vi "ControlProgram6.6_4.vi"() -> ()   [LabVIEW 2016]
uses:
  <vilib>/Utility/miscctls.llb/LVPoint32TypeDef.ctl
  <vilib>/Platform/TimedLoop/XDataNode/timing_clust.ctl
  <vilib>/Platform/TimedLoop/XDataNode/nitl_modes.ctl
  <vilib>/Platform/TimedLoop/XDataNode/wakeup.ctl
  <vilib>/Instr/_visa.llb/Select Event Type.ctl
  <vilib>/vision/Avi1.llb/AviRefnum.ctl
  <vilib>/Utility/error.llb/DialogType.ctl
  <vilib>/DAQmx/write.llb/DAQmx Write (Analog 1D DBL NChan 1Samp).vi
  <vilib>/DAQmx/read.llb/DAQmx Read (Analog 2D DBL NChan NSamp).vi
  <vilib>/Analysis/baseanly.llb/Mean (DBL).vi
  <vilib>/DAQmx/write.llb/DAQmx Write (Digital Bool 1Line 1Point).vi
  <vilib>/DAQmx/create/channels.llb/DAQmx Create Channel (DO-Digital Output).vi
  <vilib>/DAQmx/create/channels.llb/DAQmx Create Channel (AI-Voltage-Basic).vi
  <vilib>/DAQmx/create/channels.llb/DAQmx Create Channel (AO-Voltage-Basic).vi
  <vilib>/DAQmx/configure/timing.llb/DAQmx Timing (Sample Clock).vi
  <vilib>/DAQmx/miscellaneous.llb/DAQmx Fill In Error Info.vi
  <vilib>/Instr/_visa.llb/VISA Configure Serial Port (Instr).vi
  Arnulf--joystick/git(most_up_to_date)/Logitech-joystick/Old Trap/FAST_Global_var.vi
  <vilib>/Utility/inputDevices.llb/mouseAcquire.vi
  <vilib>/Utility/inputDevices.llb/closeMouse.vi
  <vilib>/platform/TimedLoop/XDataNode/XDataNode.xnode
  <vilib>/Platform/TimedLoop/XDataNode/XDNodeRunTimeDep.lvlib
  <resource>/objmgr/daqmx.rc
  <vilib>/Analysis/NI_AALBase.lvlib
panel:
  in  "Save file index":i32
  out "Saving Move":bool
  out "Move time":string
  out "Primary Video Display":T1(plugin-control)
  out "Flush Sample Start Time":u32=2111292881
  out "Sample flush time (s)":dbl=48.0
  in  "Inject Sample":bool
  out "Cal values":T2={"AX alpha"=612.9626061060078, "BX alpha"=549.6584469744151, "AX kappa"=0.3485731373010688, "BX kappa"=0.3853424216291352, "AX offset"=-0.03900484438240665, "BX offset"=-0.11295550662085417, "AY alpha"=582.7562541114835, "BY alpha"=571.1587543790358, "AY kappa"=0.37498408087930674, "BY kappa"=0.36252029651198364, "AY offset"=-0.21125584642206058, "BY offset"=-0.12469077200400738}
  in  "Inject Pump 1":bool
  in  "Inject Pump 2":bool
  in  "Tab Control 2":T3(tab)
  in  "Force FB script":bool
  in  "Got ADig bead":bool
  in  "Move Cap. 2 (ADig Top)":bool
  in  "Dump beads":bool
  in  "Got DNA bead":bool
  in  "Flow on\ncap 2?":bool=TRUE
  in  "Flow on\ncap 1?":bool=TRUE
  in  "Flow on\ndump?":bool=TRUE
  in  "Raster set":i32=1
  in  "Fish After TA?":bool=TRUE
  in  "Delta after tether":dbl=1700.0
  in  "TA Cancel Save?":bool=TRUE
  in  "Min fish\ndelta (nm)":dbl=1425.0 min=0.0 max=5000.0 step=50.0
  in  "Max fish\ndelta (nm)":dbl=1900.0 min=0.0 max=5000.0 step=25.0
  in  "Fish Speed (ms)":i32=5000
  in  "Wait (ms)":i32=1500
  in  "# attempts":dbl=10.0
  in  "Cutoff force (pN)":dbl=4.5
  in  "Raster after\n tether?":bool=TRUE
  out "Tether":bool
  out "Attempt #":i32
  in  "Flow on\nwhile fish?":bool=TRUE
  in  "Flow on\nafter raster?":bool=TRUE
  in  "Offset raster set":i32
  in  "Offset @ Delta (nm)":dbl=1700.0
  in  "Cal @ Delta (nm)":dbl=2500.0
  in  "Cal stage position":i32=3
  out "Cal Final Sampling Rate":dbl=125000.0
  in  "Cal Averaging":i32=1
  in  "Wait before dip (s)":dbl=3.0
  in  "Start dipping after?":bool
  in  "Start trap delta (nm)":dbl=1700.0
  in  "Repeat Dip":bool
  out "Dip #":i32
  in  "Dip attempts":dbl=3.0
  in  "Cancel Rep\n Dip":bool
  out "Return elasped time":i32
  in  "Return duration":dbl=15.0
  in  "Cancel dwell":bool=TRUE
  in  "Pause dwell":bool
  in  "Start/Return position":dbl=3.0
  in  "Dip duration":dbl=15.0
  in  "Dip position":dbl=4.0
  in  "Dip":bool
  out "Dip elasped time":i32
  in  "Stop":bool=TRUE
  in  "?":T4(tab)
  out "FAST X-Y":bool
  out "FAST Z":bool
  in  "Cal time (s)":dbl=5.0
  in  "Save N sets":bool
  in  "N sets":i32=200
  out "Cal sets to save":i32=500
  in  "Reset data stream":bool
  out "Buffer Overflow":bool
  out "Stage moving":bool
  in  "Comment":string
  in  "Raster scan":bool
  out "Saving":bool
  in  "Save cal":bool
  in  "Save Data":bool
  in  "Stop saving":bool
  out "Calibrating":bool
  out "Progress":dbl(slide) scale=0.0..100.0
  in  "Read Cal":bool
  in  "Fish":bool
  in  "Averaging Number":i32=1250
  out "Final Sampling Rate":dbl=100.0
  in  "Trap position (V)":cluster{"X":dbl, "Y":dbl}={"X"=3.9042624789680316, "Y"=0.2}
  in  "Trap delta (nm)":dbl=2500.0 min=0.0 max=5000.0 step=50.0
  in  "Fixed X":dbl=1.1
  in  "Fixed Y":dbl=0.15
  in  "Shutter 1 (B)":bool
  in  "Shutter 2 (A)":bool
  in  "Pulling direction":bool
  out "Raster scanning...":bool
  out "Current file name":path=path "D:/data/160111/160111_006.dat"
  in  "AX alpha":dbl=612.9626061060078 format="%#_3p"
  in  "BX alpha":dbl=549.6584469744151 format="%#_3g"
  in  "AX kappa":dbl=0.3485731373010688 format="%#_3g"
  in  "BX kappa":dbl=0.3853424216291352 format="%#_3g"
  in  "AX offset":dbl=-0.03900484438240665 format="%#_3g"
  in  "BX offset":dbl=-0.11295550662085417 format="%#_3g"
  in  "AY alpha":dbl=582.7562541114835 format="%#_3g"
  in  "BY alpha":dbl=571.1587543790358 format="%#_3g"
  in  "AY kappa":dbl=0.37498408087930674 format="%#_3g"
  in  "BY kappa":dbl=0.36252029651198364 format="%#_3g"
  in  "AY offset":dbl=-0.21125584642206058 format="%#_3g"
  in  "BY offset":dbl=-0.12469077200400738 format="%#_3g"
  out "Buffer status":u8(slide) scale=0.0..100.0
  in  "Target":bool
  in  "Set Current\nPos to (0,0,0)":bool
  in  "dump spot":string="Dump beads spot"
  in  "up flow spot":string="Upper flow spot"
  in  "low flow spot":string="Lower flow spot"
  in  "up cap":string="Upper capillary (ADig beads)"
  in  "bottom cap":string="Lower capillary (DNA beads)"
  in  "Move to Position 5":bool
  in  "Set Position 5":bool
  in  "Saved stage positions":dbl[][](array[numeric])=[[1.0, 0.0, 0.0, 0.0], [2.0, -0.13716, -3.21132, 0.01436], [3.0, 0.45, -0.73974, 0.005], [4.0, 0.45, -2.1978, 0.005], [5.0, 0.45, -2.63158, -0.02256]]
  in  "Set Position 2":bool
  in  "Move to Position 2":bool
  in  "Set Position 1":bool
  in  "Move to Position 1":bool
  in  "Set Position 4":bool
  in  "Move to Position 4":bool
  in  "Set Position 3":bool
  in  "Move to Position 3":bool
  out "Stage error":errorcluster
  in  "Clear Volume":bool
  out "Sample Flush Meter":u8(slide) scale=0.0..100.0
  out "Flushing Sample":bool
  in  "Flush Sample":bool
  in  "Normal \nRate (ul/hr)  3":dbl=100.0
  in  "Normal \nVolume (ul) 3":dbl=250.0
  in  "Normal \nVolume (ul) 2":dbl
  in  "Normal \nRate (ul/hr)":dbl
  in  "Normal \nVolume (ul)":dbl
  in  "Flush\nRate (ul/min)":dbl
  in  "Flush\nVolume (ul)":dbl
  in  "Flush \nRate (ul/min)  2":dbl
  in  "Flush Pump 2":bool
  in  "Flush\nVolume (ul)  2":dbl
  in  "Flush Pump 1":bool
  in  "Normal \nRate (ul/hr)  2":dbl
  in  "Write Wait":i32=1000
  in  "Flush \nRate (ul/min)  3":dbl=100.0
  in  "Flush\nVolume (ul)  3":dbl=80.0
  out "error out":errorcluster
  in  "Use Mouse to Move Trap?":bool
  in  "Pause Mouse/Mirror Connection":bool
  out "Reference Voltage":cluster{dbl, dbl}={0.0, -0.0}
  out "Saved voltage":cluster{dbl, dbl}={5.766666666666665, 1.45}
  out "Real Coordinates":cluster{"Horizontal":i32, "Vertical":i32}={"Horizontal"=897, "Vertical"=-1271}
  out "CoordinatesMousePressed":T5
  in  "Force Feedback 2":bool
  in  "Offset 2":cluster{"Off Y":dbl, "Off X":dbl}={"Off Y"=1.5, "Off X"=0.17}
  in  "Setpoint voltage 2":cluster{"SP Y":dbl, "SP X":dbl}={"SP Y"=0.6, "SP X"=0.0}
  out "Sum error":dbl(knob) scale=-0.2..0.2
  out "Trap sep":waveform(dbl)[](graph)=[{"t0"=timestamp(4.489999999999949 s since 1904-01-01), "dt"=0.002, "Y"=[-1157.7639781743756, -1157.678951177374, -1157.7582331070425, -1157.7490409992681, -1157.8995617642552], "attributes"=variant("NI_ChannelName"=variant(string "T2 X"))}, {"t0"=timestamp(4.489999999999949 s since 1904-01-01), "dt"=0.002, "Y"=[-909.0775466981794, -909.1316439023619, -909.1322956759037, -909.1570630705896, -909.1264297140281], "attributes"=variant("NI_ChannelName"=variant(string "T2 Y"))}]
  in  "Set reading to\nsetpoint 1":bool
  in  "Offset Y (nm)":dbl format="%0.2f"
  in  "Offset X (nm)":dbl format="%0.2f"
  in  "Remove offsets":bool
  in  "Force Feedback 1":bool
  out "Feedback Output \nVoltage 2":cluster{dbl, dbl} {"?" format="%#_4g"; "?" format="%#_4g"}
  in  "Offset 1":cluster{"Off Y":dbl, "Off X":dbl}={"Off Y"=1.5, "Off X"=0.17}
  in  "Setpoint voltage 1":cluster{"SP Y":dbl, "SP X":dbl}={"SP Y"=0.6, "SP X"=0.0}
  in  "Feedback const":T6={"Ki_B_Y"=0.5, "Ki_B_X"=0.0, "Kp Y"=1.0, "Kp X"=0.0}
  out "Mean Trap Pos X 2 (nm)":dbl=-1157.769953044463 format="%0.2f"
  out "Mean Trp Pos Y 2 (nm)":dbl=-909.1249958122125 format="%0.2f"
  out "T2 X RMS (A)":dbl=0.7168002469275427 format="%0.2f"
  out "T2 Y RMS (A)":dbl=0.25997187037503383 format="%0.2f"
  in  "Set reading to\nsetpoint 2":bool
  in  "Scan range (nm)":dbl=425.0
  in  "Scan speed (nm/s)":dbl=100.0 min=0.0 max=100.0
  in  "Step size (nm)":dbl=1.0
  in  "Save scans":bool=TRUE
  in  "# scans":i32=1
  in  "Load param":bool
  in  "Scan Parameters":T7(array[cluster])
  in  "Trap delta\nafter (nm)":dbl=1550.0
  in  "Stop raster":bool
  out "Scan range (V)":dbl=0.47672462142456534
  out "Scan steps (mirror)":u64=425
  out "Scan increment (V)":dbl=0.0011217049915872126
  out "Time per step (ms)":dbl=10.0
  out "Total raster time (s)":dbl=8.5
  out "N sets to be saved":dbl=850.0
  in  "Zoom Factor":sgl=7.0
  in  "Center Point":cluster{"X":i32, "Y":i32}={"X"=335, "Y"=271}
  in  "Intensity Upper":dbl=88.0
  in  "Intensity Lower":dbl=66.0
  out "Window Size":cluster{"Height":i32, "Width":i32}
  in  "Image Index":dbl=1.0 min=1.0
  in  "Save Image":bool
  in  "Averaging":bool
  in  "Reset Averaging":bool
  in  "Save Video":bool
  in  "New Video File":bool
  in  "Video Index":dbl=1.0 min=1.0 step=1.0
  in  "Video Capture Rate (Hz)":dbl=30.0
  in  "Initial Window Size":cluster{"Width":i32, "Height":i32}={"Width"=884, "Height"=619}
  in  "Initial Window Position":cluster{"X Position":i32, "Y Position":i32}={"X Position"=796, "Y Position"=4}
  out "Window Position":cluster{"X Position":i32, "Y Position":i32}={"X Position"=40, "Y Position"=40}
  out "Path Out":path
  in  "Target coordinates":cluster{"X1":dbl, "Y1":dbl, "X2":dbl, "Y2":dbl}={"X1"=328.0, "Y1"=274.0, "X2"=368.0, "Y2"=314.0}
  in  "# Samples/channel (in)":i32=40000 format="%.2f"
  out "Buffer size\n(Samples/channel)":u32=511
  out "DAQ rate\n(Samples/s)":dbl=125000.0 format="%#_6p"
  out "# Samples/channel":i32=1250
  out "# Samples/channel/s":dbl=100.0
  out "AvailSampPerChan":u32=9
  out "Data update period (s/set)":dbl=0.01 format="%#_6p"
  out "AvailSampPerChan 2":u32=110
  in  "PC samp per channel":i32=1000
  in  "Sampling Rate":dbl=125000.0 format="%0.0p"
  in  "DAQ Rate2":dbl=1000000.0 format="%#_6p"
  out "Data period (s)":dbl=8e-06 format="%#_6p"
  in  "Save user params":bool
  in  "User":string(combo)
  in  "Load user params":bool
  in  "Tether break\nforce (pN)":dbl=1.0
  in  "Path":path=path "E:/Data"
  out "Mirror task":refnum<k21>
  in  "Conv X (nm/V)":dbl=891.5
  in  "Conv Y (nm/V)":dbl=505.7
  in  "Min value Y":dbl format="%.1g"
  in  "Max value Y":dbl=10.0 format="%.1f"
  in  "Min value X":dbl format="%0.1f"
  in  "Max value X":dbl=10.0 format="%.1f"
  in  "HWP1":string="Half waveplate 1: differential trap power"
  in  "HWP0":string="Half waveplate 0: total trap power"
  in  "Move 1":bool
  in  "\"Degrees\" 1":dbl
  in  "Move 0":bool
  in  "\"Degrees\" 0":dbl
  in  "Y command":enum16{"Fish", "Dump", "Got ADig", "Got DNA"}(ring)
  in  "B command":enum16{"Got DNA", "Got ADig", "Dump", "Fish"}(ring)
  in  "A command":enum16{"Got ADig", "Dump", "Fish", "Got DNA"}(ring)
  in  "X command":enum16{"Dump", "Fish", "Got ADig", "Got DNA"}(ring)
  out "Logitech":bool
  out "START":bool
  out "BACK":bool
  out "Right stick button":bool
  out "Left Y":i8(slide) scale=-128.0..127.0
  out "Left X":i8(slide) scale=-128.0..127.0
  out "Right Y":i8(slide) scale=-128.0..127.0
  out "Right X":i8(slide) scale=-128.0..127.0
  out "X":bool
  out "Y":bool
  out "A":bool
  out "B":bool
  out "RB":bool
  out "LB":bool
  out "R":bool
  out "L":bool
  out "D":bool
  out "U":bool
  out "Left stick button":bool
  out "FAST Z":bool
  out "FAST X-Y":bool
  in  "XY Speed Definitions":T8={"Slow X velocity input"="0.05", "Slow Y velocity input"="0.05", "Fast1 X velocity input"="0.1", "Fast1 Y velocity input"="0.1", "Fast2 X velocity input"="0.2", "Fast2 Y velocity input"="0.2"}
  in  "Z Speed Definitions":cluster{"Slow Z":string, "Fast Z":string}={"Slow Z"="0.025", "Fast Z"="0.05"}
  in  "Z Wait time":string="120"
  in  "X-Y Wait time":string="125"
  in  "USB port":refnum<visa-resource-name>="USB0::0x046D::0xC21D::CC66247B::RAW"
  out "Deflection":T5
  in  "Sampling Rate":dbl=125000.0 format="%0.2f"
  in  "Averaging Number":i32=12500
  in  "DAQ Rate":dbl=1000000.0
  out "Final Sampling Rate":dbl
  in  "Tab Control":T9(tab)
  in  "Downsamp\nfact":dbl=250.0
  out "Bead sep":waveform(dbl)[](graph)=[{"t0"=timestamp(4.489999999999949 s since 1904-01-01), "dt"=0.002, "Y"=[8093.963535945606, 8103.1617772716045, 8385.72390184118, 8245.733099167523, 8154.925676756515], "attributes"=variant("NI_ChannelName"=variant(string "T2"))}, {"t0"=timestamp(4.489999999999949 s since 1904-01-01), "dt"=0.002, "Y"=[1717.924930434114, 1628.723007842151, 1787.6888378897193, 1598.475730715916, 1776.2517588078954], "attributes"=variant("NI_ChannelName"=variant(string "T1"))}]
  out "Force (pN)":waveform(dbl)[](graph)=[{"t0"=timestamp(4.489999999999949 s since 1904-01-01), "dt"=0.002, "Y"=[2821.5994183803123, 2824.8226375853515, 2923.3663028678166, 2874.5254578927593, 2842.869034836209], "attributes"=variant("NI_ChannelName"=variant(string "T2"))}, {"t0"=timestamp(4.489999999999949 s since 1904-01-01), "dt"=0.002, "Y"=[623.5850847499229, 591.0680427774053, 648.761979867749, 579.944408346982, 644.7436619059413], "attributes"=variant("NI_ChannelName"=variant(string "T1"))}]
  out "Mean force (pN)":dbl=1737.5286029210451 format="%0.2f"
  out "Force noise (pN)":dbl=26.83032703631318 format="%0.2f"
  out "Mean Bead Sep\n(nm)":dbl=4949.257225667222 format="%0.2f"
  out "Bead Sep Noise\n(A)":dbl=757.8078481959694 format="%0.2f"
  out "PSD 2":cluster{dbl[], dbl[]}(graph)
  out "PSD 1":cluster{dbl[], dbl[]}(graph)
  out "PSD 1 Sum":dbl(slide) scale=0.0..10.0
  out "PSD 2 Sum":dbl(slide) scale=0.0..10.0
  in  "Start":bool
  out "All signals 2":waveform(dbl)[](graph)=[{"t0"=timestamp(4.489999999999949 s since 1904-01-01), "dt"=0.002, "Y"=[0.0010396217068286443, 0.0010666908927528754, 0.001103298744846499, 0.0010651440823993424, 0.0010656596859401936], "attributes"=variant("NI_ChannelName"=variant(string "A y"))}, {"t0"=timestamp(4.489999999999949 s since 1904-01-01), "dt"=0.002, "Y"=[0.02000680227246931, 0.020097032918054827, 0.02003412926844257, 0.020136734401221615, 0.020087494249822452], "attributes"=variant("NI_ChannelName"=variant(string "A x"))}, {"t0"=timestamp(4.489999999999949 s since 1904-01-01), "dt"=0.002, "Y"=[-0.0014958587831537804, -0.0015046240440107857, -0.0014930229638311983, -0.001533240041751485, -0.0015262793936602433], "attributes"=variant("NI_ChannelName"=variant(string "B y"))}, {"t0"=timestamp(4.489999999999949 s since 1904-01-01), "dt"=0.002, "Y"=[0.0002901198559372817, 0.0002731049385577592, 0.00026511308349727467, 0.0002517073909711183, 0.0002916666665966012], "attributes"=variant("NI_ChannelName"=variant(string "B x"))}, {"t0"=timestamp(4.489999999999949 s since 1904-01-01), "dt"=0.002, "Y"=[-0.001511556786147372, -0.0015167122027053212, -0.0014612914746018214, -0.0014935128282145193, -0.0015064013696263116], "attributes"=variant("NI_ChannelName"=variant(string "A sum"))}, {"t0"=timestamp(4.489999999999949 s since 1904-01-01), "dt"=0.002, "Y"=[-0.0005242945138364382, -0.0005565158674093218, -0.000501095139248956, -0.0005771375336978897, -0.0005165613890095197], "attributes"=variant("NI_ChannelName"=variant(string "B sum"))}, {"t0"=timestamp(4.489999999999949 s since 1904-01-01), "dt"=0.002, "Y"=[0.0013303666019343777, 0.0014257418088905328, 0.0013368108726387405, 0.0013471217058124534, 0.0011782818123890176], "attributes"=variant("NI_ChannelName"=variant(string "Trap x"))}, {"t0"=timestamp(4.489999999999949 s since 1904-01-01), "dt"=0.002, "Y"=[0.0023382505474007294, 0.002231275652833831, 0.002229986798687363, 0.0021810103409340116, 0.002241586486003531], "attributes"=variant("NI_ChannelName"=variant(string "Trap y"))}]
  out "All signals":waveform(dbl)[](graph)=[{"t0"=timestamp(4.489999999999949 s since 1904-01-01), "dt"=0.002, "Y"=[0.0010396217068286443, 0.0010666908927528754, 0.001103298744846499, 0.0010651440823993424, 0.0010656596859401936], "attributes"=variant("NI_ChannelName"=variant(string "A y"))}, {"t0"=timestamp(4.489999999999949 s since 1904-01-01), "dt"=0.002, "Y"=[0.02000680227246931, 0.020097032918054827, 0.02003412926844257, 0.020136734401221615, 0.020087494249822452], "attributes"=variant("NI_ChannelName"=variant(string "A x"))}, {"t0"=timestamp(4.489999999999949 s since 1904-01-01), "dt"=0.002, "Y"=[-0.0014958587831537804, -0.0015046240440107857, -0.0014930229638311983, -0.001533240041751485, -0.0015262793936602433], "attributes"=variant("NI_ChannelName"=variant(string "B y"))}, {"t0"=timestamp(4.489999999999949 s since 1904-01-01), "dt"=0.002, "Y"=[0.0002901198559372817, 0.0002731049385577592, 0.00026511308349727467, 0.0002517073909711183, 0.0002916666665966012], "attributes"=variant("NI_ChannelName"=variant(string "B x"))}, {"t0"=timestamp(4.489999999999949 s since 1904-01-01), "dt"=0.002, "Y"=[-0.001511556786147372, -0.0015167122027053212, -0.0014612914746018214, -0.0014935128282145193, -0.0015064013696263116], "attributes"=variant("NI_ChannelName"=variant(string "A sum"))}, {"t0"=timestamp(4.489999999999949 s since 1904-01-01), "dt"=0.002, "Y"=[-0.0005242945138364382, -0.0005565158674093218, -0.000501095139248956, -0.0005771375336978897, -0.0005165613890095197], "attributes"=variant("NI_ChannelName"=variant(string "B sum"))}, {"t0"=timestamp(4.489999999999949 s since 1904-01-01), "dt"=0.002, "Y"=[0.0013303666019343777, 0.0014257418088905328, 0.0013368108726387405, 0.0013471217058124534, 0.0011782818123890176], "attributes"=variant("NI_ChannelName"=variant(string "Trap x"))}, {"t0"=timestamp(4.489999999999949 s since 1904-01-01), "dt"=0.002, "Y"=[0.0023382505474007294, 0.002231275652833831, 0.002229986798687363, 0.0021810103409340116, 0.002241586486003531], "attributes"=variant("NI_ChannelName"=variant(string "Trap y"))}]
  out "Chart Freq (Hz)":dbl=500.0
  # "Bead Calibration"
  # "Y"
  # "X"
  # "Pump #1 Controls"
  # "Pump #2 Controls"
  # "Sample Pump Controls"
  # "Retract the pumps manually. Change it back to INFUSE when you're done. Suck it up, don't whine."
  # "Shutter 1 (B)"
  # "Move to Lower Cap"
  # "Inject Sample"
  # "Move to Upper Cap"
  # "Shutter 2 (A)"
  # "Select the Joystick input:"
  # "Overflow happens when >40 commands\nsent in 5 seconds. Then 4 consecutive beeps."
  # "Try increasing wait time to reduce 'following error threshold exceeded' occurances."
  # "Left stick controls Z axis.\nRight on stick: neg Z-dir\nUp on stick: neg Z-dir"
  # "Toggles FAST Z"
  # "Toggles FAST X-Y"
  # "The default Newport max velocity is 0.4"
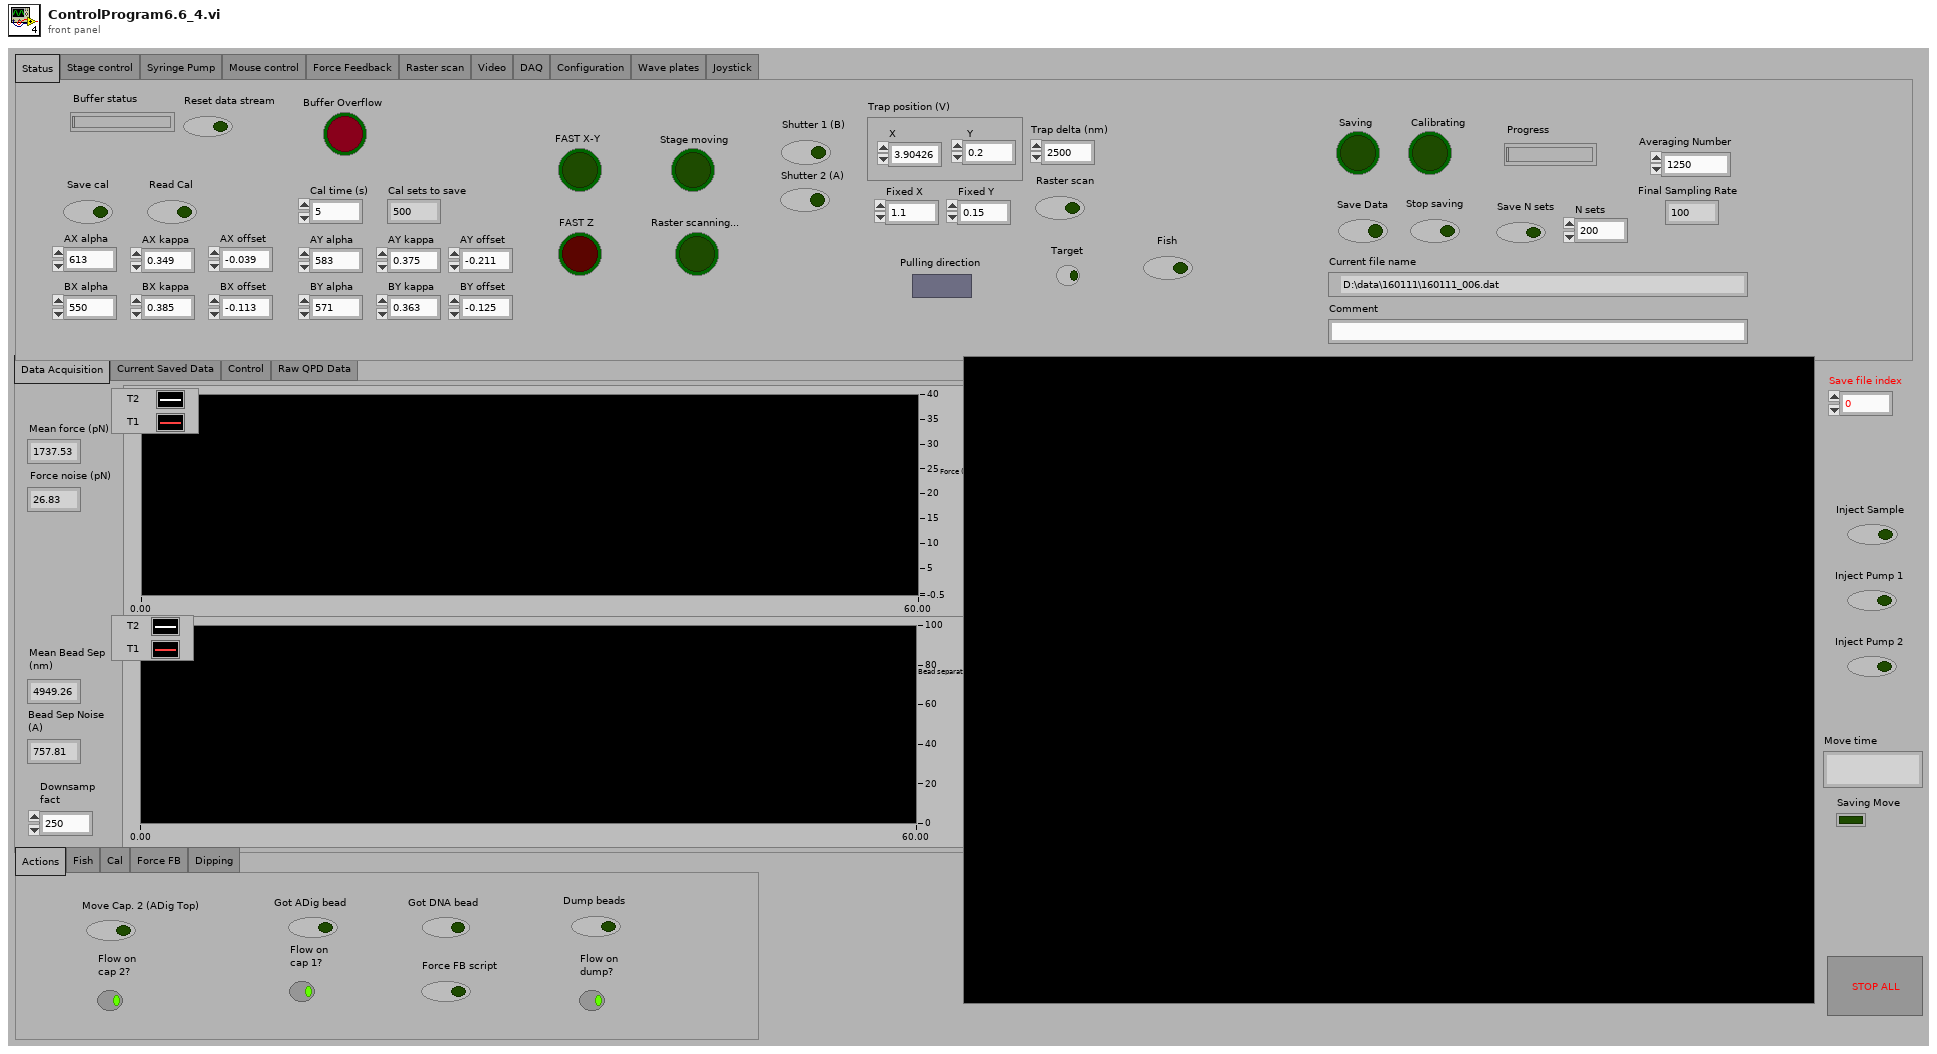
[diagram p1: front panel]
types:
  T1 = typedef "IMAQ Image.ctl" = refnum<image>
  T2 = cluster{"AX alpha":dbl, "BX alpha":dbl, "AX kappa":dbl, "BX kappa":dbl, "AX offset":dbl, "BX offset":dbl, "AY alpha":dbl, "BY alpha":dbl, "AY kappa":dbl, "BY kappa":dbl, "AY offset":dbl, "BY offset":dbl}
  T3 = enum32{"Actions", "Fish", "Cal", "Force FB", "Dipping"}
  T4 = enum32{"Status", "Stage control", "Syringe Pump", "Mouse control", "Force Feedback", "Raster scan", "Video", "DAQ", "Configuration", "Wave plates", "Joystick"}
  T5 = typedef "LVPoint32TypeDef.ctl" = cluster{"Horizontal":i32, "Vertical":i32}
  T6 = cluster{"Ki_B_Y":dbl, "Ki_B_X":dbl, "Kp Y":dbl, "Kp X":dbl}
  T7 = cluster{"Label":string, "Scan range 1":dbl, "Step size 1":dbl, "Scan speed 1":i32, "# scans 2":i32}[]
  T8 = cluster{"Slow X velocity input":string, "Slow Y velocity input":string, "Fast1 X velocity input":string, "Fast1 Y velocity input":string, "Fast2 X velocity input":string, "Fast2 Y velocity input":string}
  T9 = enum32{"Data Acquisition", "Current Saved Data", "Control", "Raw QPD Data"}
  T10 = typedef "Select Event Type.ctl" = u32
  T11 = enum32{"setting", "request", "request control", "info", "statistics", "system settings", "I/O sub system", "HRT control", "camera descriptions", "device specific data", "event sub system settings", "event sub system results", "image memory manager"}
  T12 = typedef "AviRefnum.ctl" = refnum<k1>
  T13 = typedef "XDNodeRunTimeDep.lvlib/timing_clust.ctl" = cluster{"Expected End [f-1]":u64, "Actual End [f-1]":u64, "Finished Late? [f-1]":bool, "Expected End [i-1]":u64, "Actual End [i-1]":u64, "Finished Late? [i-1]":bool, "Expected Start [i]":u64, "Actual Start [i]":u64, "Expected Start [f]":u64, "Actual Start [f]":u64, "Source Name":string, "Structure Name":string, "Period":i64, "Deadline":i64, "Offset":i64, "Start":i64, "Priority":i32, "Timeout":i32, "Mode":T14, "Wakeup Reason":T15, "Error":errorcluster, "Source Type":string, "Secondary Source Type":string, "Global End Time":u64, "Global Start Time":u64, "Frame Duration":u64, "Iteration Duration":u64, "Assigned CPU":i32, "I/O Scan Engine Mode":u32}
  T14 = typedef "XDNodeRunTimeDep.lvlib/nitl_modes.ctl" = enum32{"No Change", "Process missed periods, maintain original phase", "Discard missed periods, maintain original phase", "Process missed periods, ignore original phase", "Discard missed periods, ignore original phase"}
  T15 = typedef "XDNodeRunTimeDep.lvlib/wakeup.ctl" = enum32{"Normal", "Aborted", "Asynchronous wakeup", "Timing source error", "Timed loop error", "Timeout"}
  T16 = typedef "Image Type" = u32
  T17 = typedef "imagedata.ctl" = cluster{"image type":i32, "image depth":i32, "image":u8[], "mask":u8[], "colors":u32[], "Rectangle":cluster{"left":i16, "top":i16, "right":i16, "bottom":i16}}
  T18 = enum16{"open", "replace", "create", "open or create", "replace or create", "replace or create with confirmation"}
  T19 = enum16{"big-endian, network order", "native, host order", "little-endian"}
  T20 = cluster{string, string, string, string, string, string, string, string}
  T21 = cluster{"LB":bool, "RB":bool, "BACK":bool, "Logitech":bool, "START":bool}
  T22 = cluster{"Right X":i8, "Right Y":i8, "Left X":i8, "Left Y":i8}
  T23 = enum32{"Status", "Stage control", "Syringe Pump", "Mouse control", "Force Feedback", "Raster scan", "Video", "DAQ", "Configuration", "Wave plates"}
  T24 = typedef "DialogType.ctl" = u16
  T25 = cluster{"button 1":bool, "button 2":bool, "button 3":bool, "button 4":bool}
  T26 = cluster{"[0]":dbl, "[1]":dbl, "[2]":dbl, "[3]":dbl, "[4]":dbl, "[5]":dbl, "[6]":dbl, "[7]":dbl, "[8]":dbl, "[9]":dbl, "[10]":dbl, "[11]":dbl}
  T27 = cluster{"Label":string, "Scan range 1":dbl, "Step size 1":dbl, "Scan speed 1":i32, "# scans 2":i32}
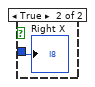
[diagram p5: hidden frame]
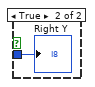
[diagram p6: hidden frame]
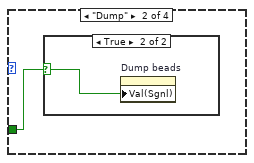
[diagram p10: hidden frame]
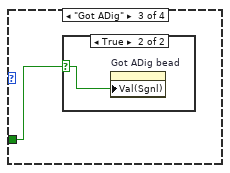
[diagram p12: hidden frame]
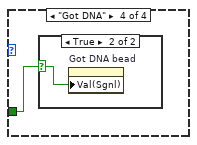
[diagram p14: hidden frame]
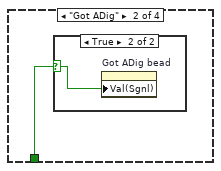
[diagram p17: hidden frame]
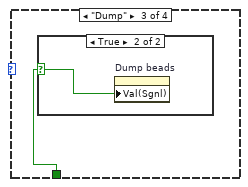
[diagram p19: hidden frame]
diagram:
  w10 = T10 1073684535 items=["Service Request"=1073684491, "Trigger"=3221168138, "Clear"=1073684493, "VXI Signal"=1073684512, "VXI/VME Interrupt"=3221168161, "VXI/VME Sysfail"=1073684509, "VXI/VME Sysreset"=1073684510, "GPIB CIC"=1073684498, "GPIB Talk"=1073684499, "GPIB Listen"=1073684500, "PXI Interrupt"=1073684514, "Serial Break"=1073684515, "Serial TermChar"=1073684516, "Serial CTS"=1073684521, "Serial DSR"=1073684522, "Serial DCD"=1073684524, "Serial RI"=1073684526, "Serial Character"=1073684533, "USB Interrupt"=1073684535, "All Enabled"=1073709055] ("Event Type")
  w49 = 10.0 ("Minimum Value")
  w50 = -10.0 ("Minimum Value")
  w52 = -2.0 ("Minimum Value")
  w53 = 2.0 ("Maximum Value")
  w78 = 10123 items=["Finite Samples"=10178, "Continuous Samples"=10123] ("sample mode")
  w98 = tag "Dev1/port2/line1"  # Shutter 2
  w101 = tag "Dev1/port1/line4"  # Shutter 1
  # "Open the RAW resource"
  # "Enable USB Interrupt Event"
  # "Create channels for movable mirror"
  # "Create channels for detectors"
  n1 = call-poly <vilib>:"DAQmx Create Virtual Channel.vi"("maximum value"=w53, "minimum value"=w52, "physical channels"=tag "Dev1/ai0" ("Physical Channel")) -> ("task out"=w54:refnum<k21>, "error out"=w77:errorcluster)  [unwired: 11 in]
  n2 = call-poly <vilib>:"DAQmx Create Virtual Channel.vi"("task in"=w54, "maximum value"=w53, "minimum value"=w52, "physical channels"=tag "Dev1/ai1", "error in"=w77) -> ("task out"=w75:refnum<k21>, "error out"=w74:errorcluster)  [unwired: 9 in]
  n3 = call-poly <vilib>:"DAQmx Create Virtual Channel.vi"("task in"=w75, "maximum value"=w53, "minimum value"=w52, "physical channels"=tag "Dev1/ai2", "error in"=w74) -> ("task out"=w66:refnum<k21>, "error out"=w65:errorcluster)  [unwired: 9 in]
  n4 = call-poly <vilib>:"DAQmx Create Virtual Channel.vi"("task in"=w66, "maximum value"=w53, "minimum value"=w52, "physical channels"=tag "Dev1/ai3" ("Physical Channel"), "error in"=w65) -> ("task out"=w51:refnum<k21>, "error out"=w71:errorcluster)  [unwired: 9 in]
  n5 = call-poly <vilib>:"DAQmx Create Virtual Channel.vi"("task in"=w51, "maximum value"=w49, "minimum value"=w50, "physical channels"=tag "Dev1/ai4", "error in"=w71) -> ("task out"=w69:refnum<k21>, "error out"=w68:errorcluster)  [unwired: 9 in]
  n6 = call-poly <vilib>:"DAQmx Create Virtual Channel.vi"("task in"=w69, "maximum value"=w49, "minimum value"=w50, "physical channels"=tag "Dev1/ai5", "error in"=w68) -> ("task out"=w64:refnum<k21>, "error out"=w63:errorcluster)  [unwired: 9 in]
  n7 = call-poly <vilib>:"DAQmx Create Virtual Channel.vi"("task in"=w64, "maximum value"=w49, "minimum value"=w50, "physical channels"=tag "Dev1/ai6", "error in"=w63) -> ("task out"=w58:refnum<k21>, "error out"=w56:errorcluster)  [unwired: 9 in]
  n8 = call-poly <vilib>:"DAQmx Create Virtual Channel.vi"("task in"=w58, "maximum value"=w49, "minimum value"=w50, "physical channels"=tag "Dev1/ai7", "error in"=w56) -> ("task out"=w57:refnum<k21>, "error out"=w55:errorcluster)  [unwired: 9 in]
  n9 = call-poly <vilib>:"DAQmx Timing.vi"("task/channels in"=w57, "sample mode"=w78, "samples per channel"="PC samp per channel", "rate"="Sampling Rate", "error in"=w55) -> ("task out"=w61:refnum<k21>, "error out"=w60:errorcluster)  [unwired: 9 in]
  n10 = call-poly <vilib>:"DAQmx Create Virtual Channel.vi"("maximum value"="Max value Y", "minimum value"="Min value Y", "physical channels"=tag "Dev1/ao1" ("Trap X Axis")) -> ("task out"=w46:refnum<k21>, "error out"=w48:errorcluster)  [unwired: 11 in]
  n11 = property class="DAQmx Timing"(reference=w61, error in=w60, "More:AI Convert:Rate"="DAQ Rate2") -> (reference out=w19:refnum<k21>, error out=w18:errorcluster, "SampClk.Rate"=→"DAQ rate\n(Samples/s)":dbl)
  n12 = call-poly <vilib>:"DAQmx Create Virtual Channel.vi"("task in"=w46, "maximum value"="Max value X", "minimum value"="Min value X", "physical channels"=tag "Dev1/ao0" ("Trap Y Axis"), "error in"=w48) -> ("task out"=w37:refnum<k21>, "error out"=w36:errorcluster)  [unwired: 9 in]
  "Mirror task" <- w37
  n13 = property class="DAQmx Buffer"(reference=w19, error in=w18) -> (reference out=w16:refnum<k21>, error out=w15:errorcluster, "Input.OnbrdBufSize"=→"Buffer size\n(Samples/channel)":u32)
  n14 = call <vilib>:"DAQmx Start Task.vi"("task/channels in"=w16, "error in"=w15) -> ("task out"=w38:refnum<k21>)  [unwired: 12 in, 1 out]
  n15 = flat-sequence "Video" {
    tunnel: [w114] -> w13
    tunnel: w13 -> [w155]
    frame #0 {
      n16 = while {
        stop <- w107 continue-if-true
        n17 = call "Close Video Capture.vi"() -> ("error code OUT"=w109:i32)
        n18 = Equal?(x=w109, y=0) -> (x = y?=w107:bool)
      }
      n19 = local write "Stop"(FALSE ("Stop All")) -> ()
    }
    frame #1 {
      n20 = call "DMR_Init.vi"() -> ()  [unwired: 3 out]
    }
    frame #2 {
      # "Setting the destination format to Mono8 makes sure that the image can be displayed in the intensity plot."
      n21 = call "DMR_GetDevice.vi"("search string IN"="DE514724602") -> ("device handle OUT"=w132:i32)  [unwired: 4 in, 2 out]
      n22 = call "DMR_OpenDevice.vi"("device handle IN"=w132) -> ("driver handle OUT"=w115:i32)  [unwired: 4 out]
      n23 = call "DMR_FindList.vi"("flags IN"=u32 0 ("flags"), "list name IN"="" ("String"), "list type IN"=T11."camera descriptions", "driver handle IN"=w115) -> ("list handle OUT"=w118:i32)  [unwired: 2 out]
      n24 = call "DMR_FindList.vi"("flags IN"=u32 0 ("flags"), "list name IN"="Base", "list type IN"=T11."setting", "driver handle IN"=w115) -> ("list handle OUT"=w116:i32)  [unwired: 2 out]
      n25 = call "OBJ_GetHandle.vi"("object name IN"="VideoStandard", "list handle IN"=w118) -> ("object handle OUT"=w112:i32)  [unwired: 3 out]
      n26 = call "OBJ_GetHandle.vi"("object name IN"="PixelFormat", "list handle IN"=w116) -> ("object handle OUT"=w126:i32)  [unwired: 3 out]
      n27 = call "OBJ_SetS.vi"("value index IN"=0, "value IN"="NTSC M", "object handle IN"=w112) -> ()  [unwired: 2 out]
      n28 = call "OBJ_SetS.vi"("value index IN"=0, "value IN"="Mono8" ("value"), "object handle IN"=w126) -> ()  [unwired: 2 out]
      n29 = call "OBJ_GetHandle.vi"("object name IN"="VideoChannel", "list handle IN"=w116) -> ("object handle OUT"=w122:i32)  [unwired: 3 out]
      n30 = while {
        tunnel: [w137] -> w114
        tunnel: w115 -> [w134]
        stop <- w135 continue-if-true
        n31 = call "DMR_ImageRequestSingle.vi"("request control IN"=0, "driver handle IN"=w134) -> ("error code OUT"=w136:i32, "driver handle OUT"=w137:i32)  [unwired: 2 out]
        n32 = Equal To 0?(x=w136) -> (x = 0?=w135:bool)
      }
      n33 = call "OBJ_SetI.vi"("value index IN"=0, "value IN"=0 ("Video channel"), "object handle IN"=w122) -> ()  [unwired: 2 out]
    }
    frame #3 {
      w143 = T16 0 items=["Grayscale (U8)", "Grayscale (I16)", "Grayscale (SGL)", "Complex (CSG)", "RGB (U32)", "HSL (U32)", "RGB (U64)"] ("Image Type")
      w151 = T16 0 items=["Grayscale (U8)", "Grayscale (I16)", "Grayscale (SGL)", "Complex (CSG)", "RGB (U32)", "HSL (U32)", "RGB (U64)"] ("Image Type")
      n34 = for "Create Greyscale map" {
        N: 256 -> [_]
        tunnel: [w157] -> w140 mode=indexing
        workers-P: _ -> [_]
        i -> [w160]
        n35 = To Unsigned Byte Integer(number=w160) -> (unsigned 8bit integer=w156:u8)
        n36 = Join Numbers(hi=w156, lo=w156) -> ((hi.lo)=w159:u16)
        n37 = Join Numbers(hi=w156, lo=w156) -> ((hi.lo)=w158:u16)
        n38 = Join Numbers(hi=w159, lo=w158) -> ((hi.lo)=w157:u32)
      }
      n39 = call "IMAQ Create"("Image Name"="Scaled video", "Image Type"=w143) -> ("New Image"=w142:T1)  [unwired: 2 in, 2 out]
      n40 = call "IMAQ Create"("Image Name"="Main video", "Image Type"=w151) -> ("New Image"=w152:T1)  [unwired: 2 in, 2 out]
      n41 = node-c288(0 ("Processor")) -> (w150:T13)  [unwired: 3 out]
      n42 = Initialize Array(u32 0 ("Window Number (0...15)"), 480 ("dimension size"), 640 ("dimension size")) -> (w145:u32[][])
      n43 = timed-loop {
        tunnel: w155 -> [w177]
        tunnel: [w176] -> w154
        tunnel: w152 -> [w175]
        timing: w150 -> [_]
        timing-out: [_] -> w149
        tunnel: w145 -> [w164]
        tunnel: w142 -> [w162]
        tunnel: w140 -> [w161]
        stop <- w163 stop-if-true
        # "This block performs the \nactual image capture."
        n44 = node-c288() -> ()  [unwired: 2 out]
        n45 = local read "Stop"() -> (w163:bool)
        n46 = Reciprocal(x="Video Capture Rate (Hz)") -> (1/x=w167:dbl)
        n47 = Multiply(x=w167, y=1000.0) -> (x*y=w165:dbl)
        n48 = call "DMR_ImageRequestWaitFor.vi"("queue number IN"=0, "timeout(ms) IN"=500, "driver handle IN"=w177) -> ("error code OUT"=w181:i32, "request number OUT"=w178:i32, "driver handle OUT"=w179:i32)
        n49 = feedback #1(T12 refnum ("Avi Refnum")) -> (w169:T12)
        n50 = case shown="True" "New Video File" {
          tunnel: [T12 refnum ("Avi Refnum") w198] -> w171
          tunnel: [FALSE TRUE] -> w172
          tunnel: w169 -> [_ w194]
          frame False {
          }
          frame True {
            n51 = call "Create new save file.vi"("Ext"=".avi" ("string"), "Index In"="Video Index") -> ("Path Out"=w190:path, "Index Out"=w191:dbl)  [unwired: 1 in]
            "Path Out" <- w190
            n52 = Not Equal?(x=w194, y=T12 refnum ("Avi Refnum")) -> (x != y?=w195:bool)
            n53 = Increment(x=w191) -> (x+1=w200:dbl)
            n54 = case shown="True" w195 {
              tunnel: w194 -> [_ w201]
              frame False {
              }
              frame True {
                n55 = call "IMAQ AVI Close"("Avi Refnum"=w201) -> ()  [unwired: 1 in, 10 out]
              }
            }
            n56 = local write "Video Index"(w200) -> ()
            n57 = call "IMAQ AVI Create"("Frames Per Second"=u32 30, "AVI Path"=w190) -> ("Avi Refnum"=w198:T12)  [unwired: 5 in, 4 out]
          }
        }
        n58 = Equal To 0?(x=w181) -> (x = 0?=w180:bool)
        n59 = Select(t=w171, s=w172, f=w169) -> (s? t:f=w170:T12)
        n60 = feedback-in #1(w170) -> ()
        n61 = case shown="True" w180 {
          tunnel: w179 -> [w202 w229]
          tunnel: w178 -> [_ w228]
          tunnel: [w202 w225] -> w176
          tunnel: w175 -> [_ w206]
          tunnel: w164 -> [_ w213]
          tunnel: w170 -> [_ w211]
          tunnel: w162 -> [_ w207]
          tunnel: w161 -> [_ w208]
          frame False {
          }
          frame True {
            w219 = u32 0 ("X-offset IN")
            n62 = call "DMR_GetImageRequestBufferData.vi"("driver handle IN"=w229, "request number IN"=w228) -> ("width OUT"=w218:i32, "height OUT"=w217:i32, "driver handle OUT"=w224:i32, "request number OUT"=w223:i32, "bytes per pixel OUT"=w220:i32)  [unwired: 13 out]
            n63 = call "DMR_GetImageRequestBufferImageData.vi"("driver handle IN"=w224, "request number IN"=w223, "bytes per pixel IN"=w220, "X-offset IN"=w219, "Y-offset IN"=w219, "height IN"=w217, "width IN"=w218) -> ("driver handle OUT"=w222:u32, "request number OUT"=w221:u32, "image OUT"=w214:u32[][])  [unwired: 10 out]
            n64 = call "DMR_ImageRequestUnlock.vi"("request number IN"=w221, "driver handle IN"=w222) -> ("driver handle OUT"=w227:i32)  [unwired: 1 in, 2 out]
            n65 = case shown="False" "Averaging" {
              tunnel: w214 -> [w270 w275]
              tunnel: [w270 w274] -> w210
              tunnel: w213 -> [_ w272]
              frame False {
              }
              frame True {
                (unwired) 1
                w280 = 1
                n66 = feedback #2(w272) -> (w271:u32[][])
                n67 = Add(x=w275, y=w271) -> (x+y=w276:u32[][])
                n68 = Select(t=w272, s="Reset Averaging", f=w276) -> (s? t:f=w278:u32[][])
                n69 = feedback-in #2(w278) -> ()
                n70 = feedback #3(w280) -> (w273:i32)
                n71 = Divide(x=w276, y=w273) -> (x/y=w277:dbl[][])
                n72 = Increment(x=w273) -> (x+1=w281:i32)
                n73 = To Unsigned Long Integer(number=w277) -> (unsigned 32bit integer=w274:u32[][])
                n74 = Select(t=w280, s="Reset Averaging", f=w281) -> (s? t:f=w279:i32)
                n75 = feedback-in #3(w279) -> ()
              }
            }
            n76 = call "DMR_ImageRequestSingle.vi"("request control IN"=0, "driver handle IN"=w227) -> ("driver handle OUT"=w225:i32)  [unwired: 3 out]
            n77 = disable-structure shown="Disabled" {
              disable-tunnel: w210 -> [w247 _]
              disable-tunnel: w207 -> [w246 _]
              frame Disabled {
                n78 = To Double Precision Float(number=w247) -> (double precision float=w245:dbl[][])
                n79 = In Range and Coerce(upper limit="Intensity Upper", x=w245, lower limit="Intensity Lower") -> (coerced(x)=w244:dbl[][])  [unwired: 1 out]
                n80 = Subtract(x="Intensity Upper", y="Intensity Lower") -> (x-y=w241:dbl)
                n81 = Subtract(x=w244, y="Intensity Lower") -> (x-y=w242:dbl[][])
                n82 = Divide(x=w242, y=w241) -> (x/y=w243:dbl[][])
                n83 = Multiply(x=255.0, y=w243) -> (x*y=w239:dbl[][])
                n84 = To Unsigned Byte Integer(number=w239) -> (unsigned 8bit integer=w248:u8[][])
                n85 = call "IMAQ ArrayToImage"("Image Pixels (U8)"=w248, "Image"=w246) -> ("Image Out"=w235:T1)  [unwired: 4 in, 5 out]
                n86 = First Call?() -> (First Call?: T/F=w236:bool)
                n87 = case shown="True" w236 {
                  tunnel: w235 -> [w249 w260]
                  frame False {
                    n88 = flat-sequence {
                      tunnel: w249 -> [w255]
                      frame #0 {
                        w252 = FALSE ("Get/Set Status? (Set)")
                        w251 = 0 ("Window Number (0...15)")
                        n89 = call "IMAQ WindSize"("Get/Set Status? (Set)"=w252, "Window Number"=w251) -> ("Width & Height out"=→"Window Size":cluster{"Width":i32, "Height":i32})  [unwired: 4 in, 2 out]
                        n90 = call "IMAQ WindMove"("Window Number (0...15)"=w251, "Get/Set Status? (Set)"=w252) -> ("Coordinates (screen)"=→"Window Position":cluster{"X Position":i32, "Y Position":i32})  [unwired: 3 in, 1 out]
                        n91 = call "IMAQ WindDraw"("Resize to Image Size? (Y)"=FALSE, "Window Number (0...15)"=w251, "Image"=w255) -> ()  [unwired: 7 in, 2 out]
                      }
                      frame #1 {
                        n92 = call "IMAQ WindZoom 2"("Center Point"="Center Point", "Zoom to Fit? (False)"=FALSE, "Zoom Factor"="Zoom Factor") -> ()  [unwired: 5 in, 4 out]
                      }
                    }
                  }
                  frame True {
                    n93 = flat-sequence {
                      tunnel: w260 -> [w263]
                      tunnel: [w261] -> w259
                      tunnel: w259 -> [w265]
                      frame #0 {
                        w262 = TRUE ("Resize to Image Size? (Y)")
                        w261 = 0 ("Window Number (0...15)")
                        n94 = call "IMAQ WindNonTearing"("Window Number"=w261, "NonTearing? (True)"=w262) -> ()  [unwired: 8 in, 2 out]
                        n95 = call "IMAQ WindDraw"("Resize to Image Size? (Y)"=w262, "Window Number (0...15)"=w261, "Image"=w263) -> ()  [unwired: 7 in, 2 out]
                      }
                      frame #1 {
                        n96 = call "IMAQ WindSize"("Scrollbars? (N)"=FALSE, "Width & Height"="Initial Window Size", "Window Number"=w265) -> ()  [unwired: 3 in, 3 out]
                        n97 = call "IMAQ WindMove"("Window Number (0...15)"=w265, "Coordinates (screen)"="Initial Window Position") -> ()  [unwired: 3 in, 2 out]
                      }
                    }
                  }
                }
              }
              frame Enabled {
              }
            }
            n98 = To Unsigned Byte Integer(number=w210) -> (unsigned 8bit integer=w209:u8[][])
            n99 = call "IMAQ ArrayToImage"("Image Pixels (U8)"=w209, "Image"=w206) -> ("Image Out"=w204:T1)  [unwired: 4 in, 5 out]
            n100 = case shown="True" "Save Video" {
              tunnel: w211 -> [_ w269]
              tunnel: w204 -> [_ w268]
              frame False {
              }
              frame True {
                n101 = call "IMAQ AVI Write Frame"("Image"=w268, "Avi Refnum"=w269) -> ()  [unwired: 2 in, 8 out]
              }
            }
            n102 = case shown="False" "Save Image" {
              tunnel: w209 -> [_ w284]
              tunnel: w208 -> [_ w283]
              frame False {
              }
              frame True {
                n103 = call <vilib>:"Flatten Pixmap.vi"("colors"=w283, "8-bit pixmap"=w284) -> ("image data"=w290:T17)  [unwired: 4 in, 5 out]
                n104 = call "Create new save file.vi"("Insert"="video_frame_" ("string"), "Ext"=".bmp" ("string"), "Index In"="Image Index") -> ("Path Out"=w286:path, "Index Out"=w291:dbl)
                n105 = Increment(x=w291) -> (x+1=w285:dbl)
                n106 = local write "Image Index"(w285) -> ()
                n107 = call <vilib>:"Write BMP File.vi"("image data"=w290, "path to BMP file"=w286) -> ()  [unwired: 1 in, 9 out]
              }
            }
            n108 = case shown="False" "Target" {
              tunnel: w204 -> [w230 w234]
              tunnel: [w230 w232] -> w203
              frame False {
              }
              frame True {
                n109 = local read "Target coordinates"() -> (w231:cluster{"X1":dbl, "Y1":dbl, "X2":dbl, "Y2":dbl})
                n110 = call "IMAQ Overlay Oval"("Color"=u32 16711680, "Bounding Rectangle"=w231, "Image"=w234) -> ("Image Out"=w232:T1)  [unwired: 7 in, 1 out]
              }
            }
            "Primary Video Display" <- w203
          }
        }
        n111 = node-c288(w165) -> ()  [unwired: 1 out]
      }
      n112 = node-c288(w149) -> ()  [unwired: 1 out]
      n113 = call "DMR_CloseDevice2.vi"("driver handle IN"=w154) -> ()  [unwired: 3 in, 2 out]
    }
    frame #4 {
      n114 = call "DMR_Close.vi"() -> ()  [unwired: 1 out]
    }
  }
  n115 = while {
    tunnel: [w361] -> w84
    tunnel: [w535] -> w85
    tunnel: [w359] -> w83
    tunnel: [w643] -> w80
    tunnel: w38 -> [w346]
    tunnel: w37 -> [w639]
    tunnel: w36 -> [w644]
    stop <- w643 stop-if-true
    w398 = "NI_ChannelName" ("name")
    w302 = "NI_ChannelName" ("name")
    w463 = -1
    # "Negate these value to make Force feedback work in X. 6-14-18 A.T."
    # "BX - AX"
    # "BY - AY"
    # "Scan # counter"
    # "DAQ loop iteration\ncounter (for timing)"
    # "Step counter"
    # "Force feedback"
    # "Raster scan"
    # "Rewire everything"
    # "Invert these because changed\nfrom PSD to QPD"
    # "Trap Y"
    # "Trap X"
    # "Convert to\npN"
    # "Convert to\nnm"
    # "Subtract\noffset"
    # "Normalize by\nsum"
    # "B sum"
    # "BX"
    # "BY"
    # "AX"
    # "AY"
    # "A sum"
    # "Close files when done saving"
    n116 = disable-structure shown="Disabled" {
      frame Disabled {
        n117 = property class="DAQmx Read"() -> ("AvailSampPerChan"=→"AvailSampPerChan 2":u32)  [unwired: 2 in, 2 out]
      }
      frame Enabled {
      }
    }
    n118 = local read "Averaging Number"() -> (w369:i32)
    n119 = local read "Averaging Number"() -> (w371:i32)
    "# Samples/channel" <- w371
    n120 = local read "Sampling Rate"() -> (w642:dbl)
    n121 = call-poly <vilib>:"DAQmx Read.vi"("task/channels in"=w346, "number of samples per channel"=w369, "timeout"=10.0) -> ("task out"=w345:refnum<k21>, "data"=w370:dbl[][], "error out"=w464:errorcluster)  [unwired: 10 in]
    n122 = Unbundle By Name(w464) -> ("status"=w583:bool)
    n123 = Divide(x=w642, y="Cal Averaging") -> (x/y=→"Cal Final Sampling Rate":dbl)
    n124 = Divide(x=w642, y=w371) -> (x/y=→"Final Sampling Rate" →"# Samples/channel/s":dbl)
    n125 = Index Array(array=w370, index (row)=4) -> (element=w460:dbl[])  [unwired: 1 in]
    n126 = disable-structure shown="Disabled" {
      frame Disabled {
        n127 = local read "Buffer size\n(Samples/channel)"() -> (w661:u32)
        n128 = property class="DAQmx Read"() -> ("AvailSampPerChan"=w662:u32)  [unwired: 2 in, 2 out]
        "AvailSampPerChan" <- w662
        n129 = Divide(x=w662, y=w661) -> (x/y=→"Buffer status":dbl)
      }
      frame Enabled {
      }
    }
    n130 = Index Array(array=w370, index (row)=5) -> (element=w459:dbl[])  [unwired: 1 in]
    n131 = Index Array(array=w370, index (row)=0) -> (element=w321:dbl[])  [unwired: 1 in]
    n132 = Index Array(array=w370, index (row)=3) -> (element=w320:dbl[])  [unwired: 1 in]
    n133 = Index Array(array=w370, index (row)=1) -> (element=w319:dbl[])  [unwired: 1 in]
    n134 = Index Array(array=w370, index (row)=7) -> (element=w317:dbl[])  [unwired: 1 in]
    n135 = Index Array(array=w370, index (row)=2) -> (element=w322:dbl[])  [unwired: 1 in]
    n136 = Index Array(array=w370, index (row)=6) -> (element=w318:dbl[])  [unwired: 1 in]
    n137 = case shown="True" w583 {
      frame False {
      }
      frame True {
        n138 = call <vilib>:"Beep.vi"() -> ()  [unwired: 12 in]
        "Buffer Overflow" <- TRUE
      }
    }
    n139 = Divide(x=w322, y=w318) -> (x/y=w316:dbl[])
    n140 = Divide(x=w321, y=w318) -> (x/y=w315:dbl[])
    n141 = Divide(x=w320, y=w317) -> (x/y=w314:dbl[])
    n142 = Divide(x=w319, y=w317) -> (x/y=w313:dbl[])
    n143 = local read "Cal values"() -> (w575:T2)
    n144 = Build Array(w316, w315, w314, w313) -> (w312:dbl[][])
    n145 = Unbundle(w575) -> ("AX alpha"=w563:dbl, "BX alpha"=w559:dbl, "AX kappa"=w555:dbl, "BX kappa"=w551:dbl, "AX offset"=w569:dbl, "BX offset"=w567:dbl, "AY alpha"=w566:dbl, "BY alpha"=w561:dbl, "AY kappa"=w557:dbl, "BY kappa"=w553:dbl, "AY offset"=w573:dbl, "BY offset"=w571:dbl)
    n146 = Multiply(x=w319, y=w463) -> (x*y=w461:dbl[])
    n147 = Multiply(x=w321, y=w463) -> (x*y=w462:dbl[])
    n148 = local write "AX alpha"(w563) -> ()
    n149 = local write "BY offset"(w571) -> ()
    n150 = Build Array(w462, w322, w461, w320, w318, w317, w460, w459) -> (w395:dbl[][])
    n151 = local write "BX alpha"(w559) -> ()
    n152 = case shown="True" "Reset data stream" {
      selector: "Reset data stream" -> [_ w810]
      tunnel: w345 -> [w802 w808]
      tunnel: [w802 w806] -> w535
      tunnel: w464 -> [w801 w805]
      tunnel: [w801 w803] -> _
      frame False {
      }
      frame True {
        n153 = Not(x=w810) -> (.not. x?=w809:bool)
        n154 = call <vilib>:"DAQmx Stop Task.vi"("task/channels in"=w808, "error in"=w805) -> ("task out"=w807:refnum<k21>, "error out"=w804:errorcluster)  [unwired: 12 in]
        n155 = local write "Reset data stream"(w809) -> ()
        n156 = local write "Buffer Overflow"(w809) -> ()
        n157 = call <vilib>:"DAQmx Start Task.vi"("task/channels in"=w807, "error in"=w804) -> ("task out"=w806:refnum<k21>, "error out"=w803:errorcluster)  [unwired: 12 in]
      }
    }
    n158 = call-poly <vilib>:"Mean.vi"("X"=w459) -> ("mean"=w589:dbl)  [unwired: 1 out]
    n159 = local write "AY offset"(w573) -> ()
    n160 = call-poly <vilib>:"Mean.vi"("X"=w460) -> ("mean"=w590:dbl)  [unwired: 1 out]
    n161 = call-poly <vilib>:"Mean.vi"("X"=w322) -> ("mean"=w596:dbl)  [unwired: 1 out]
    n162 = call-poly <vilib>:"Mean.vi"("X"=w320) -> ("mean"=w594:dbl)  [unwired: 1 out]
    n163 = call-poly <vilib>:"Mean.vi"("X"=w318) -> ("mean"=w593:dbl)  [unwired: 1 out]
    n164 = call-poly <vilib>:"Mean.vi"("X"=w317) -> ("mean"=w592:dbl)  [unwired: 1 out]
    n165 = local read "Averaging Number"() -> (w368:i32)
    n166 = local write "BY kappa"(w553) -> ()
    n167 = local write "AX kappa"(w555) -> ()
    n168 = call-poly <vilib>:"Mean.vi"("X"=w461) -> ("mean"=w595:dbl)  [unwired: 1 out]
    n169 = local write "AY kappa"(w557) -> ()
    n170 = call-poly <vilib>:"Mean.vi"("X"=w462) -> ("mean"=w597:dbl)  [unwired: 1 out]
    n171 = local read "DAQ rate\n(Samples/s)"() -> (w374:dbl)
    n172 = Build Array(w590, w589) -> (w588:dbl[])
    n173 = local write "BX kappa"(w551) -> ()
    n174 = local write "BY alpha"(w561) -> ()
    n175 = local write "AX offset"(w569) -> ()
    n176 = local write "BX offset"(w567) -> ()
    n177 = local write "AY alpha"(w566) -> ()
    n178 = Build Array(w597, w596, w595, w594, w593, w592) -> (w586:dbl[])
    n179 = local read "Total raster time (s)"() -> (w342:dbl)
    n180 = Divide(x=w368, y=w374) -> (x/y=w338:dbl)
    "Data update period (s/set)" <- w338
    n181 = Reciprocal(x=w374) -> (1/x=w375:dbl)
    "Data period (s)" <- w375
    n182 = Divide(x=w342, y=w338) -> (x/y=w341:dbl)
    n183 = Divide(x="Cal time (s)", y=w338) -> (x/y=w337:dbl)
    n184 = Divide(x=w597, y=w593) -> (x/y=w627:dbl)
    n185 = Divide(x=w596, y=w593) -> (x/y=w333:dbl)
    n186 = Round Toward -Infinity(1:w341) -> (0:w340:dbl)
    n187 = Divide(x=w595, y=w592) -> (x/y=w634:dbl)
    n188 = Divide(x=w594, y=w592) -> (x/y=w335:dbl)
    n189 = Round Toward -Infinity(1:w337) -> (0:→"Cal sets to save":dbl)
    n190 = local write "N sets to be saved"(w340) -> ()
    n191 = Build Array("Force Feedback 1", "Force Feedback 2") -> (w298:bool[])
    n192 = Boolean Array To Number(Boolean array=w298) -> (number=w297:u32)
    n193 = Negate(x=w333) -> (-x=w332:dbl)
    n194 = Negate(x=w335) -> (-x=w334:dbl)
    n195 = Subtract(x=w627, y="AY offset") -> (x-y=w609:dbl)
    n196 = Subtract(x=w333, y="AX offset") -> (x-y=w610:dbl)
    n197 = Subtract(x=w634, y="BY offset") -> (x-y=w608:dbl)
    n198 = Subtract(x=w335, y="BX offset") -> (x-y=w611:dbl)
    n199 = Subtract(x=w634, y=w627) -> (x-y=w625:dbl)
    n200 = Subtract(x=w334, y=w332) -> (x-y=w626:dbl)
    n201 = feedback #4(0.0) -> (w534:dbl)
    n202 = Multiply(x="Downsamp\nfact", y=w375) -> (x*y=w310:dbl)
    n203 = Multiply(x=w609, y="AY alpha") -> (x*y=w543:dbl)
    n204 = Multiply(x=w610, y="AX alpha") -> (x*y=w541:dbl)
    n205 = Multiply(x=w611, y="BX alpha") -> (x*y=w542:dbl)
    n206 = Multiply(x=w608, y="BY alpha") -> (x*y=w544:dbl)
    n207 = Add(x=w338, y=w534) -> (x+y=w532:dbl)
    n208 = feedback-in #4(w532) -> ()
    n209 = Square(x=w543) -> (x^2=w619:dbl)
    n210 = Square(x=w541) -> (x^2=w620:dbl)
    n211 = Square(x=w544) -> (x^2=w621:dbl)
    n212 = Square(x=w542) -> (x^2=w622:dbl)
    n213 = Bundle(w625, w626) -> (w329:cluster{dbl, dbl})  [unwired: 1 in]
    n214 = case shown="True" "Set reading to\nsetpoint 1" {
      tunnel: w329 -> [_ w799]
      frame False {
      }
      frame True {
        n215 = property on="Setpoint voltage 1" class="Clust (strict)"("Val(Sgnl)"=w799) -> ()  [unwired: 2 in, 2 out]
        n216 = local read "Trap position (V)"() -> (w798:cluster{"X":dbl, "Y":dbl})
        n217 = local write "Set reading to\nsetpoint 1"(FALSE ("Set reading to\nsetpoint")) -> ()
        n218 = Unbundle(w798) -> ("X"=w797:dbl, "Y"=w796:dbl)
        n219 = Bundle("Y"=w796, "X"=w797) -> (w795:cluster{"Y":dbl, "X":dbl})  [unwired: 1 in]
        n220 = property on="Offset 1" class="Clust (strict)"("Val(Sgnl)"=w795) -> ()  [unwired: 2 in, 2 out]
      }
    }
    n221 = Reciprocal(x=w310) -> (1/x=→"Chart Freq (Hz)":dbl)
    n222 = To Time Stamp(1:w532) -> (0:w309:timestamp)
    n223 = Add(x=w619, y=w620) -> (x+y=w623:dbl)
    n224 = Add(x=w621, y=w622) -> (x+y=w633:dbl)
    n225 = Multiply(x=w541, y="AX kappa") -> (x*y=w537:dbl)
    n226 = Bundle("A y", "A x", "B y", "B x", "A sum", "B sum", "Trap x", "Trap y") -> (w523:T20)  [unwired: 1 in]
    n227 = Multiply(x=w542, y="BX kappa") -> (x*y=w538:dbl)
    n228 = Square Root(x=w623) -> (sqrt(x)=w637:dbl)
    n229 = Square Root(x=w633) -> (sqrt(x)=w636:dbl)
    n230 = Multiply(x=w543, y="AY kappa") -> (x*y=w539:dbl)
    n231 = Multiply(x=w544, y="BY kappa") -> (x*y=w540:dbl)
    n232 = Subtract(x=w589, y="Fixed Y") -> (x-y=w624:dbl)
    n233 = Subtract(x=w590, y="Fixed X") -> (x-y=w628:dbl)
    n234 = Cluster To Array(cluster=w523) -> (array=w522:string[])
    n235 = for {
      tunnel: w395 -> [w788] mode=indexing
      tunnel: w310 -> [w787]
      tunnel: "Downsamp\nfact" -> [w793]
      tunnel: [w791] -> w328 mode=indexing
      tunnel: w309 -> [w794]
      tunnel: w522 -> [w790] mode=indexing
      tunnel: w302 -> [w789]
      n236 = call "Downsample 1D array.vi"("Ave N"=w793, "Arrray In"=w788) -> ("Array Out"=w786:dbl[])  [unwired: 9 in]
      n237 = Bundle By Name("Y"=w786, "dt"=w787, "t0"=w794) -> (w792:waveform(dbl))  [unwired: 1 in]
      n238 = Set Waveform Attribute(5:w790, 6:w789, 7:w792) -> (3:w791:waveform(dbl))  [unwired: 1 in, 2 out]
    }
    "All signals" <- w328
    n239 = Square(x=w539) -> (x^2=w612:dbl)
    n240 = Square(x=w537) -> (x^2=w613:dbl)
    n241 = Square(x=w540) -> (x^2=w614:dbl)
    n242 = Square(x=w538) -> (x^2=w615:dbl)
    n243 = Add(x=w612, y=w613) -> (x+y=w616:dbl)
    n244 = Add(x=w614, y=w615) -> (x+y=w617:dbl)
    n245 = Multiply(x=w624, y="Conv Y (nm/V)") -> (x*y=w546:dbl)
    n246 = Multiply(x=w628, y="Conv X (nm/V)") -> (x*y=w547:dbl)
    n247 = feedback #5() -> (w584:cluster{"B_Y":dbl, "B_X":dbl})  [unwired: 1 in]
    n248 = case shown="1" w297 {
      tunnel: [w1143 w1160 w1170] -> w362
      tunnel: [w1142 w1159 w1171] -> w360
      tunnel: w329 -> [_ w1158 w1173]
      tunnel: [cluster{"B_Y":dbl, "B_X":dbl} {"B_Y"=0.0, "B_X"=0.0} ("Sum error past") w1150 w1168] -> w585
      tunnel: w584 -> [_ w1157 w1169]
      tunnel: w639 -> [w1143 w1153 w1161]
      tunnel: w644 -> [w1142 w1152 w1172]
      frame 0, Default {
        # "Force feedback"
      }
      frame 1 {
        n249 = local write "Force Feedback 2"(FALSE) -> ()
        n250 = call "ForceFeedback2.vi"("PSD/Mirror Voltages"=w1158, "Sum error"=w1157, "task/channels in"=w1153, "error in"=w1152, "Desired voltage"="Setpoint voltage 1", "Feedback const"="Feedback const", "offset"="Offset 1") -> ("task out"=w1160:refnum<k21>, "Sum error past"=w1150:cluster{"B_Y":dbl, "B_X":dbl}, "Output Voltage"=→"Feedback Output \nVoltage 2":cluster{dbl, dbl}, "error out"=w1159:errorcluster)  [unwired: 8 in, 1 out]
        n251 = local read "Pulling direction"() -> (w1149:bool)
        n252 = Unbundle(w1150) -> ("B_Y"=w1147:dbl, "B_X"=w1146:dbl)
        n253 = Select(t=w1147, s=w1149, f=w1146) -> (s? t:f=→"Sum error":dbl)
      }
      frame 2 {
        n254 = local write "Force Feedback 1"(FALSE) -> ()
        n255 = local read "Feedback const"() -> (w1162:T6)
        n256 = call "ForceFeedback2.vi"("PSD/Mirror Voltages"=w1173, "Sum error"=w1169, "task/channels in"=w1161, "error in"=w1172, "Desired voltage"="Setpoint voltage 2", "Feedback const"=w1162, "offset"="Offset 2") -> ("task out"=w1170:refnum<k21>, "Sum error past"=w1168:cluster{"B_Y":dbl, "B_X":dbl}, "Output Voltage"=w1163:cluster{dbl, dbl}, "error out"=w1171:errorcluster)  [unwired: 8 in, 1 out]
        n257 = local read "Pulling direction"() -> (w1164:bool)
        n258 = property on="Feedback Output \nVoltage 2" class="Clust (strict)"("Val(Sgnl)"=w1163) -> ()  [unwired: 2 in, 2 out]
        n259 = Unbundle(w1168) -> ("B_Y"=w1167:dbl, "B_X"=w1166:dbl)
        n260 = Select(t=w1167, s=w1164, f=w1166) -> (s? t:f=w1165:dbl)
        n261 = local write "Sum error"(w1165) -> ()
      }
    }
    n262 = feedback-in #5(w585) -> ()
    n263 = Square Root(x=w616) -> (sqrt(x)=w545:dbl)
    n264 = Square Root(x=w617) -> (sqrt(x)=w638:dbl)
    n265 = Add(x=w545, y=w638) -> (x+y=w618:dbl)
    n266 = case shown="True" "Set reading to\nsetpoint 2" {
      tunnel: w329 -> [_ w656]
      frame False {
      }
      frame True {
        n267 = local read "Trap position (V)"() -> (w659:cluster{"X":dbl, "Y":dbl})
        n268 = property on="Setpoint voltage 2" class="Clust (strict)"("Val(Sgnl)"=w656) -> ()  [unwired: 2 in, 2 out]
        n269 = local write "Set reading to\nsetpoint 2"(FALSE) -> ()
        n270 = Unbundle(w659) -> ("X"=w658:dbl, "Y"=w657:dbl)
        n271 = Bundle("Y"=w657, "X"=w658) -> (w655:cluster{"Y":dbl, "X":dbl})  [unwired: 1 in]
        n272 = property on="Offset 2" class="Clust (strict)"("Val(Sgnl)"=w655) -> ()  [unwired: 2 in, 2 out]
      }
    }
    n273 = Build Array(w627, w333, w634, w335, w593, w592, w545, w638, w637, w636, w547, w546) -> ()  [unwired: 1 out]
    n274 = Divide(x=w618, y=2.0) -> (x/y=w582:dbl)
    n275 = Bundle("AX/Asum", "AY/Asum", "BX/Bsum", "BY/Bsum") -> (w304:cluster{string, string, string, string})  [unwired: 1 in]
    n276 = Index Array(array=w328, index=6) -> (element=w400:waveform(dbl))
    n277 = Index Array(array=w328, index=7) -> (element=w402:waveform(dbl))
    n278 = Cluster To Array(cluster=w304) -> (array=w303:string[])
    n279 = for {
      tunnel: w312 -> [w654] mode=indexing
      tunnel: "Downsamp\nfact" -> [w653]
      tunnel: w310 -> [w652]
      tunnel: w309 -> [w650]
      tunnel: w303 -> [w648] mode=indexing
      tunnel: w302 -> [w647]
      tunnel: [w646] -> w301 mode=indexing
      n280 = call "Downsample 1D array.vi"("Ave N"=w653, "Arrray In"=w654) -> ("Array Out"=w651:dbl[])  [unwired: 9 in]
      n281 = Bundle By Name("Y"=w651, "dt"=w652, "t0"=w650) -> (w649:waveform(dbl))  [unwired: 1 in]
      n282 = Set Waveform Attribute(5:w648, 6:w647, 7:w649) -> (3:w646:waveform(dbl))  [unwired: 1 in, 2 out]
    }
    "All signals 2" <- w301
    n283 = local read "Fixed X"() -> (w449:dbl)
    n284 = local read "Fixed Y"() -> (w451:dbl)
    n285 = Unbundle By Name(w400) -> ("Y"=w453:dbl[])
    n286 = Unbundle By Name(w402) -> ("Y"=w452:dbl[])
    n287 = Index Array(array=w328, index=0) -> (element=w407:waveform(dbl))
    n288 = Index Array(array=w328, index=1) -> (element=w519:waveform(dbl))
    n289 = Index Array(array=w328, index=4) -> (element=w513:waveform(dbl))
    n290 = Subtract(x=w453, y=w449) -> (x-y=w450:dbl[])
    n291 = Subtract(x=w452, y=w451) -> (x-y=w447:dbl[])
    n292 = Unbundle By Name(w407) -> ("Y"=w511:dbl[])
    n293 = Unbundle By Name(w519) -> ("Y"=w510:dbl[])
    n294 = Unbundle By Name(w513) -> ("Y"=w509:dbl[])
    n295 = Index Array(array=w328, index=5) -> (element=w512:waveform(dbl))
    n296 = local read "Conv X (nm/V)"() -> (w448:dbl)
    n297 = local read "Conv Y (nm/V)"() -> (w446:dbl)
    n298 = Index Array(array=w328, index=2) -> (element=w323:waveform(dbl))
    n299 = Index Array(array=w328, index=3) -> (element=w516:waveform(dbl))
    n300 = Set Waveform Attribute(5:"T2 X", 6:w398, 7:w400) -> (3:w399:waveform(dbl))  [unwired: 1 in, 2 out]
    n301 = Set Waveform Attribute(5:"T2 Y", 6:w398, 7:w402) -> (3:w401:waveform(dbl))  [unwired: 1 in, 2 out]
    n302 = Unbundle By Name(w512) -> ("Y"=w506:dbl[])
    n303 = Unbundle By Name(w323) -> ("Y"=w508:dbl[])
    n304 = Unbundle By Name(w516) -> ("Y"=w507:dbl[])
    n305 = Divide(x=w511, y=w509) -> (x/y=w327:dbl[])
    n306 = Divide(x=w510, y=w509) -> (x/y=w326:dbl[])
    n307 = local read "AY offset"() -> (w497:dbl)
    n308 = local read "AX offset"() -> (w495:dbl)
    n309 = Multiply(x=w450, y=w448) -> (x*y=w392:dbl[])
    n310 = Multiply(x=w447, y=w446) -> (x*y=w394:dbl[])
    n311 = Divide(x=w507, y=w506) -> (x/y=w324:dbl[])
    n312 = Subtract(x=w326, y=w495) -> (x-y=w498:dbl[])
    n313 = local read "BX offset"() -> (w505:dbl)
    n314 = Subtract(x=w327, y=w497) -> (x-y=w499:dbl[])
    n315 = Divide(x=w508, y=w506) -> (x/y=w325:dbl[])
    n316 = local read "AY alpha"() -> (w496:dbl)
    n317 = local read "AX alpha"() -> (w494:dbl)
    n318 = call-poly <vilib>:"Mean.vi"("X"=w394) -> ("mean"=w429:dbl)  [unwired: 1 out]
    "Mean Trp Pos Y 2 (nm)" <- w429
    n319 = Subtract(x=w325, y=w327) -> (x-y=w419:dbl[])
    n320 = Subtract(x=w324, y=w326) -> (x-y=w418:dbl[])
    n321 = local read "BY offset"() -> (w502:dbl)
    n322 = Subtract(x=w392, y="Offset X (nm)") -> (x-y=w391:dbl[])
    n323 = Subtract(x=w394, y="Offset Y (nm)") -> (x-y=w393:dbl[])
    n324 = Subtract(x=w325, y=w502) -> (x-y=w504:dbl[])
    n325 = Subtract(x=w324, y=w505) -> (x-y=w503:dbl[])
    n326 = Subtract(x=w429, y=w394) -> (x-y=w428:dbl[])
    n327 = call-poly <vilib>:"Mean.vi"("X"=w392) -> ("mean"=w433:dbl)  [unwired: 1 out]
    "Mean Trap Pos X 2 (nm)" <- w433
    n328 = Build Array(w419, w418) -> (w416:dbl[][])
    n329 = Index Array(array=w416, index (row)=0) -> (element=w414:dbl[])  [unwired: 1 in]
    n330 = Index Array(array=w416, index (row)=1) -> (element=w413:dbl[])  [unwired: 1 in]
    n331 = call-poly <vilib>:"Mean.vi"("X"=w414) -> ("mean"=w412:dbl)  [unwired: 1 out]
    n332 = call-poly <vilib>:"Mean.vi"("X"=w413) -> ("mean"=w411:dbl)  [unwired: 1 out]
    n333 = Bundle("mean"=w412, "mean"=w411) -> ()  [unwired: 1 in, 1 out]
    n334 = local read "BX alpha"() -> (w500:dbl)
    n335 = Multiply(x=w499, y=w496) -> (x*y=w487:dbl[])
    n336 = Multiply(x=w498, y=w494) -> (x*y=w486:dbl[])
    n337 = Square(x=w428) -> (x^2=w427:dbl[])
    n338 = Subtract(x=w433, y=w392) -> (x-y=w432:dbl[])
    n339 = Bundle By Name(cluster=w401, "Y"=w393) -> (w444:waveform(dbl))
    n340 = Bundle By Name(cluster=w399, "Y"=w391) -> (w445:waveform(dbl))
    n341 = local read "BY alpha"() -> (w501:dbl)
    n342 = local read "Raster scanning..."() -> (w344:bool)
    n343 = local read "Saving"() -> (w548:bool)
    n344 = local read "Tether"() -> (w549:bool)
    n345 = Square(x=w432) -> (x^2=w431:dbl[])
    n346 = call-poly <vilib>:"Mean.vi"("X"=w427) -> ("mean"=w426:dbl)  [unwired: 1 out]
    n347 = Square(x=w487) -> (x^2=w493:dbl[])
    n348 = Multiply(x=w504, y=w501) -> (x*y=w485:dbl[])
    n349 = Square(x=w486) -> (x^2=w492:dbl[])
    n350 = Multiply(x=w503, y=w500) -> (x*y=w484:dbl[])
    n351 = Less?(x=w582, y="Tether break\nforce (pN)") -> (x < y?=w580:bool)
    n352 = call-poly <vilib>:"Mean.vi"("X"=w431) -> ("mean"=w430:dbl)  [unwired: 1 out]
    n353 = Build Array(w445, w444) -> (w363:waveform(dbl)[])
    "Trap sep" <- w363
    n354 = Square Root(x=w426) -> (sqrt(x)=w425:dbl)
    n355 = Square(x=w485) -> (x^2=w491:dbl[])
    n356 = Square(x=w484) -> (x^2=w490:dbl[])
    n357 = Add(x=w493, y=w492) -> (x+y=w489:dbl[])
    n358 = Square Root(x=w430) -> (sqrt(x)=w423:dbl)
    n359 = Compound Arithmetic op=AND(w548, w549, w580) -> (w579:bool)
    n360 = Multiply(x=w425, y=10) -> (x*y=→"T2 Y RMS (A)":dbl)
    n361 = Square Root(x=w489) -> (sqrt(x)=w387:dbl[])
    n362 = Add(x=w491, y=w490) -> (x+y=w488:dbl[])
    n363 = Set Waveform Attribute(5:"T2", 6:"NI_ChannelName" ("name"), 7:w407) -> (3:w406:waveform(dbl))  [unwired: 1 in, 2 out]
    n364 = Set Waveform Attribute(5:"T1", 6:"NI_ChannelName" ("name"), 7:w323) -> (3:w404:waveform(dbl))  [unwired: 1 in, 2 out]
    n365 = case shown="True" w579 {
      selector: w579 -> [_ w817]
      tunnel: w344 -> [w811 w813]
      tunnel: [w811 w813] -> w343
      frame False {
      }
      frame True {
        n366 = call <vilib>:"Beep.vi"() -> ()  [unwired: 12 in]
        n367 = Not(x=w817) -> (.not. x?=w812:bool)
        n368 = And(x=w813, y="Fish After TA?") -> (x .and. y?=w815:bool)
        n369 = local write "Force Feedback 1"(w812) -> ()
        n370 = local write "Tether"(w812) -> ()
        n371 = case shown="True" w815 {
          selector: w815 -> [_ w818]
          frame False {
          }
          frame True {
            n372 = property on="Fish" class="Bool (strict)"("Val(Sgnl)"=w818) -> ()  [unwired: 2 in, 2 out]
          }
        }
        n373 = local write "Force Feedback 2"(w812) -> ()
        n374 = property on="Stop saving" class="Bool (strict)"("Val(Sgnl)"="TA Cancel Save?") -> ()  [unwired: 2 in, 2 out]
      }
    }
    n375 = Square Root(x=w488) -> (sqrt(x)=w386:dbl[])
    n376 = Multiply(x=w423, y=10) -> (x*y=→"T2 X RMS (A)":dbl)
    n377 = Bundle By Name(cluster=w406, "Y"=w387) -> (w410:waveform(dbl))
    n378 = Bundle By Name(cluster=w404, "Y"=w386) -> (w466:waveform(dbl))
    n379 = Add(x=w387, y=w386) -> (x+y=w385:dbl[])
    n380 = case shown="True" "Remove offsets" {
      selector: "Remove offsets" -> [_ w784]
      frame False {
      }
      frame True {
        n381 = local read "Mean Trp Pos Y 2 (nm)"() -> (w782:dbl)
        n382 = Not(x=w784) -> (.not. x?=w785:bool)
        n383 = local read "Mean Trap Pos X 2 (nm)"() -> (w783:dbl)
        n384 = local write "Remove offsets"(w785) -> ()
        n385 = local write "Offset Y (nm)"(w782) -> ()
        n386 = local write "Offset X (nm)"(w783) -> ()
      }
    }
    n387 = Build Array(w410, w466) -> (→"Bead sep":waveform(dbl)[])
    n388 = local read "AY kappa"() -> (w483:dbl)
    n389 = local read "AX kappa"() -> (w482:dbl)
    n390 = Divide(x=w385, y=2) -> (x/y=w383:dbl[])
    n391 = local read "BX kappa"() -> (w480:dbl)
    n392 = local read "BY kappa"() -> (w481:dbl)
    n393 = call-poly <vilib>:"Mean.vi"("X"=w383) -> ("mean"=w382:dbl)  [unwired: 1 out]
    "Mean Bead Sep\n(nm)" <- w382
    n394 = local read "Calibrating"() -> (w296:bool)
    n395 = Multiply(x=w487, y=w483) -> (x*y=w476:dbl[])
    n396 = Multiply(x=w486, y=w482) -> (x*y=w477:dbl[])
    n397 = Square(x=w476) -> (x^2=w475:dbl[])
    n398 = Square(x=w477) -> (x^2=w474:dbl[])
    n399 = Subtract(x=w383, y=w382) -> (x-y=w381:dbl[])
    n400 = Multiply(x=w485, y=w481) -> (x*y=w478:dbl[])
    n401 = Multiply(x=w484, y=w480) -> (x*y=w479:dbl[])
    n402 = Or(x=w343, y="Raster scan") -> (x .or. y?=w358:bool)
    n403 = Add(x=w475, y=w474) -> (x+y=w471:dbl[])
    n404 = Square(x=w381) -> (x^2=w380:dbl[])
    n405 = Square Root(x=w471) -> (sqrt(x)=w443:dbl[])
    n406 = Square(x=w478) -> (x^2=w473:dbl[])
    n407 = Square(x=w479) -> (x^2=w472:dbl[])
    n408 = call-poly <vilib>:"Mean.vi"("X"=w380) -> ("mean"=w379:dbl)  [unwired: 1 out]
    n409 = Add(x=w473, y=w472) -> (x+y=w470:dbl[])
    n410 = Bundle By Name(cluster=w406, "Y"=w443) -> (w469:waveform(dbl))
    n411 = local read "Saving"() -> (w578:bool)
    n412 = Or(x=w296, y=w578) -> ()  [unwired: 1 out]
    n413 = Square Root(x=w379) -> (sqrt(x)=w378:dbl)
    n414 = Square Root(x=w470) -> (sqrt(x)=w442:dbl[])
    n415 = Multiply(x=10, y=w378) -> (x*y=→"Bead Sep Noise\n(A)":dbl)
    n416 = Bundle By Name(cluster=w404, "Y"=w442) -> (w468:waveform(dbl))
    n417 = Add(x=w443, y=w442) -> (x+y=w441:dbl[])
    n418 = Build Array(w469, w468) -> (→"Force (pN)":waveform(dbl)[])
    n419 = Divide(x=w441, y=2) -> (x/y=w438:dbl[])
    n420 = call-poly <vilib>:"Mean.vi"("X"=w438) -> ("mean"=w439:dbl)  [unwired: 1 out]
    "Mean force (pN)" <- w439
    n421 = Subtract(x=w439, y=w438) -> (x-y=w437:dbl[])
    n422 = Square(x=w437) -> (x^2=w436:dbl[])
    n423 = call-poly <vilib>:"Mean.vi"("X"=w436) -> ("mean"=w435:dbl)  [unwired: 1 out]
    n424 = flat-sequence {
      tunnel: w296 -> [w861]
      tunnel: w578 -> [_]
      tunnel: w296 -> [_]
      tunnel: w578 -> [_]
      tunnel: w395 -> [w848]
      tunnel: [w848] -> w599
      tunnel: w464 -> [w847]
      tunnel: [w847] -> w598
      tunnel: w586 -> [w846]
      tunnel: [w846] -> w591
      tunnel: w588 -> [w845]
      tunnel: [w845] -> w587
      tunnel: [w842] -> w577
      tunnel: [w839] -> w576
      tunnel: [w836] -> w458
      tunnel: [w835] -> w457
      tunnel: [w832] -> w456
      tunnel: w365 -> [w829]
      tunnel: ["Save Data"] -> w364
      tunnel: [w822] -> w331
      tunnel: w599 -> [w1042]
      tunnel: w598 -> [w1041]
      tunnel: w591 -> [_]
      tunnel: w587 -> [_]
      tunnel: w577 -> [w1040]
      tunnel: w576 -> [w1039]
      tunnel: w458 -> [w1038]
      tunnel: w457 -> [w1037]
      tunnel: w456 -> [w1036]
      tunnel: w364 -> [w1035]
      tunnel: w363 -> [w1034]
      tunnel: w331 -> [w1032]
      frame #0 {
        w828 = 0.0
        # "1: old trap\n0: fleezers"
        # "Create files if saving data"
        n425 = local read "Save N sets"() -> (w831:bool)
        n426 = local read "Fixed X"() -> (w827:dbl)
        n427 = local read "Trap position (V)"() -> (w856:cluster{"X":dbl, "Y":dbl})
        n428 = local read "Fixed Y"() -> (w826:dbl)
        n429 = local read "Sampling Rate"() -> (w859:dbl)
        n430 = Or(x=w831, y="Save Data") -> (x .or. y?=w830:bool)
        n431 = Build Array(w830, "Save cal", w829) -> (w850:bool[])
        n432 = Compound Arithmetic op=OR("Save Data", "Save cal", w829) -> (w852:bool)
        n433 = Boolean Array To Number(Boolean array=w850) -> (number=w849:u32)
        n434 = Unbundle(w856) -> ("X"=w825:dbl, "Y"=w824:dbl)
        n435 = Build Array(w825, w824, w827, w826, w828, w828) -> (w855:dbl[])
        n436 = feedback #6(refnum<k0> refnum) -> (w821:refnum<file>)
        n437 = feedback #7(0) -> (w853:i32)
        n438 = feedback #8(refnum<k0> refnum) -> (w843:refnum<file>)
        n439 = feedback #9() -> (w837:dbl)  [unwired: 1 in]
        n440 = feedback #10(FALSE) -> (w833:bool)
        n441 = feedback #11(refnum<k0> refnum) -> (w840:refnum<file>)
        n442 = case shown="True" w852 {
          tunnel: w861 -> [_ _]
          tunnel: 9 -> [_ w907]
          tunnel: w859 -> [_ w906]
          tunnel: 6 -> [_ w905]
          tunnel: 5 -> [_ w904]
          tunnel: w855 -> [_ w903]
          tunnel: [w867 1] -> w836
          tunnel: w853 -> [w868 _]
          tunnel: w849 -> [_ w879]
          tunnel: [w866 w878] -> w842
          tunnel: w843 -> [w866 _]
          tunnel: [w865 w877] -> w839
          tunnel: w840 -> [w865 _]
          tunnel: 1.0 -> [_ w876]
          tunnel: [w864 w875] -> w835
          tunnel: w837 -> [w864 _]
          tunnel: [w863 w874] -> w832
          tunnel: w833 -> [w863 _]
          tunnel: [w862 w869] -> w822
          tunnel: w821 -> [w862 _]
          frame False {
            n443 = Increment(x=w868) -> (x+1=w867:i32)
          }
          frame True {
            w880 = FALSE ("Save Data")
            w885 = FALSE
            w886 = T19."big-endian, network order" ("byte order (0:big-endian, network order)")
            n444 = local write "Save cal"(w880) -> ()
            n445 = local write "Save Data"(w880) -> ()
            n446 = case shown="1, Default" w879 {
              tunnel: w907 -> [w982 w1000 w1031]
              tunnel: w906 -> [w961 w999 w1008]
              tunnel: w905 -> [w981 w997 w1027]
              tunnel: w904 -> [w980 w996 w1026]
              tunnel: w903 -> [w979 w993 w1023]
              tunnel: [w978 w992 w1012] -> w900
              tunnel: [w959 w983 w1003] -> w874
              tunnel: ["Averaging Number" 200 w1010] -> _
              tunnel: w876 -> [w966 w985 w1009]
              tunnel: [w962 w984 w1004] -> w875
              tunnel: [w959 w983 w1002] -> w871
              frame 1, Default {
                w959 = TRUE
                w967 = 0.0
                # "stage x,yz"
                # "Save N number/length of data. e.g. N =200 \nwill give only 200 long data points"
                # "Time trace"
                n447 = Boolean To (0,1)(Boolean=w959) -> (0, 1=w972:i16)
                n448 = local read "Averaging Number"() -> (w977:i32)
                n449 = Increment(x=w972) -> (x+1=w971:i16)
                n450 = Divide(x=w961, y=w977) -> (x/y=w976:dbl)
                n451 = To Double Precision Float(number=w971) -> (double precision float=w970:dbl)
                n452 = Reciprocal(x=w976) -> (1/x=w975:dbl)
                n453 = Reciprocal(x=w961) -> (1/x=w960:dbl)
                n454 = Build Array(w982, w960, w975, w981, w980, 0 ("f")) -> (w974:dbl[])
                n455 = Build Array(w970, w966, w967, w967, w967) -> (w973:dbl[])
                n456 = Build Array (concatenate)(w974, w979, w973) -> (w978:dbl[])
                n457 = Select(t="N sets", s="Save N sets", f=2147483647) -> (s? t:f=w962:i32)
              }
              frame 2 {
                w983 = FALSE
                w988 = 0.0
                # "Calibration file"
                n458 = Reciprocal(x=w999) -> (1/x=w998:dbl)
                n459 = Boolean To (0,1)(Boolean=w983) -> (0, 1=w991:i16)
                n460 = To Double Precision Float(number=w991) -> (double precision float=w990:dbl)
                n461 = Build Array(w1000, w998, w998, w997, w996, 1) -> (w994:dbl[])
                n462 = Build Array(w990, w985, w988, w988, w988) -> (w989:dbl[])
                n463 = Build Array (concatenate)(w994, w993, w989) -> (w992:dbl[])
                n464 = local read "Cal sets to save"() -> (w984:i32)
                "Calibrating" <- TRUE ("Calibrating")
              }
              frame 4 {
                w1001 = FALSE ("Raster scan")
                w1019 = 0.0
                w1003 = TRUE
                # "Not using ncycles"
                # "FX curve"
                n465 = Not(x=w1003) -> (.not. x?=w1002:bool)
                n466 = local read "Averaging Number"() -> (w1030:i32)
                n467 = Boolean To (0,1)(Boolean=w1003) -> (0, 1=w1022:i16)
                n468 = local write "Saving Move"(w1001) -> ()
                n469 = Divide(x=w1008, y=w1030) -> (x/y=w1029:dbl)
                n470 = Increment(x=w1022) -> (x+1=w1021:i16)
                n471 = local write "Raster scan"(w1001) -> ()
                n472 = To Double Precision Float(number=w1021) -> (double precision float=w1020:dbl)
                n473 = Reciprocal(x=w1029) -> (1/x=w1028:dbl)
                n474 = Reciprocal(x=w1008) -> (1/x=w1007:dbl)
                n475 = Build Array(w1020, w1009, w1019, w1019, w1019) -> (w1018:dbl[])
                n476 = Build Array(w1031, w1007, w1028, w1027, w1026, 2) -> (w1024:dbl[])
                n477 = local read "Scan range (V)"() -> (w1005:dbl)
                n478 = local read "Pulling direction"() -> (w1016:bool)
                n479 = local read "Scan steps (mirror)"() -> (w1006:u64)
                n480 = local read "# scans"() -> (w1014:i32)
                n481 = local read "N sets to be saved"() -> (w1004:dbl)
                n482 = Not(x=w1016) -> (.not. x?=w1015:bool)
                n483 = local read "Averaging Number"() -> (w1010:i32)
                n484 = Boolean To (0,1)(Boolean=w1015) -> (0, 1=w1017:i16)
                n485 = Build Array(w1017, w1005, w1006, 0, w1014) -> (w1013:dbl[])
                n486 = Build Array (concatenate)(w1024, w1023, w1018, w1013) -> (w1012:dbl[])
              }
            }
            n487 = call "CreateSaveFile.vi"("Index In"="Save file index", "Ext"=".dat", "Insert"="", "Directory"="Path") -> ("Index Out"=w873:i32, "Path Out"=w870:path)  [unwired: 6 in]
            "Current file name" <- w870
            n488 = case shown="True" w871 {
              tunnel: w870 -> [_ w919]
              tunnel: [refnum<k0> refnum w916] -> w869
              frame False {
              }
              frame True {
                # "SY 190201 \nAdding functionality to get time points of start and stop moves. \nWehn timetrace save data starts save time point"
                n489 = Path To String(path=w919) -> (string=w923:string)
                n490 = Get Date/Time In Seconds() -> (seconds since 1Jan1904=w933:timestamp)
                n491 = String Length(string=w923) -> (length=w920:i32)
                n492 = Subtract(x=w920, y=4) -> (x-y=w922:i32)
                n493 = Format Date/Time String(time format string (%c)="%H:%M:%S%3u", seconds (now)=w933, UTC format=TRUE) -> (date/time string=w917:string)
                n494 = call <vilib>:"Space Constant.vi"() -> ("String"=w911:string)
                n495 = String Subset(string=w923, length (rest)=w922) -> (substring=w924:string)  [unwired: 1 in]
                n496 = Concatenate Strings(w924, "_stagetime.txt" ("string")) -> (w926:string)
                n497 = String To Path(string=w926) -> (path=w927:path)
                n498 = Open/Create/Replace File(file path (use dialog)=w927, operation (0:open)=T18."create", access (0:read/write)=enum16{"read/write", "read-only", "write-only"}."write-only") -> (refnum out=w931:refnum<file>, error out=w930:errorcluster)  [unwired: 3 in, 1 out]
                n499 = Deny Access(4:w930, 7:w931) -> (3:w932:refnum<file>)  [unwired: 1 in, 1 out]
                n500 = Concatenate Strings(w917, w911, "start", "\r\n") -> (w918:string)
                n501 = Write to Text File(file (use dialog)=w932, text=w918) -> (refnum out=w916:refnum<file>)  [unwired: 2 in, 2 out]
                n502 = local write "Move time"(w917) -> ()
                n503 = local read "Raster scanning..."() -> (w914:bool)
                n504 = local read "Calibrating"() -> (w915:bool)
                n505 = Or(x=w915, y=w914) -> (x .or. y?=w913:bool)
                n506 = Not(x=w913) -> (.not. x?=w912:bool)
                n507 = local write "Saving Move"(w912) -> ()
              }
            }
            n508 = Open/Create/Replace File(file path (use dialog)=w870, operation (0:open)=T18."create", access (0:read/write)=enum16{"read/write", "read-only", "write-only"}."write-only") -> (refnum out=w893:refnum<file>, error out=w894:errorcluster)  [unwired: 3 in, 1 out]
            n509 = local write "Save file index"(w873) -> ()
            n510 = Array Size(array=w900) -> (size(s)=w902:i32)
            n511 = case shown="True" w874 {
              tunnel: w870 -> [_ w958]
              tunnel: [refnum<k0> refnum w937] -> w877
              frame False {
              }
              frame True {
                w944 = 0.0
                n512 = Path To String(path=w958) -> (string=w954:string)
                n513 = Build Array(w944, w944, w944, w944, w944, w944, w944, w944) -> (w941:dbl[])
                n514 = String Length(string=w954) -> (length=w957:i32)
                n515 = Array Size(array=w941) -> (size(s)=w943:i32)
                n516 = Subtract(x=w957, y=4) -> (x-y=w955:i32)
                n517 = To Double Precision Float(number=w943) -> (double precision float=w942:dbl)
                n518 = String Subset(string=w954, length (rest)=w955) -> (substring=w953:string)  [unwired: 1 in]
                n519 = Build Array (concatenate)(w942, w941) -> (w940:dbl[])
                n520 = Concatenate Strings(w953, "_pos.dat" ("string")) -> (w951:string)
                n521 = String To Path(string=w951) -> (path=w950:path)
                n522 = Open/Create/Replace File(file path (use dialog)=w950, operation (0:open)=T18."create", access (0:read/write)=enum16{"read/write", "read-only", "write-only"}."write-only") -> (refnum out=w946:refnum<file>, error out=w947:errorcluster)  [unwired: 3 in, 1 out]
                n523 = Deny Access(4:w947, 7:w946) -> (3:w945:refnum<file>)  [unwired: 1 in, 1 out]
                n524 = Write to Binary File(file (use dialog)=w945, data=w940, 5:FALSE ("prepend array or string size? (T)"), 9:T19."big-endian, network order" ("byte order (0:big-endian, network order)")) -> (refnum out=w937:refnum<file>)  [unwired: 2 in, 2 out]
              }
            }
            n525 = Deny Access(4:w894, 7:w893) -> (0:w884:errorcluster, 3:w892:refnum<file>)  [unwired: 1 in]
            n526 = String Length(string="Comment") -> (length=w899:i32)
            n527 = To Double Precision Float(number=w902) -> (double precision float=w901:dbl)
            n528 = To Double Precision Float(number=w899) -> (double precision float=w898:dbl)
            n529 = Build Array (concatenate)(w901, w900, w898) -> (w889:dbl[])
            n530 = Write to Binary File(file (use dialog)=w892, data=w889, error in=w884, 5:w885, 9:w886) -> (refnum out=w888:refnum<file>, error out=w883:errorcluster)  [unwired: 1 in, 1 out]
            n531 = Write to Binary File(file (use dialog)=w888, data="Comment", error in=w883, 5:w885, 9:w886) -> (refnum out=w878:refnum<file>)  [unwired: 1 in, 2 out]
            "Saving" <- TRUE
          }
        }
        n532 = feedback-in #6(w822) -> ()
        n533 = feedback-in #7(w836) -> ()
        n534 = feedback-in #8(w842) -> ()
        n535 = feedback-in #9(w835) -> ()
        n536 = feedback-in #10(w832) -> ()
        n537 = feedback-in #11(w839) -> ()
      }
      frame #1 {
        n538 = local read "Saving"() -> (w1033:bool)
        n539 = case shown="True" w1033 {
          tunnel: w1042 -> [_ w1062]
          tunnel: w1041 -> [_ w1061]
          tunnel: w1040 -> [_ w1060]
          tunnel: w1039 -> [_ w1059]
          tunnel: w1038 -> [_ w1050]
          tunnel: w1037 -> [_ w1051]
          tunnel: w1036 -> [_ w1054]
          tunnel: w1035 -> [_ w1046]
          tunnel: w1034 -> [_ w1045]
          tunnel: w1032 -> [_ w1043]
          frame False {
            (unwired) FALSE ("Calibrating")
          }
          frame True {
            n540 = local read "Stop"() -> (w1057:bool)
            n541 = Less Or Equal?(x=w1050, y=w1051) -> (x <= y?=w1058:bool)
            n542 = Divide(x=w1050, y=w1051) -> (x/y=w1049:dbl)
            n543 = Or(x=w1057, y="Stop saving") -> (x .or. y?=w1044:bool)
            n544 = Multiply(x=100.0, y=w1049) -> (x*y=w1048:dbl)
            n545 = Not(x=w1044) -> (.not. x?=w1056:bool)
            n546 = And(x=w1058, y=w1056) -> (x .and. y?=w1055:bool)
            n547 = case shown="True" w1055 {
              tunnel: w1060 -> [w1067 w1092]
              tunnel: w1061 -> [_ w1091]
              tunnel: w1062 -> [_ w1090]
              tunnel: w1059 -> [w1066 w1089]
              tunnel: w1054 -> [w1063 _]
              tunnel: [0.0 ("Progress") w1088] -> w1053
              tunnel: w1048 -> [_ w1088]
              tunnel: w1046 -> [_ _]
              tunnel: w1045 -> [_ w1087]
              tunnel: w1043 -> [w1064 w1084]
              frame False {
                n548 = flat-sequence {
                  tunnel: w1067 -> [w1072]
                  tunnel: w1066 -> [w1071]
                  tunnel: w1064 -> [w1070]
                  tunnel: w1063 -> [w1069]
                  frame #0 {
                    n549 = local read "Saving Move"() -> (w1068:bool)
                    n550 = case shown="True" w1069 {
                      tunnel: w1071 -> [_ w1082]
                      frame False {
                      }
                      frame True {
                        n551 = Close File(refnum=w1082) -> ()  [unwired: 1 in, 2 out]
                      }
                    }
                    n552 = case shown="True" w1068 {
                      tunnel: w1070 -> [_ w1077]
                      frame False {
                      }
                      frame True {
                        n553 = Get Date/Time In Seconds() -> (seconds since 1Jan1904=w1081:timestamp)
                        n554 = call <vilib>:"Space Constant.vi"() -> ("String"=w1076:string)
                        n555 = Format Date/Time String(time format string (%c)="%H:%M:%S%3u", seconds (now)=w1081, UTC format=TRUE) -> (date/time string=w1074:string)
                        n556 = Concatenate Strings(w1074, w1076, "end") -> (w1073:string)
                        n557 = Write to Text File(file (use dialog)=w1077, text=w1073) -> (refnum out=w1078:refnum<file>)  [unwired: 2 in, 2 out]
                        n558 = Close File(refnum=w1078) -> ()  [unwired: 1 in, 2 out]
                        n559 = local write "Move time"(w1074) -> ()
                      }
                    }
                    n560 = Close File(refnum=w1072) -> ()  [unwired: 1 in, 2 out]
                  }
                  frame #1 {
                    w1083 = FALSE
                    n561 = local write "Saving"(w1083) -> ()
                    n562 = local write "Stop saving"(w1083) -> ()
                    n563 = local write "Saving Move"(w1083) -> ()
                    n564 = local write "Calibrating"(w1083) -> ()
                    n565 = call <vilib>:"Beep.vi"() -> ()  [unwired: 12 in]
                  }
                }
              }
              frame True {
                n566 = local read "Calibrating"() -> (w1086:bool)
                n567 = local read "Saving Move"() -> (w1085:bool)
                n568 = case shown="True" w1086 {
                  tunnel: w1092 -> [w1125 w1141]
                  tunnel: w1091 -> [_ w1140]
                  tunnel: w1090 -> [w1112 w1134]
                  tunnel: w1089 -> [w1111 _]
                  tunnel: w1087 -> [w1103 _]
                  frame False {
                    n569 = local read "Averaging Number"() -> (w1119:i32)
                    n570 = Array Subset(array=w1112, index (row)=0 ("index"), length (row)=6 ("length")) -> (w1108:dbl[][])  [unwired: 2 in]
                    n571 = Array Subset(array=w1112, index (row)=6 ("index"), length (row)=2 ("length")) -> (w1107:dbl[][])  [unwired: 2 in]
                    n572 = Array Size(array=w1107) -> (size(s)=w1118:i32[])
                    n573 = Array Size(array=w1108) -> (size(s)=w1115:i32[])
                    n574 = Index Array(array=w1103, index=0) -> (element=w1100:waveform(dbl))
                    n575 = Index Array(array=w1103, index=1) -> (element=w1099:waveform(dbl))
                    n576 = for {
                      tunnel: w1108 -> [w1129] mode=indexing
                      tunnel: w1119 -> [w1131]
                      tunnel: [w1130] -> w1106 mode=indexing
                      n577 = call "Downsample 1D array.vi"("Ave N"=w1131, "Arrray In"=w1129) -> ("Array Out"=w1130:dbl[])  [unwired: 9 in]
                    }
                    n578 = Unbundle By Name(w1100) -> ()  [unwired: 1 out]
                    n579 = Unbundle By Name(w1099) -> ()  [unwired: 1 out]
                    n580 = Multiply Array Elements(1:w1115) -> (0:w1114:i32)
                    n581 = for {
                      tunnel: w1107 -> [w1128] mode=indexing
                      tunnel: w1119 -> [w1127]
                      tunnel: [w1126] -> w1110 mode=indexing
                      n582 = call "Downsample 1D array.vi"("Ave N"=w1127, "Arrray In"=w1128) -> ("Array Out"=w1126:dbl[])  [unwired: 9 in]
                    }
                    n583 = Multiply Array Elements(1:w1118) -> (0:w1117:i32)
                    n584 = Divide(x=w1114, y=w1119) -> (x/y=w1120:dbl)
                    n585 = Divide(x=w1117, y=w1119) -> (x/y=w1116:dbl)
                    n586 = Transpose 2D Array(2D array=w1106) -> (transposed array=w1105:dbl[][])
                    n587 = Transpose 2D Array(2D array=w1110) -> (transposed array=w1104:dbl[][])
                    n588 = Reshape Array(w1105, w1120) -> (w1109:dbl[])
                    n589 = Reshape Array(w1104, w1116) -> (w1113:dbl[])
                    n590 = call <vilib>:"Write File+ [SGL].vi"("1D array"=w1113, "refnum"=w1111) -> ()  [unwired: 7 in, 3 out]
                    n591 = call <vilib>:"Write File+ [SGL].vi"("1D array"=w1109, "refnum"=w1125) -> ()  [unwired: 7 in, 3 out]
                  }
                  frame True {
                    n592 = Array Subset(array=w1134, index (row)=0 ("index"), length (row)=6 ("length")) -> (w1132:dbl[][])  [unwired: 2 in]
                    n593 = Transpose 2D Array(2D array=w1132) -> (transposed array=w1138:dbl[][])
                    n594 = Array Size(array=w1132) -> (size(s)=w1133:i32[])
                    n595 = Multiply Array Elements(1:w1133) -> (0:w1139:i32)
                    n596 = Reshape Array(w1138, w1139) -> (w1137:dbl[])
                    n597 = call <vilib>:"Write File+ [SGL].vi"("1D array"=w1137, "error in (no error)"=w1140, "refnum"=w1141) -> ()  [unwired: 6 in, 3 out]
                  }
                }
                n598 = case shown="True" w1085 {
                  tunnel: w1084 -> [_ w1093]
                  frame False {
                  }
                  frame True {
                    n599 = event shown="[0] \"Move time\": Value Change" {
                      selector: _ -> [_ _]
                      dyn-events: _ -> [_ _]
                      timeout: 1 -> [_ _]
                      tunnel: w1093 -> [w1098 _]
                      event "Move time": Value Change {
                        n600 = event-data() -> ("NewVal"=w1097:string)  [unwired: 1 in, 5 out]
                        n601 = Concatenate Strings(w1097, "\r\n") -> (w1095:string)
                        n602 = Write to Text File(file (use dialog)=w1098, text=w1095) -> ()  [unwired: 2 in, 3 out]
                      }
                      event Timeout {
                        n603 = event-data() -> ()  [unwired: 1 in, 3 out]
                      }
                    }
                  }
                }
              }
            }
            "Progress" <- w1053
          }
        }
      }
    }
    n604 = Square Root(x=w435) -> (sqrt(x)=→"Force noise (pN)":dbl)
    n605 = local read "Flushing Sample"() -> (w367:bool)
    n606 = case shown="True" w367 {
      frame False {
      }
      frame True {
        n607 = local read "Flush Sample Start Time"() -> (w778:u32)
        n608 = local read "Sample flush time (s)"() -> (w771:dbl)
        n609 = Tick Count (ms)() -> (millisecond timer value=w779:u32)
        n610 = Subtract(x=w779, y=w778) -> (x-y=w769:u32)
        n611 = Multiply(x=u32 1000, y=w771) -> (x*y=w770:dbl)
        n612 = Divide(x=w769, y=w770) -> (x/y=w774:dbl)
        n613 = Greater?(x=w769, y=w770) -> (0:w777:bool)
        n614 = Not(x=w777) -> (.not. x?=w776:bool)
        n615 = Boolean To (0,1)(Boolean=w776) -> (0, 1=w775:i16)
        n616 = Compound Arithmetic op=MULTIPLY(w775, w774, 100.0 ("value")) -> (→"Sample Flush Meter":dbl)
        n617 = case shown="True" w777 {
          frame False {
          }
          frame True {
            w781 = FALSE ("Inject Sample")
            n618 = property on="Clear Volume" class="Bool (strict)"("Val(Sgnl)"=TRUE ("Value (Signaling)")) -> ()  [unwired: 2 in, 2 out]
            n619 = local write "Inject Sample"(w781) -> ()
            n620 = local write "Flushing Sample"(w781) -> ()
          }
        }
      }
    }
    n621 = feedback #12(0) -> (w351:i32)
    n622 = feedback #13(0) -> (w348:i32)
    n623 = feedback #14(0) -> (w353:i32)
    n624 = case shown="True" w358 {
      tunnel: w362 -> [w670 w728]
      tunnel: [w670 w712] -> w361
      tunnel: w360 -> [w669 w727]
      tunnel: [w669 w711] -> w359
      tunnel: "Raster scan" -> [w668 w705]
      tunnel: [w668 w704] -> w356
      tunnel: [0 w703] -> w354
      tunnel: w353 -> [_ w697]
      tunnel: w351 -> [_ w685]
      tunnel: [0 w688] -> w350
      tunnel: w348 -> [_ w694]
      tunnel: [0 w693] -> w347
      frame False {
      }
      frame True {
        # "Reset step counter"
        # "Current position"
        # "Initial values"
        n625 = local read "Conv Y (nm/V)"() -> (w680:dbl)
        n626 = local read "Conv X (nm/V)"() -> (w681:dbl)
        n627 = local read "Trap delta (nm)"() -> (w679:dbl)
        n628 = disable-structure shown="Disabled" {
          frame Disabled {
            n629 = local write "Raster scan"(FALSE ("Raster scan")) -> ()
            n630 = property on="Reset data stream" class="Bool (strict)"("Val(Sgnl)"=TRUE) -> ()  [unwired: 2 in, 2 out]
          }
          frame Enabled {
          }
        }
        n631 = local read "Data update period (s/set)"() -> (w702:dbl)
        n632 = local read "Time per step (ms)"() -> (w699:dbl)
        n633 = Select(t=w680, s="Pulling direction", f=w681) -> (s? t:f=w678:dbl)
        n634 = Divide(x=w679, y=w678) -> (x/y=w677:dbl)
        n635 = local read "Fixed X"() -> (w721:dbl)
        n636 = local read "Fixed Y"() -> (w722:dbl)
        n637 = local read "Fixed X"() -> (w683:dbl)
        n638 = local read "Fixed Y"() -> (w682:dbl)
        n639 = local read "Trap position (V)"() -> (w684:cluster{"X":dbl, "Y":dbl})
        n640 = Select(t=w682, s="Pulling direction", f=w683) -> (s? t:f=w676:dbl)
        n641 = local read "Scan steps (mirror)"() -> (w710:u64)
        n642 = Unbundle(w684) -> ("X"=w674:dbl, "Y"=w675:dbl)
        n643 = Multiply(x=w702, y=1000.0) -> (x*y=w700:dbl)
        n644 = local read "Stop raster"() -> (w717:bool)
        n645 = local read "Stop saving"() -> (w718:bool)
        n646 = Select(t=w721, s="Pulling direction", f=w722) -> (s? t:f=w729:dbl)
        n647 = Add(x=w677, y=w676) -> ()  [unwired: 1 out]
        n648 = local write "Saving Move"(FALSE) -> ()
        n649 = Divide(x=w699, y=w700) -> (x/y=w698:dbl)
        n650 = Quotient & Remainder(x=w697, y=w698) -> (x-y*floor(x/y)=w696:dbl)  [unwired: 1 out]
        n651 = Not(x=w717) -> (.not. x?=w716:bool)
        n652 = Select(t=w675, s="Pulling direction", f=w674) -> (s? t:f=w672:dbl)
        n653 = Not(x=w718) -> (.not. x?=w715:bool)
        n654 = Multiply(x=u64 2, y=w710) -> (x*y=w706:u64)
        n655 = Equal To 0?(x=w696) -> (x = 0?=w695:bool)
        n656 = Less?(x=w685, y=w706) -> (x < y?=w707:bool)
        n657 = Compound Arithmetic op=AND(w707, w716, w715, w695) -> (w708:bool)
        n658 = Not(x=w707) -> (.not. x?=w691:bool)
        n659 = feedback #15() -> (w713:dbl)  [unwired: 1 in]
        n660 = case shown="True" w708 {
          tunnel: w729 -> [_ w764]
          tunnel: w672 -> [_ w746]
          tunnel: w728 -> [w741 w763]
          tunnel: w727 -> [w740 w762]
          tunnel: [w741 w761] -> w712
          tunnel: [w740 w760] -> w711
          tunnel: [w737 w749] -> w714
          tunnel: w685 -> [w738 w744]
          tunnel: w713 -> [w737 w743]
          tunnel: w705 -> [w739 w748]
          tunnel: [w739 w748] -> w704
          tunnel: [w738 w747] -> w689
          frame False {
          }
          frame True {
            # "Go forward or backward?"
            n661 = local read "Scan increment (V)"() -> (w742:dbl)
            n662 = local read "Scan steps (mirror)"() -> (w753:u64)
            n663 = Multiply(x=w742, y=w744) -> (x*y=w745:dbl)
            n664 = Less?(x=w744, y=w753) -> (x < y?=w752:bool)
            n665 = Add(x=w746, y=w745) -> (x+y=w755:dbl)
            n666 = Subtract(x=w743, y=w742) -> (x-y=w754:dbl)
            n667 = Select(t=w755, s=w752, f=w754) -> (s? t:f=w749:dbl)
            n668 = local read "Pulling direction"() -> (w751:bool)
            n669 = Build Array(w749, w764) -> (w758:dbl[])
            n670 = Build Array(w764, w749) -> (w757:dbl[])
            n671 = Select(t=w758, s=w751, f=w757) -> (s? t:f=w756:dbl[])
            n672 = call-poly <vilib>:"DAQmx Write.vi"("task/channels in"=w763, "auto start"=TRUE, "data"=w756, "error in"=w762) -> ("task out"=w761:refnum<k21>, "error out"=w760:errorcluster)  [unwired: 9 in, 1 out]
            n673 = Increment(x=w744) -> (x+1=w747:i32)
            "Raster scanning..." <- TRUE ("Raster scanning...")
          }
        }
        n674 = feedback-in #15(w714) -> ()
        n675 = case shown="True" w691 {
          tunnel: w694 -> [w734 w736]
          tunnel: [w734 w735] -> w693
          frame False {
          }
          frame True {
            n676 = Increment(x=w736) -> (x+1=w735:i32)
          }
        }
        n677 = local read "# scans"() -> (w692:i32)
        n678 = local read "Stop saving"() -> (w720:bool)
        n679 = Greater Or Equal?(x=w693, y=w692) -> (x >= y?=w686:bool)
        n680 = Not(x=w686) -> (.not. x?=w687:bool)
        n681 = And(x=w691, y=w687) -> (x .and. y?=w690:bool)
        n682 = Compound Arithmetic op=OR(w686, "Stop raster", w720) -> (w723:bool)
        n683 = case shown="True" w723 {
          frame False {
          }
          frame True {
            n684 = flat-sequence {
              frame #0 {
                n685 = Wait (ms)(milliseconds to wait=u32 300) -> ()  [unwired: 1 out]
              }
              frame #1 {
                n686 = property on="Trap delta (nm)" class="DigNum (strict)"("Val(Sgnl)"="Trap delta\nafter (nm)") -> ()  [unwired: 2 in, 2 out]
              }
            }
          }
        }
        n687 = And(x="Flow on\nafter raster?", y=w723) -> (x .and. y?=w724:bool)
        n688 = case shown="True" w724 {
          frame False {
          }
          frame True {
            n689 = property on="Inject Sample" class="Bool (strict)"("Val(Sgnl)"=TRUE ("Value (Signaling)")) -> ()  [unwired: 2 in, 2 out]
          }
        }
        n690 = case shown="True" w690 {
          tunnel: w689 -> [w732 _]
          tunnel: [w732 0] -> w688
          frame False {
          }
          frame True {
          }
        }
        n691 = Not(x=w723) -> (.not. x?=w726:bool)
        n692 = local write "Raster scanning..."(w726) -> ()
        n693 = Increment(x=w697) -> (x+1=w703:i32)
      }
    }
    n694 = And(x="Save scans", y=w356) -> (x .and. y?=w365:bool)
    n695 = feedback-in #12(w350) -> ()
    n696 = feedback-in #13(w347) -> ()
    n697 = feedback-in #14(w354) -> ()
    n698 = local read "Stop"() -> (w643:bool)
  }
  n699 = local write "Progress"(u8 0 ("Progress")) -> ()
  n700 = local write "Calibrating"(FALSE ("Calibrating")) -> ()
  n701 = VISA Open(VISA resource name="USB port") -> (VISA resource name=w12:refnum<visa-resource-name>, error out=w11:errorcluster)  [unwired: 1 in, 3 out]
  n702 = VISA Enable Event(8:w11, 10:w10, 11:w12) -> (0:w7:errorcluster, 3:w8:refnum<visa-resource-name>)  [unwired: 1 out]
  n703 = call-poly "VISA Configure Serial Port"("VISA resource name"=refnum<visa-resource-name> "COM5", "baud rate (9600)"=u32 19200) -> ("VISA resource name out"=w2:refnum<visa-resource-name>, "error out"=w28:errorcluster)  [unwired: 12 in]
  n704 = while {
    tunnel: w2 -> [w1223]
    shift-right: [w1219] -> w4
    shift-left: w8 -> [w1222]
    shift-right: [w1220] -> w3
    shift-left: w7 -> [w1221]
    stop <- w1218 stop-if-true
    n705 = global read "FAST_Global_var.vi" "FAST L"() -> (→"FAST Z" →"FAST Z":bool)
    n706 = global read "FAST_Global_var.vi" "FAST R"() -> (→"FAST X-Y" →"FAST X-Y":bool)
    n707 = call "LogitechSubVi.vi"("USB port"=w1222, "VISA resource name in 2 (for the Newport)"=w1223, "error in (no error)"=w1221, "X-Y Wait time"="X-Y Wait time", "Z Wait time"="Z Wait time", "XY Speed Definitions"="XY Speed Definitions", "Z Speed Definitions"="Z Speed Definitions") -> ("Right stick button"=→"Right stick button":bool, "Left stick button"=→"Left stick button":bool, "USB port out"=w1219:refnum<visa-resource-name>, "error out"=w1220:errorcluster, "A B X Y"=w1212:cluster{"A":bool, "B":bool, "X":bool, "Y":bool}, "LB RB"=w1211:T21, "U D L R"=w1217:cluster{"U":bool, "D":bool, "L":bool, "R":bool}, "Sticks"=w1210:T22)  [unwired: 5 in]
    n708 = Unbundle By Name(w1211) -> ("LB"=w1205:bool, "RB"=w1204:bool, "BACK"=w1178:bool, "Logitech"=w1177:bool, "START"=w1179:bool)
    "RB" <- w1204
    "LB" <- w1205
    "BACK" <- w1178
    "START" <- w1179
    "Logitech" <- w1177
    n709 = case shown="True" w1179 {
      selector: w1179 -> [_ w1227]
      frame False {
      }
      frame True {
        n710 = property on="Move to Position 2" class="Bool (strict)"("Val(Sgnl)"=w1227) -> ()  [unwired: 2 in, 2 out]
      }
    }
    n711 = case shown="True" w1177 {
      frame False {
      }
      frame True {
        n712 = local read "Inject Sample"() -> (w1224:bool)
        n713 = Not(x=w1224) -> (.not. x?=w1225:bool)
        n714 = property on="Inject Sample" class="Bool (strict)"("Val(Sgnl)"=w1225) -> ()  [unwired: 2 in, 2 out]
      }
    }
    n715 = case shown="True" w1205 {
      frame False {
      }
      frame True {
        n716 = local read "Shutter 1 (B)"() -> (w1271:bool)
        n717 = Not(x=w1271) -> (.not. x?=w1270:bool)
        n718 = property on="Shutter 1 (B)" class="Bool (strict)"("Val(Sgnl)"=w1270) -> ()  [unwired: 2 in, 2 out]
      }
    }
    n719 = case shown="True" w1178 {
      selector: w1178 -> [_ w1226]
      frame False {
      }
      frame True {
        n720 = property on="Move to Position 1" class="Bool (strict)"("Val(Sgnl)"=w1226) -> ()  [unwired: 2 in, 2 out]
      }
    }
    n721 = Unbundle By Name(w1217) -> ("U"=→"U":bool, "D"=→"D":bool, "L"=→"L":bool, "R"=→"R":bool)
    n722 = Unbundle By Name(w1212) -> ("A"=w1200:bool, "B"=w1198:bool, "X"=w1203:bool, "Y"=w1196:bool)
    "A" <- w1200
    "B" <- w1198
    "X" <- w1203
    "Y" <- w1196
    n723 = case shown="\"Fish\"" "A command" {
      tunnel: w1200 -> [w1250 w1252 w1254 w1257]
      frame "Got ADig", Default {
        n724 = case shown="True" w1250 {
          selector: w1250 -> [_ w1251]
          frame False {
          }
          frame True {
            n725 = property on="Got ADig bead" class="Bool (strict)"("Val(Sgnl)"=w1251) -> ()  [unwired: 2 in, 2 out]
          }
        }
      }
      frame "Dump" {
        n726 = case shown="True" w1252 {
          selector: w1252 -> [_ w1253]
          frame False {
          }
          frame True {
            n727 = property on="Dump beads" class="Bool (strict)"("Val(Sgnl)"=w1253) -> ()  [unwired: 2 in, 2 out]
          }
        }
      }
      frame "Fish" {
        n728 = case shown="True" w1254 {
          frame False {
          }
          frame True {
            n729 = local read "Fish"() -> (w1255:bool)
            n730 = Not(x=w1255) -> (.not. x?=w1256:bool)
            n731 = property on="Fish" class="Bool (strict)"("Val(Sgnl)"=w1256) -> ()  [unwired: 2 in, 2 out]
          }
        }
      }
      frame "Got DNA" {
        n732 = case shown="True" w1257 {
          selector: w1257 -> [_ w1258]
          frame False {
          }
          frame True {
            n733 = property on="Got DNA bead" class="Bool (strict)"("Val(Sgnl)"=w1258) -> ()  [unwired: 2 in, 2 out]
          }
        }
      }
    }
    n734 = case shown="True" w1204 {
      frame False {
      }
      frame True {
        n735 = local read "Shutter 2 (A)"() -> (w1269:bool)
        n736 = Not(x=w1269) -> (.not. x?=w1268:bool)
        n737 = property on="Shutter 2 (A)" class="Bool (strict)"("Val(Sgnl)"=w1268) -> ()  [unwired: 2 in, 2 out]
      }
    }
    n738 = Unbundle By Name(w1210) -> ("Right X"=w1182:i8, "Right Y"=w1184:i8, "Left X"=w1186:i8, "Left Y"=w1191:i8)
    n739 = Not Equal?(x=w1191, y=i8 0) -> (x != y?=w1192:bool)
    n740 = case shown="True" w1192 {
      tunnel: w1191 -> [_ w1231]
      frame False {
      }
      frame True {
        "Left Y" <- w1231
      }
    }
    n741 = case shown="\"Got DNA\", Default" "B command" {
      tunnel: w1198 -> [w1241 w1243 w1245 w1247]
      frame "Got DNA", Default {
        n742 = case shown="True" w1241 {
          selector: w1241 -> [_ w1242]
          frame False {
          }
          frame True {
            n743 = property on="Got DNA bead" class="Bool (strict)"("Val(Sgnl)"=w1242) -> ()  [unwired: 2 in, 2 out]
          }
        }
      }
      frame "Got ADig" {
        n744 = case shown="True" w1243 {
          selector: w1243 -> [_ w1244]
          frame False {
          }
          frame True {
            n745 = property on="Got ADig bead" class="Bool (strict)"("Val(Sgnl)"=w1244) -> ()  [unwired: 2 in, 2 out]
          }
        }
      }
      frame "Dump" {
        n746 = case shown="True" w1245 {
          selector: w1245 -> [_ w1246]
          frame False {
          }
          frame True {
            n747 = property on="Dump beads" class="Bool (strict)"("Val(Sgnl)"=w1246) -> ()  [unwired: 2 in, 2 out]
          }
        }
      }
      frame "Fish" {
        n748 = case shown="True" w1247 {
          frame False {
          }
          frame True {
            n749 = local read "Fish"() -> (w1248:bool)
            n750 = Not(x=w1248) -> (.not. x?=w1249:bool)
            n751 = property on="Fish" class="Bool (strict)"("Val(Sgnl)"=w1249) -> ()  [unwired: 2 in, 2 out]
          }
        }
      }
    }
    n752 = Not Equal?(x=w1182, y=i8 0) -> (x != y?=w1183:bool)
    n753 = Not Equal?(x=w1184, y=i8 0) -> (x != y?=w1185:bool)
    n754 = Not Equal?(x=w1186, y=i8 0) -> (x != y?=w1187:bool)
    n755 = case shown="True" w1187 {
      tunnel: w1186 -> [_ w1230]
      frame False {
      }
      frame True {
        "Left X" <- w1230
      }
    }
    n756 = case shown="False" w1183 {
      tunnel: w1182 -> [_ w1228]
      frame False {
      }
      frame True {
        "Right X" <- w1228
      }
    }
    n757 = case shown="False" w1185 {
      tunnel: w1184 -> [_ w1229]
      frame False {
      }
      frame True {
        "Right Y" <- w1229
      }
    }
    n758 = case shown="\"Dump\", Default" "X command" {
      tunnel: w1203 -> [w1259 w1261 w1264 w1266]
      frame "Dump", Default {
        n759 = case shown="True" w1259 {
          selector: w1259 -> [_ w1260]
          frame False {
          }
          frame True {
            n760 = property on="Dump beads" class="Bool (strict)"("Val(Sgnl)"=w1260) -> ()  [unwired: 2 in, 2 out]
          }
        }
      }
      frame "Fish" {
        n761 = case shown="True" w1261 {
          frame False {
          }
          frame True {
            n762 = local read "Fish"() -> (w1263:bool)
            n763 = Not(x=w1263) -> (.not. x?=w1262:bool)
            n764 = property on="Fish" class="Bool (strict)"("Val(Sgnl)"=w1262) -> ()  [unwired: 2 in, 2 out]
          }
        }
      }
      frame "Got ADig" {
        n765 = case shown="True" w1264 {
          selector: w1264 -> [_ w1265]
          frame False {
          }
          frame True {
            n766 = property on="Got ADig bead" class="Bool (strict)"("Val(Sgnl)"=w1265) -> ()  [unwired: 2 in, 2 out]
          }
        }
      }
      frame "Got DNA" {
        n767 = case shown="True" w1266 {
          selector: w1266 -> [_ w1267]
          frame False {
          }
          frame True {
            n768 = property on="Got DNA bead" class="Bool (strict)"("Val(Sgnl)"=w1267) -> ()  [unwired: 2 in, 2 out]
          }
        }
      }
    }
    n769 = case shown="\"Fish\", Default" "Y command" {
      tunnel: w1196 -> [w1232 w1235 w1237 w1239]
      frame "Fish", Default {
        n770 = case shown="True" w1232 {
          frame False {
          }
          frame True {
            n771 = local read "Fish"() -> (w1233:bool)
            n772 = Not(x=w1233) -> (.not. x?=w1234:bool)
            n773 = property on="Fish" class="Bool (strict)"("Val(Sgnl)"=w1234) -> ()  [unwired: 2 in, 2 out]
          }
        }
      }
      frame "Dump" {
        n774 = case shown="True" w1235 {
          selector: w1235 -> [_ w1236]
          frame False {
          }
          frame True {
            n775 = property on="Dump beads" class="Bool (strict)"("Val(Sgnl)"=w1236) -> ()  [unwired: 2 in, 2 out]
          }
        }
      }
      frame "Got ADig" {
        n776 = case shown="True" w1237 {
          selector: w1237 -> [_ w1238]
          frame False {
          }
          frame True {
            n777 = property on="Got ADig bead" class="Bool (strict)"("Val(Sgnl)"=w1238) -> ()  [unwired: 2 in, 2 out]
          }
        }
      }
      frame "Got DNA" {
        n778 = case shown="True" w1239 {
          selector: w1239 -> [_ w1240]
          frame False {
          }
          frame True {
            n779 = property on="Got DNA bead" class="Bool (strict)"("Val(Sgnl)"=w1240) -> ()  [unwired: 2 in, 2 out]
          }
        }
      }
    }
    n780 = local read "Stop"() -> (w1218:bool)
  }
  n781 = VISA Close(VISA resource name=w4, error in (no error)=w3) -> (error out=w5:errorcluster)
  n782 = call <vilib>:"Simple Error Handler.vi"("error in (no error)"=w5) -> ()  [unwired: 1 in, 8 out]
  n783 = node-c288(i64 100 ("Period"), 2 ("Processor")) -> (w30:T13)  [unwired: 2 in]
  n784 = timed-loop {
    timing: w30 -> [_]
    timing-out: [_] -> w29
    tunnel: w2 -> [w1272]
    tunnel: w28 -> [w1274]
    tunnel: [w1272] -> w27
    stop <- w1273 stop-if-true
    n785 = node-c288() -> ()  [unwired: 1 in, 1 out]
    n786 = event shown="[8] \"Repeat Dip\": Value Change" {
      selector: _ -> [_ _ _ _ _ _ _ _ _ _ _ _ _ _ _]
      dyn-events: _ -> [_ _ _ _ _ _ _ _ _ _ _ _ _ _ _]
      timeout: _ -> [_ _ _ _ _ _ _ _ _ _ _ _ _ _ _]
      tunnel: w1272 -> [w1281 w1333 w1353 w1371 w1388 w1409 w1457 w1472 w1547 _ _ _ _ _ _]
      tunnel: w1274 -> [w1280 w1332 w1352 w1370 w1387 w1408 w1456 w1471 w1545 _ _ _ _ _ _]
      tunnel: [_ _ _ _ _ _ _ _ _ _ _ _ _ _ w1729] -> w1273
      event "Got DNA bead": Value Change {
        n787 = event-data() -> ()  [unwired: 1 in, 5 out]
        n788 = flat-sequence {
          tunnel: w1280 -> [w1284]
          tunnel: ["Cal @ Delta (nm)"] -> w1276
          tunnel: w1281 -> [w1286]
          tunnel: [w1300] -> w1279
          tunnel: w1276 -> [w1299]
          tunnel: w1279 -> [w1321]
          tunnel: [w1321] -> w1278
          tunnel: w1278 -> [w1323]
          tunnel: [w1323] -> w1277
          tunnel: w1277 -> [w1325]
          frame #0 {
            n789 = local read "Saved stage positions"() -> (w1287:dbl[][])
            n790 = property on="Inject Sample" class="Bool (strict)"("Val(Sgnl)"=TRUE ("Value (Signaling)")) -> ()  [unwired: 2 in, 2 out]
            n791 = disable-structure shown="Disabled" {
              frame Disabled {
                n792 = property on="Inject Pump 2" class="Bool (strict)"("Val(Sgnl)"=FALSE ("Inject Pump 2")) -> ()  [unwired: 2 in, 2 out]
              }
              frame Enabled {
              }
            }
            n793 = local write "Stage moving"(TRUE ("Stage moving")) -> ()
            n794 = property on="Trap delta (nm)" class="DigNum (strict)"("Val(Sgnl)"="Cal @ Delta (nm)") -> ()  [unwired: 2 in, 2 out]
            n795 = call "move to saved stage position.vi"("error in"=w1284, "Stage VISA resource name in"=w1286, "Position"="Cal stage position", "Saved Stage Positions"=w1287) -> ()  [unwired: 2 out]
          }
          frame #1 {
            n796 = local write "Stage moving"(FALSE ("Stage moving")) -> ()
            n797 = property on="Inject Sample" class="Bool (strict)"("Val(Sgnl)"=FALSE ("Value (Signaling)")) -> ()  [unwired: 2 in, 2 out]
            n798 = call <vilib>:"Beep.vi"() -> ()  [unwired: 12 in]
          }
          frame #2 {
            # "increased from 1000 to 5000 v6.4. \nMar.7,2018."
            n799 = Wait (ms)(milliseconds to wait=u32 5000) -> ()  [unwired: 1 out]
          }
          frame #3 {
            n800 = property on="Save cal" class="Bool (strict)"("Val(Sgnl)"=TRUE ("Value (Signaling)")) -> ()  [unwired: 2 in, 2 out]
          }
          frame #4 {
            n801 = Wait (ms)(milliseconds to wait=u32 2000) -> ()  [unwired: 1 out]
          }
          frame #5 {
            n802 = while {
              stop <- w1296 stop-if-true
              n803 = local read "Saving"() -> (w1297:bool)
              n804 = Not(x=w1297) -> (.not. x?=w1296:bool)
              n805 = Wait (ms)(milliseconds to wait=u32 100) -> ()  [unwired: 1 out]
            }
          }
          frame #6 {
            n806 = Wait (ms)(milliseconds to wait=u32 2000) -> ()  [unwired: 1 out]
          }
          frame #7 {
            n807 = stacked-sequence {
              tunnel: [_ _ _ _ _ _ w1315 _] -> w1300
              tunnel: w1299 -> [_ _ _ _ _ _ _ w1320]
              frame #0 {
                n808 = property on="Trap delta (nm)" class="DigNum (strict)"("Val(Sgnl)"="Offset @ Delta (nm)") -> ()  [unwired: 2 in, 2 out]
                n809 = Replace Array Subset(array=i32[] [0], new element="Offset raster set", index=0) -> (w1304:i32[])
                n810 = property on="Scan Parameters" class="Arr (strict)"("Index Values"=w1304) -> ()  [unwired: 2 in, 2 out]
              }
              frame #1 {
                n811 = Wait (ms)(milliseconds to wait=u32 200) -> ()  [unwired: 1 out]
              }
              frame #2 {
                n812 = property on="Load param" class="Bool (strict)"("Val(Sgnl)"=TRUE ("Load param")) -> ()  [unwired: 2 in, 2 out]
              }
              frame #3 {
                n813 = Wait (ms)(milliseconds to wait=u32 200) -> ()  [unwired: 1 out]
              }
              frame #4 {
                # "Only continue if there is no buffer\noverflow error"
                n814 = local read "Buffer Overflow"() -> (w1310:bool)
                n815 = Not(x=w1310) -> (.not. x?=w1309:bool)
                n816 = case shown="True" w1309 {
                  frame False {
                  }
                  frame True {
                    n817 = property on="Raster scan" class="Bool (strict)"("Val(Sgnl)"=TRUE ("Value (Signaling)")) -> ()  [unwired: 2 in, 2 out]
                  }
                }
              }
              frame #5 {
                n818 = local read "Buffer Overflow"() -> (w1313:bool)
                n819 = Not(x=w1313) -> (.not. x?=w1312:bool)
                n820 = case shown="True" w1312 {
                  frame False {
                  }
                  frame True {
                    n821 = Wait (ms)(milliseconds to wait=u32 2000) -> ()  [unwired: 1 out]
                  }
                }
              }
              frame #6 {
                n822 = local read "Buffer Overflow"() -> (w1316:bool)
                n823 = Not(x=w1316) -> (.not. x?=w1315:bool)
                n824 = case shown="True" w1315 {
                  frame False {
                  }
                  frame True {
                    n825 = while {
                      stop <- w1318 stop-if-true
                      n826 = local read "Saving"() -> (w1319:bool)
                      n827 = Not(x=w1319) -> (.not. x?=w1318:bool)
                      n828 = Wait (ms)(milliseconds to wait=u32 100) -> ()  [unwired: 1 out]
                    }
                  }
                }
              }
              frame #7 {
                n829 = property on="Trap delta (nm)" class="DigNum (strict)"("Val(Sgnl)"=w1320) -> ()  [unwired: 2 in, 2 out]
              }
            }
          }
          frame #8 {
            n830 = case shown="True" w1321 {
              frame False {
              }
              frame True {
                n831 = property on="Read Cal" class="Bool (strict)"("Val(Sgnl)"=TRUE ("Value (Signaling)")) -> ()  [unwired: 2 in, 2 out]
              }
            }
          }
          frame #9 {
            n832 = case shown="True" w1323 {
              frame False {
              }
              frame True {
                n833 = Wait (ms)(milliseconds to wait=u32 1000) -> ()  [unwired: 1 out]
              }
            }
          }
          frame #10 {
            n834 = case shown="True" w1325 {
              frame False {
              }
              frame True {
                n835 = property on="Fish" class="Bool (strict)"("Val(Sgnl)"=TRUE ("Value (Signaling)")) -> ()  [unwired: 2 in, 2 out]
                n836 = case shown="False" "Flow on\nwhile fish?" {
                  frame False {
                    n837 = property on="Inject Sample" class="Bool (strict)"("Val(Sgnl)"=FALSE) -> ()  [unwired: 2 in, 2 out]
                  }
                  frame True {
                    n838 = property on="Inject Sample" class="Bool (strict)"("Val(Sgnl)"=TRUE ("Value (Signaling)")) -> ()  [unwired: 2 in, 2 out]
                  }
                }
              }
            }
          }
        }
        n839 = local write "Got DNA bead"(FALSE) -> ()
      }
      event "Dump beads": Value Change {
        n840 = event-data() -> ()  [unwired: 1 in, 5 out]
        n841 = flat-sequence {
          tunnel: w1332 -> [w1336]
          tunnel: w1333 -> [w1337]
          tunnel: [w1337] -> w1331
          tunnel: [w1336] -> w1330
          tunnel: w1331 -> [w1340]
          tunnel: w1330 -> [w1339]
          frame #0 {
            w1334 = FALSE ("Fish")
            n842 = local read "Saving"() -> (w1335:bool)
            n843 = local write "Force Feedback 2"(w1334) -> ()
            n844 = local write "Pause dwell"(w1334) -> ()
            n845 = local write "Force Feedback 1"(w1334) -> ()
            n846 = local write "Dump beads"(w1334) -> ()
            n847 = property on="Stop saving" class="Bool (strict)"("Val(Sgnl)"=w1335) -> ()  [unwired: 2 in, 2 out]
            n848 = local write "Fish"(w1334) -> ()
          }
          frame #1 {
            n849 = local read "Saved stage positions"() -> (w1342:dbl[][])
            n850 = case shown="True" "Flow on\ndump?" {
              frame False {
              }
              frame True {
                n851 = property on="Inject Sample" class="Bool (strict)"("Val(Sgnl)"=TRUE ("Value (Signaling)")) -> ()  [unwired: 2 in, 2 out]
              }
            }
            n852 = local write "Stage moving"(TRUE ("Stage moving")) -> ()
            n853 = call "move to saved stage position.vi"("error in"=w1339, "Stage VISA resource name in"=w1340, "Position"=5, "Saved Stage Positions"=w1342) -> ()  [unwired: 2 out]
          }
          frame #2 {
            n854 = local read "Shutter 1 (B)"() -> (w1347:bool)
            n855 = local read "Shutter 2 (A)"() -> (w1346:bool)
            n856 = call <vilib>:"Beep.vi"() -> ()  [unwired: 12 in]
            n857 = case shown="True" w1347 {
              frame False {
              }
              frame True {
                n858 = property on="Shutter 1 (B)" class="Bool (strict)"("Val(Sgnl)"=FALSE ("Value (Signaling)")) -> ()  [unwired: 2 in, 2 out]
              }
            }
            n859 = case shown="True" w1346 {
              frame False {
              }
              frame True {
                n860 = property on="Shutter 2 (A)" class="Bool (strict)"("Val(Sgnl)"=FALSE) -> ()  [unwired: 2 in, 2 out]
              }
            }
            n861 = local write "Stage moving"(FALSE ("Stage moving")) -> ()
            n862 = local write "Tether"(FALSE ("Tether")) -> ()
          }
          frame #3 {
            n863 = property on="Move Cap. 2 (ADig Top)" class="Bool (strict)"("Val(Sgnl)"=TRUE ("Value (Signaling)")) -> ()  [unwired: 2 in, 2 out]
          }
        }
      }
      event "Move Cap. 2 (ADig Top)": Value Change {
        n864 = event-data() -> ()  [unwired: 1 in, 5 out]
        n865 = flat-sequence {
          tunnel: w1353 -> [w1357]
          tunnel: w1352 -> [w1356]
          frame #0 {
            n866 = local read "Saved stage positions"() -> (w1355:dbl[][])
            n867 = case shown="True" "Flow on\ncap 2?" {
              frame False {
              }
              frame True {
                n868 = property on="Inject Sample" class="Bool (strict)"("Val(Sgnl)"=TRUE ("Value (Signaling)")) -> ()  [unwired: 2 in, 2 out]
              }
            }
            n869 = local write "Move Cap. 2 (ADig Top)"(FALSE ("Move Cap. 2 (ADig Top)")) -> ()
            n870 = local write "Stage moving"(TRUE ("Stage moving")) -> ()
            n871 = call "move to saved stage position.vi"("error in"=w1356, "Stage VISA resource name in"=w1357, "Position"=2, "Saved Stage Positions"=w1355) -> ()  [unwired: 2 out]
          }
          frame #1 {
            # "Make sure you don't reverse\nwhich is ON and OFF"
            n872 = local read "Cal @ Delta (nm)"() -> (w1365:dbl)
            n873 = local write "Stage moving"(FALSE ("Stage moving")) -> ()
            n874 = call <vilib>:"Beep.vi"() -> ()  [unwired: 12 in]
            n875 = property on="Trap delta (nm)" class="DigNum (strict)"("Val(Sgnl)"=w1365) -> ()  [unwired: 2 in, 2 out]
            n876 = property class="TabCtl (strict)"("Val(Sgnl)"=T4."Status" ("Value (Signaling)")) -> ()  [unwired: 2 in, 2 out]
            n877 = disable-structure shown="Disabled" {
              frame Disabled {
                n878 = property on="Inject Pump 1" class="Bool (strict)"("Val(Sgnl)"=TRUE ("Inject Pump 2")) -> ()  [unwired: 2 in, 2 out]
              }
              frame Enabled {
              }
            }
            n879 = local read "Shutter 2 (A)"() -> (w1364:bool)
            n880 = case shown="False" w1364 {
              frame False {
                n881 = property on="Shutter 2 (A)" class="Bool (strict)"("Val(Sgnl)"=TRUE ("Value (Signaling)")) -> ()  [unwired: 2 in, 2 out]
              }
              frame True {
              }
            }
            n882 = property on="Inject Sample" class="Bool (strict)"("Val(Sgnl)"=FALSE ("Value (Signaling)")) -> ()  [unwired: 2 in, 2 out]
          }
        }
      }
      event "Got ADig bead": Value Change {
        n883 = event-data() -> ()  [unwired: 1 in, 5 out]
        n884 = flat-sequence {
          tunnel: w1371 -> [w1375]
          tunnel: w1370 -> [w1374]
          frame #0 {
            n885 = local read "Saved stage positions"() -> (w1377:dbl[][])
            n886 = property on="Inject Pump 1" class="Bool (strict)"("Val(Sgnl)"=FALSE ("Inject Pump 2")) -> ()  [unwired: 2 in, 2 out]
            n887 = case shown="True" "Flow on\ncap 1?" {
              frame False {
              }
              frame True {
                n888 = property on="Inject Sample" class="Bool (strict)"("Val(Sgnl)"=TRUE ("Value (Signaling)")) -> ()  [unwired: 2 in, 2 out]
              }
            }
            n889 = local write "Stage moving"(TRUE ("Stage moving")) -> ()
            n890 = call "move to saved stage position.vi"("error in"=w1374, "Stage VISA resource name in"=w1375, "Position"=1, "Saved Stage Positions"=w1377) -> ()  [unwired: 2 out]
          }
          frame #1 {
            n891 = local read "Shutter 1 (B)"() -> (w1381:bool)
            n892 = disable-structure shown="Disabled" {
              frame Disabled {
                n893 = property on="Inject Pump 2" class="Bool (strict)"("Val(Sgnl)"=TRUE ("Inject Pump 2")) -> ()  [unwired: 2 in, 2 out]
              }
              frame Enabled {
              }
            }
            n894 = local write "Stage moving"(FALSE ("Stage moving")) -> ()
            n895 = case shown="False" w1381 {
              frame False {
                n896 = property on="Shutter 1 (B)" class="Bool (strict)"("Val(Sgnl)"=TRUE ("Value (Signaling)")) -> ()  [unwired: 2 in, 2 out]
              }
              frame True {
              }
            }
            n897 = property on="Inject Sample" class="Bool (strict)"("Val(Sgnl)"=FALSE ("Value (Signaling)")) -> ()  [unwired: 2 in, 2 out]
            n898 = call <vilib>:"Beep.vi"() -> ()  [unwired: 12 in]
          }
        }
        n899 = local write "Got ADig bead"(FALSE ("Got ADig bead")) -> ()
      }
      event "Set Position 1", "Set Position 2", "Set Position 3", "Set Position 4", "Set Position 5": Value Change {
        n900 = event-data() -> ()  [unwired: 1 in, 5 out]
        n901 = Build Array("Set Position 1", "Set Position 2", "Set Position 3", "Set Position 4", "Set Position 5") -> (w1400:bool[])
        n902 = Boolean Array To Number(Boolean array=w1400) -> (number=w1399:u32)
        n903 = call "Read Stage Position.vi"("error in"=w1387, "VISA resource name in"=w1388) -> ("Current Position"=w1385:cluster{dbl, dbl, dbl}, "error out"=→"Stage error":errorcluster)  [unwired: 1 in, 1 out]
        n904 = Logarithm Base 2(1:w1399) -> (0:w1393:dbl)
        n905 = Cluster To Array(cluster=w1385) -> (array=w1395:dbl[])
        n906 = Increment(x=w1393) -> (x+1=w1396:dbl)
        n907 = Build Array (concatenate)(w1396, w1395) -> (w1394:dbl[])
        n908 = Replace Array Subset(array="Saved stage positions", new element=w1394, index (row)=w1393) -> (w1397:dbl[][])  [unwired: 1 in]
        n909 = local write "Saved stage positions"(w1397) -> ()
      }
      event "Move to Position 2", "Move to Position 4", "Move to Position 3", "Move to Position 5", "Move to Position 1": Value Change {
        w1403 = FALSE
        n910 = event-data() -> ()  [unwired: 1 in, 5 out]
        n911 = Build Array("Move to Position 1", "Move to Position 2", "Move to Position 3", "Move to Position 4", "Move to Position 5") -> (w1412:bool[])
        n912 = Boolean Array To Number(Boolean array=w1412) -> (number=w1411:u32)
        n913 = Logarithm Base 2(1:w1411) -> (0:w1410:dbl)
        n914 = flat-sequence {
          tunnel: w1410 -> [w1421]
          tunnel: w1409 -> [w1420]
          tunnel: w1408 -> [w1419]
          tunnel: [w1414] -> w1402
          tunnel: w1402 -> [w1431]
          frame #0 {
            # "only change move time when \nsaving move in T and calibrating is F"
            n915 = local read "Saved stage positions"() -> (w1422:dbl[][])
            n916 = property on="Saving Move" class="Bool (strict)"() -> ("Value"=w1416:bool)  [unwired: 2 in, 2 out]
            n917 = property on="Calibrating" class="Bool (strict)"() -> ("Value"=w1417:bool)  [unwired: 2 in, 2 out]
            n918 = Not(x=w1417) -> (.not. x?=w1415:bool)
            n919 = Increment(x=w1421) -> (x+1=w1414:dbl)
            n920 = And(x=w1416, y=w1415) -> (x .and. y?=w1418:bool)
            n921 = case shown="True" w1418 {
              frame False {
              }
              frame True {
                n922 = Get Date/Time In Seconds() -> (seconds since 1Jan1904=w1428:timestamp)
                n923 = Format Date/Time String(time format string (%c)="%H:%M:%S%3u", seconds (now)=w1428, UTC format=TRUE) -> (date/time string=w1427:string)
                n924 = call <vilib>:"Space Constant.vi"() -> ("String"=w1426:string)
                n925 = Concatenate Strings(w1427, w1426, "moving") -> (w1424:string)
                n926 = property on="Move time" class="Str"("Val(Sgnl)"=w1424) -> ()  [unwired: 2 in, 2 out]
              }
            }
            n927 = call "move to saved stage position.vi"("error in"=w1419, "Stage VISA resource name in"=w1420, "Position"=w1414, "Saved Stage Positions"=w1422) -> ()  [unwired: 2 out]
            n928 = call <vilib>:"Beep.vi"() -> ()  [unwired: 12 in]
            "Stage moving" <- TRUE ("Stage moving")
          }
          frame #1 {
            n929 = property on="Saving Move" class="Bool (strict)"() -> ("Value"=w1433:bool)  [unwired: 2 in, 2 out]
            n930 = property on="Calibrating" class="Bool (strict)"() -> ("Value"=w1434:bool)  [unwired: 2 in, 2 out]
            n931 = call <vilib>:"Beep.vi"() -> ()  [unwired: 12 in]
            n932 = Not(x=w1434) -> (.not. x?=w1432:bool)
            n933 = local write "Stage moving"(FALSE ("Stage moving")) -> ()
            n934 = And(x=w1433, y=w1432) -> (x .and. y?=w1435:bool)
            n935 = case shown="True" w1435 {
              tunnel: w1431 -> [_ w1439]
              frame False {
              }
              frame True {
                n936 = Get Date/Time In Seconds() -> (seconds since 1Jan1904=w1443:timestamp)
                n937 = Format Date/Time String(time format string (%c)="%H:%M:%S%3u", seconds (now)=w1443, UTC format=TRUE) -> (date/time string=w1442:string)
                n938 = Number To Decimal String(number=w1439, width (-)=i16 1) -> (decimal integer string=w1437:string)
                n939 = call <vilib>:"Space Constant.vi"() -> ("String"=w1440:string)
                n940 = Concatenate Strings(w1442, w1440, w1437) -> (w1441:string)
                n941 = property on="Move time" class="Str"("Val(Sgnl)"=w1441) -> ()  [unwired: 2 in, 2 out]
              }
            }
          }
        }
        n942 = local write "Move to Position 1"(w1403) -> ()
        n943 = local write "Move to Position 2"(w1403) -> ()
        n944 = local write "Move to Position 3"(w1403) -> ()
        n945 = local write "Move to Position 4"(w1403) -> ()
        n946 = local write "Move to Position 5"(w1403) -> ()
      }
      event "Set Current\nPos to (0,0,0)": Value Change {
        w1447 = ";" ("string")
        # "DH is \"Define Home\" -KW"
        n947 = event-data() -> ()  [unwired: 1 in, 5 out]
        n948 = local write "Set Current\nPos to (0,0,0)"(FALSE ("Set Current\nPos to (0,0,0)")) -> ()
        n949 = call-poly "VISA Configure Serial Port"("VISA resource name"=w1457, "baud rate (9600)"=u32 19200, "error in (no error)"=w1456) -> ("VISA resource name out"=w1451:refnum<visa-resource-name>, "error out"=w1450:errorcluster)  [unwired: 11 in]
        n950 = Concatenate Strings("1DH" ("string"), w1447, "2DH" ("string"), w1447, "3DH" ("string"), "\r") -> (w1449:string)
        n951 = VISA Write(VISA resource name=w1451, write buffer=w1449, error in (no error)=w1450) -> (error out=w1448:errorcluster)  [unwired: 2 out]
        n952 = local write "Stage error"(w1448) -> ()
      }
      event "Dip": Value Change {
        n953 = event-data() -> ()  [unwired: 1 in, 5 out]
        n954 = property on="Calibrating" class="Bool (strict)"() -> ("Value"=w1464:bool)  [unwired: 2 in, 2 out]
        n955 = Not(x=w1464) -> (.not. x?=w1462:bool)
        n956 = property on="Saving Move" class="Bool (strict)"() -> ("Value"=w1463:bool)  [unwired: 2 in, 2 out]
        n957 = And(x=w1463, y=w1462) -> (x .and. y?=w1461:bool)
        n958 = flat-sequence {
          tunnel: w1472 -> [w1476]
          tunnel: w1471 -> [w1475]
          tunnel: [w1477] -> w1469
          tunnel: [w1476] -> w1467
          tunnel: [w1475] -> w1465
          tunnel: w1461 -> [w1474]
          tunnel: ["Dip position"] -> w1460
          tunnel: [w1493] -> w1470
          tunnel: w1469 -> [w1493]
          tunnel: [w1492] -> w1468
          tunnel: w1467 -> [w1492]
          tunnel: [w1491] -> w1466
          tunnel: w1465 -> [w1491]
          tunnel: w1461 -> [w1487]
          tunnel: w1460 -> [w1486]
          tunnel: w1470 -> [w1524]
          tunnel: w1468 -> [w1523]
          tunnel: w1466 -> [w1522]
          tunnel: w1461 -> [w1520]
          tunnel: ["Start/Return position"] -> w1459
          tunnel: w1461 -> [w1533]
          tunnel: w1459 -> [w1532]
          frame #0 {
            n959 = local read "Saved stage positions"() -> (w1477:dbl[][])
            n960 = case shown="True" w1474 {
              frame False {
              }
              frame True {
                n961 = Get Date/Time In Seconds() -> (seconds since 1Jan1904=w1485:timestamp)
                n962 = call <vilib>:"Space Constant.vi"() -> ("String"=w1481:string)
                n963 = Format Date/Time String(time format string (%c)="%H:%M:%S%3u", seconds (now)=w1485, UTC format=TRUE) -> (date/time string=w1482:string)
                n964 = Concatenate Strings(w1482, w1481, "moving") -> (w1480:string)
                n965 = property on="Move time" class="Str"("Val(Sgnl)"=w1480) -> ()  [unwired: 2 in, 2 out]
              }
            }
            n966 = local write "Stage moving"(TRUE) -> ()
            n967 = call "move to saved stage position.vi"("error in"=w1475, "Stage VISA resource name in"=w1476, "Position"="Dip position", "Saved Stage Positions"=w1477) -> ()  [unwired: 2 out]
          }
          frame #1 {
            n968 = node-c288() -> (w1490:T13)  [unwired: 4 in]
            n969 = case shown="True" w1487 {
              tunnel: w1486 -> [_ w1497]
              frame False {
              }
              frame True {
                n970 = Get Date/Time In Seconds() -> (seconds since 1Jan1904=w1502:timestamp)
                n971 = Number To Decimal String(number=w1497, width (-)=i16 1) -> (decimal integer string=w1496:string)
                n972 = Format Date/Time String(time format string (%c)="%H:%M:%S%3u", seconds (now)=w1502, UTC format=TRUE) -> (date/time string=w1495:string)
                n973 = call <vilib>:"Space Constant.vi"() -> ("String"=w1499:string)
                n974 = Concatenate Strings(w1495, w1499, w1496) -> (w1494:string)
                n975 = property on="Move time" class="Str"("Val(Sgnl)"=w1494) -> ()  [unwired: 2 in, 2 out]
              }
            }
            n976 = timed-loop {
              timing: w1490 -> [_]
              timing-out: [_] -> w1489
              i -> [w1513]
              stop <- w1506 stop-if-true
              n977 = node-c288() -> ()  [unwired: 1 in, 1 out]
              n978 = local read "Cancel Rep\n Dip"() -> (w1503:bool)
              n979 = Greater Or Equal?(x=w1513, y="Dip duration") -> (x >= y?=w1509:bool)
              n980 = local read "Dump beads"() -> (w1504:bool)
              n981 = Or(x=w1509, y="Cancel dwell") -> (x .or. y?=w1508:bool)
              n982 = Not(x="Pause dwell") -> (.not. x?=w1510:bool)
              n983 = node-c288() -> ()  [unwired: 1 in, 1 out]
              n984 = And(x=w1510, y=w1508) -> (x .and. y?=w1507:bool)
              n985 = Compound Arithmetic op=OR(w1507, w1504, w1503) -> (w1506:bool)
              "Dip elasped time" <- w1513
            }
            n986 = local write "Stage moving"(FALSE ("Stage moving")) -> ()
            n987 = node-c288(w1489) -> ()  [unwired: 1 out]
          }
          frame #2 {
            w1518 = FALSE ("Cancel dwell")
            n988 = case shown="True" w1520 {
              frame False {
              }
              frame True {
                n989 = Get Date/Time In Seconds() -> (seconds since 1Jan1904=w1531:timestamp)
                n990 = Format Date/Time String(time format string (%c)="%H:%M:%S%3u", seconds (now)=w1531, UTC format=TRUE) -> (date/time string=w1528:string)
                n991 = call <vilib>:"Space Constant.vi"() -> ("String"=w1527:string)
                n992 = Concatenate Strings(w1528, w1527, "moving") -> (w1525:string)
                n993 = property on="Move time" class="Str"("Val(Sgnl)"=w1525) -> ()  [unwired: 2 in, 2 out]
              }
            }
            n994 = local write "Cancel dwell"(w1518) -> ()
            n995 = local write "Cancel Rep\n Dip"(w1518) -> ()
            n996 = local write "Stage moving"(TRUE) -> ()
            n997 = call "move to saved stage position.vi"("error in"=w1522, "Stage VISA resource name in"=w1523, "Position"="Start/Return position", "Saved Stage Positions"=w1524) -> ()  [unwired: 2 out]
          }
          frame #3 {
            n998 = case shown="True" w1533 {
              tunnel: w1532 -> [_ w1535]
              frame False {
              }
              frame True {
                n999 = Get Date/Time In Seconds() -> (seconds since 1Jan1904=w1543:timestamp)
                n1000 = Number To Decimal String(number=w1535, width (-)=i16 1) -> (decimal integer string=w1536:string)
                n1001 = call <vilib>:"Space Constant.vi"() -> ("String"=w1540:string)
                n1002 = Format Date/Time String(time format string (%c)="%H:%M:%S%3u", seconds (now)=w1543, UTC format=TRUE) -> (date/time string=w1537:string)
                n1003 = Concatenate Strings(w1537, w1540, w1536) -> (w1538:string)
                n1004 = property on="Move time" class="Str"("Val(Sgnl)"=w1538) -> ()  [unwired: 2 in, 2 out]
              }
            }
            n1005 = local write "Stage moving"(FALSE ("Stage moving")) -> ()
          }
          frame #4 {
            n1006 = local write "Dip"(FALSE ("Dip")) -> ()
          }
        }
      }
      event "Repeat Dip": Value Change {
        n1007 = event-data() -> ()  [unwired: 1 in, 6 out]
        n1008 = local read "Saved stage positions"() -> (w1548:dbl[][])
        n1009 = local read "Calibrating"() -> (w1551:bool)
        n1010 = local read "Saving Move"() -> (w1550:bool)
        n1011 = Not(x=w1551) -> (.not. x?=w1549:bool)
        n1012 = And(x=w1550, y=w1549) -> (x .and. y?=w1546:bool)
        n1013 = flat-sequence {
          tunnel: w1548 -> [w1555]
          tunnel: w1547 -> [w1554]
          tunnel: w1546 -> [w1553]
          tunnel: w1545 -> [w1552]
          frame #0 {
            n1014 = while {
              tunnel: w1555 -> [w1572]
              tunnel: w1554 -> [w1569]
              tunnel: w1553 -> [w1566]
              tunnel: w1553 -> [w1565]
              tunnel: w1552 -> [w1564]
              tunnel: w1552 -> [w1563]
              i -> [w1573]
              stop <- w1562 stop-if-true
              n1015 = flat-sequence {
                tunnel: w1572 -> [w1579]
                tunnel: [w1579] -> w1570
                tunnel: w1569 -> [w1578]
                tunnel: [w1578] -> w1567
                tunnel: w1566 -> [w1577]
                tunnel: w1564 -> [w1576]
                tunnel: [w1575] -> w1558
                tunnel: [w1591] -> w1571
                tunnel: w1570 -> [w1591]
                tunnel: [w1590] -> w1568
                tunnel: w1567 -> [w1590]
                tunnel: w1565 -> [w1589]
                tunnel: w1558 -> [w1588]
                tunnel: w1571 -> [w1624]
                tunnel: w1568 -> [w1623]
                tunnel: w1565 -> [w1622]
                tunnel: w1563 -> [w1621]
                tunnel: [w1620] -> w1557
                tunnel: w1565 -> [w1634]
                tunnel: w1557 -> [w1633]
                frame #0 {
                  n1016 = case shown="True" w1577 {
                    frame False {
                    }
                    frame True {
                      n1017 = Get Date/Time In Seconds() -> (seconds since 1Jan1904=w1587:timestamp)
                      n1018 = call <vilib>:"Space Constant.vi"() -> ("String"=w1583:string)
                      n1019 = Format Date/Time String(time format string (%c)="%H:%M:%S%3u", seconds (now)=w1587, UTC format=TRUE) -> (date/time string=w1584:string)
                      n1020 = Concatenate Strings(w1584, w1583, "moving") -> (w1581:string)
                      n1021 = property on="Move time" class="Str"("Val(Sgnl)"=w1581) -> ()  [unwired: 2 in, 2 out]
                    }
                  }
                  n1022 = local read "Dip position"() -> (w1575:dbl)
                  n1023 = local write "Stage moving"(TRUE) -> ()
                  n1024 = call "move to saved stage position.vi"("error in"=w1576, "Stage VISA resource name in"=w1578, "Position"=w1575, "Saved Stage Positions"=w1579) -> ()  [unwired: 2 out]
                }
                frame #1 {
                  # "IN DIPPING POSITION"
                  n1025 = node-c288() -> (w1594:T13)  [unwired: 4 in]
                  n1026 = case shown="True" w1589 {
                    tunnel: w1588 -> [_ w1599]
                    frame False {
                    }
                    frame True {
                      n1027 = Get Date/Time In Seconds() -> (seconds since 1Jan1904=w1603:timestamp)
                      n1028 = Format Date/Time String(time format string (%c)="%H:%M:%S%3u", seconds (now)=w1603, UTC format=TRUE) -> (date/time string=w1598:string)
                      n1029 = Number To Decimal String(number=w1599, width (-)=i16 1) -> (decimal integer string=w1596:string)
                      n1030 = call <vilib>:"Space Constant.vi"() -> ("String"=w1597:string)
                      n1031 = Concatenate Strings(w1598, w1597, w1596) -> (w1595:string)
                      n1032 = property on="Move time" class="Str"("Val(Sgnl)"=w1595) -> ()  [unwired: 2 in, 2 out]
                    }
                  }
                  n1033 = timed-loop {
                    timing: w1594 -> [_]
                    timing-out: [_] -> w1593
                    i -> [w1613]
                    stop <- w1605 stop-if-true
                    n1034 = node-c288() -> ()  [unwired: 1 in, 1 out]
                    n1035 = local read "Dip duration"() -> (w1612:dbl)
                    n1036 = local read "Cancel dwell"() -> (w1611:bool)
                    n1037 = local write "Dip elasped time"(w1613) -> ()
                    n1038 = To Double Precision Float(number=w1613) -> (double precision float=w1614:dbl)
                    n1039 = local read "Pause dwell"() -> (w1615:bool)
                    n1040 = Greater Or Equal?(x=w1614, y=w1612) -> (x >= y?=w1610:bool)
                    n1041 = local read "Dump beads"() -> (w1606:bool)
                    n1042 = Or(x=w1610, y=w1611) -> (x .or. y?=w1609:bool)
                    n1043 = Not(x=w1615) -> (.not. x?=w1608:bool)
                    n1044 = local read "Cancel Rep\n Dip"() -> (w1604:bool)
                    n1045 = And(x=w1608, y=w1609) -> (x .and. y?=w1607:bool)
                    n1046 = node-c288() -> ()  [unwired: 1 in, 1 out]
                    n1047 = Compound Arithmetic op=OR(w1604, w1607, w1606) -> (w1605:bool)
                  }
                  n1048 = local write "Stage moving"(FALSE) -> ()
                  n1049 = node-c288(w1593) -> ()  [unwired: 1 out]
                }
                frame #2 {
                  n1050 = case shown="True" w1622 {
                    frame False {
                    }
                    frame True {
                      n1051 = Get Date/Time In Seconds() -> (seconds since 1Jan1904=w1632:timestamp)
                      n1052 = call <vilib>:"Space Constant.vi"() -> ("String"=w1628:string)
                      n1053 = Format Date/Time String(time format string (%c)="%H:%M:%S%3u", seconds (now)=w1632, UTC format=TRUE) -> (date/time string=w1629:string)
                      n1054 = Concatenate Strings(w1629, w1628, "moving") -> (w1626:string)
                      n1055 = property on="Move time" class="Str"("Val(Sgnl)"=w1626) -> ()  [unwired: 2 in, 2 out]
                    }
                  }
                  n1056 = local read "Start/Return position"() -> (w1620:dbl)
                  n1057 = local write "Stage moving"(TRUE) -> ()
                  n1058 = call "move to saved stage position.vi"("error in"=w1621, "Stage VISA resource name in"=w1623, "Position"=w1620, "Saved Stage Positions"=w1624) -> ()  [unwired: 2 out]
                }
                frame #3 {
                  # "IN RETURN POSITION"
                  n1059 = node-c288() -> (w1637:T13)  [unwired: 4 in]
                  n1060 = timed-loop {
                    timing: w1637 -> [_]
                    timing-out: [_] -> w1636
                    i -> [w1657]
                    stop <- w1648 stop-if-true
                    n1061 = node-c288() -> ()  [unwired: 1 in, 1 out]
                    n1062 = local read "Return duration"() -> (w1655:dbl)
                    n1063 = local read "Cancel dwell"() -> (w1653:bool)
                    n1064 = local write "Return elasped time"(w1657) -> ()
                    n1065 = To Double Precision Float(number=w1657) -> (double precision float=w1658:dbl)
                    n1066 = local read "Pause dwell"() -> (w1656:bool)
                    n1067 = Greater Or Equal?(x=w1658, y=w1655) -> (x >= y?=w1654:bool)
                    n1068 = local read "Dump beads"() -> (w1649:bool)
                    n1069 = Or(x=w1654, y=w1653) -> (x .or. y?=w1652:bool)
                    n1070 = local read "Cancel Rep\n Dip"() -> (w1647:bool)
                    n1071 = Not(x=w1656) -> (.not. x?=w1651:bool)
                    n1072 = node-c288() -> ()  [unwired: 1 in, 1 out]
                    n1073 = And(x=w1651, y=w1652) -> (x .and. y?=w1650:bool)
                    n1074 = Compound Arithmetic op=OR(w1647, w1650, w1649) -> (w1648:bool)
                  }
                  n1075 = case shown="True" w1634 {
                    tunnel: w1633 -> [_ w1642]
                    frame False {
                    }
                    frame True {
                      n1076 = Get Date/Time In Seconds() -> (seconds since 1Jan1904=w1646:timestamp)
                      n1077 = Format Date/Time String(time format string (%c)="%H:%M:%S%3u", seconds (now)=w1646, UTC format=TRUE) -> (date/time string=w1639:string)
                      n1078 = Number To Decimal String(number=w1642, width (-)=i16 1) -> (decimal integer string=w1641:string)
                      n1079 = call <vilib>:"Space Constant.vi"() -> ("String"=w1640:string)
                      n1080 = Concatenate Strings(w1639, w1640, w1641) -> (w1638:string)
                      n1081 = property on="Move time" class="Str"("Val(Sgnl)"=w1638) -> ()  [unwired: 2 in, 2 out]
                    }
                  }
                  n1082 = local write "Stage moving"(FALSE) -> ()
                  n1083 = node-c288(w1636) -> ()  [unwired: 1 out]
                }
              }
              n1084 = Increment(x=w1573) -> (x+1=w1560:i32)
              "Dip #" <- w1560
              n1085 = property on="Cancel Rep\n Dip" class="Bool (strict)"() -> ("Value"=w1556:bool)  [unwired: 2 in, 2 out]
              n1086 = To Double Precision Float(number=w1560) -> (double precision float=w1559:dbl)
              n1087 = Greater Or Equal?(x=w1559, y="Dip attempts") -> (x >= y?=w1574:bool)
              n1088 = Or(x=w1556, y=w1574) -> (x .or. y?=w1562:bool)
            }
          }
          frame #1 {
            w1663 = FALSE
            n1089 = local write "Cancel Rep\n Dip"(w1663) -> ()
            n1090 = call <vilib>:"Beep.vi"() -> ()  [unwired: 12 in]
            n1091 = local write "Repeat Dip"(w1663) -> ()
          }
        }
      }
      event "Force FB script": Value Change {
        n1092 = event-data() -> ()  [unwired: 1 in, 5 out]
        n1093 = flat-sequence {
          frame #0 {
            n1094 = disable-structure shown="Disabled" {
              frame Disabled {
                n1095 = local read "# Samples/channel"() -> (w1666:i32)
                n1096 = local write "# Samples/channel (in)"(w1666) -> ()
              }
              frame Enabled {
              }
            }
            n1097 = local write "Force FB script"(FALSE ("Force FB script")) -> ()
            n1098 = property on="Trap delta (nm)" class="DigNum (strict)"("Val(Sgnl)"="Start trap delta (nm)") -> ()  [unwired: 2 in, 2 out]
          }
          frame #1 {
            n1099 = Wait (ms)(milliseconds to wait=u32 500) -> ()  [unwired: 1 out]
          }
          frame #2 {
            n1100 = property on="Set reading to\nsetpoint 1" class="Bool (strict)"("Val(Sgnl)"=TRUE ("Value (Signaling)")) -> ()  [unwired: 2 in, 2 out]
          }
          frame #3 {
            n1101 = Wait (ms)(milliseconds to wait=u32 300) -> ()  [unwired: 1 out]
          }
          frame #4 {
            n1102 = local write "Force Feedback 1"(TRUE ("Force Feedback")) -> ()
            n1103 = property on="Tabs" class="TabCtl (strict)"("Val(Sgnl)"=T23."Force Feedback" ("Value (Signaling)")) -> ()  [unwired: 2 in, 2 out]
          }
          frame #5 {
            n1104 = property on="Save Data" class="Bool (strict)"("Val(Sgnl)"=TRUE ("Value (Signaling)")) -> ()  [unwired: 2 in, 2 out]
          }
          frame #6 {
            n1105 = Multiply(x="Wait before dip (s)", y=1000) -> (x*y=w1673:dbl)
            n1106 = Wait (ms)(milliseconds to wait=w1673) -> ()  [unwired: 1 out]
          }
          frame #7 {
            n1107 = case shown="True" "Start dipping after?" {
              selector: "Start dipping after?" -> [_ w1678]
              frame False {
              }
              frame True {
                n1108 = property on="Dip" class="Bool (strict)"("Val(Sgnl)"=w1678) -> ()  [unwired: 2 in, 2 out]
              }
            }
            n1109 = property on="Remove offsets" class="Bool (strict)"("Val(Sgnl)"=TRUE ("Value (Signaling)")) -> ()  [unwired: 2 in, 2 out]
          }
        }
      }
      event "Move 0": Value Change {
        n1110 = event-data() -> ()  [unwired: 1 in, 5 out]
        n1111 = local write "Move 0"(FALSE) -> ()
        n1112 = call "HalfWavePlate.vi"("Degrees"="\"Degrees\" 0", "Motor"=0) -> ()  [unwired: 1 in]
      }
      event "Move 1": Value Change {
        n1113 = event-data() -> ()  [unwired: 1 in, 5 out]
        n1114 = local write "Move 1"(FALSE) -> ()
        n1115 = call "HalfWavePlate.vi"("Degrees"="\"Degrees\" 1", "Motor"=1) -> ()  [unwired: 1 in]
      }
      event "Save user params": Value Change {
        n1116 = event-data() -> ()  [unwired: 1 in, 6 out]
        n1117 = local write "Save user params"(FALSE) -> ()
        n1118 = call "save control values.vi"("User"="User") -> ()  [unwired: 8 in, 1 out]
      }
      event "Load user params": Value Change {
        # "Exceptions. Don't load these parameters."
        n1119 = event-data() -> ()  [unwired: 1 in, 6 out]
        n1120 = local write "Load user params"(FALSE) -> ()
        n1121 = flat-sequence {
          tunnel: [w1711] -> w1702
          tunnel: [w1710] -> w1700
          tunnel: [w1709] -> w1698
          tunnel: [w1708] -> w1696
          tunnel: [w1707] -> w1694
          tunnel: [w1706] -> w1692
          tunnel: [w1705] -> w1690
          tunnel: [w1704] -> w1687
          tunnel: [w1719] -> w1703
          tunnel: w1702 -> [w1719]
          tunnel: [w1718] -> w1701
          tunnel: w1700 -> [w1718]
          tunnel: [w1717] -> w1699
          tunnel: w1698 -> [w1717]
          tunnel: [w1716] -> w1697
          tunnel: w1696 -> [w1716]
          tunnel: [w1715] -> w1695
          tunnel: w1694 -> [w1715]
          tunnel: [w1714] -> w1693
          tunnel: w1692 -> [w1714]
          tunnel: [w1713] -> w1691
          tunnel: w1690 -> [w1713]
          tunnel: [w1712] -> w1688
          tunnel: w1687 -> [w1712]
          tunnel: w1703 -> [w1728]
          tunnel: w1701 -> [w1727]
          tunnel: w1699 -> [w1726]
          tunnel: w1697 -> [w1725]
          tunnel: w1695 -> [w1724]
          tunnel: w1693 -> [w1723]
          tunnel: w1691 -> [w1722]
          tunnel: w1688 -> [w1721]
          frame #0 {
            n1122 = local read "Force Feedback 2"() -> (w1704:bool)
            n1123 = local read "Force Feedback 1"() -> (w1705:bool)
            n1124 = local read "Shutter 1 (B)"() -> (w1711:bool)
            n1125 = local read "Shutter 2 (A)"() -> (w1710:bool)
            n1126 = local read "Inject Sample"() -> (w1708:bool)
            n1127 = local read "Trap delta (nm)"() -> (w1707:dbl)
            n1128 = local read "Save file index"() -> (w1706:i32)
            n1129 = local read "Fish"() -> (w1709:bool)
          }
          frame #1 {
            n1130 = local read "User"() -> (w1720:string)
            n1131 = call "retrieve control values.vi"("User"=w1720) -> ()  [unwired: 10 in, 1 out]
          }
          frame #2 {
            n1132 = local write "Force Feedback 1"(w1722) -> ()
            n1133 = local write "Force Feedback 2"(w1721) -> ()
            n1134 = local write "Trap delta (nm)"(w1724) -> ()
            n1135 = local write "Save file index"(w1723) -> ()
            n1136 = local write "Inject Sample"(w1725) -> ()
            n1137 = local write "Shutter 2 (A)"(w1727) -> ()
            n1138 = local write "Shutter 1 (B)"(w1728) -> ()
            n1139 = local write "Fish"(w1726) -> ()
          }
        }
      }
      event "Stop": Value Change {
        n1140 = event-data() -> ()  [unwired: 1 in, 5 out]
        n1141 = local read "Stop"() -> (w1729:bool)
      }
    }
    n1142 = node-c288() -> ()  [unwired: 1 in, 1 out]
  }
  n1143 = call-poly <vilib>:"DAQmx Create Virtual Channel.vi"("lines"=w98) -> ("task out"=w97:refnum<k21>)  [unwired: 13 in, 1 out]
  n1144 = call-poly <vilib>:"DAQmx Create Virtual Channel.vi"("lines"=w101) -> ("task out"=w100:refnum<k21>)  [unwired: 13 in, 1 out]
  n1145 = node-c288(2 ("Processor")) -> (w82:T13)  [unwired: 3 in]
  n1146 = timed-loop {
    timing: w82 -> [_]
    timing-out: [_] -> w81
    stop <- w1732 stop-if-true
    n1147 = node-c288() -> ()  [unwired: 1 in, 1 out]
    n1148 = case shown="\"Control\"" "Tab Control" {
      frame "Control" {
        n1149 = case shown="True" "Start" {
          frame False {
          }
          frame True {
            w1745 = T24 3 items=["no dialog", "OK message", "continue or stop message", "OK message + warnings", "continue/stop + warnings"] ("type of dialog (OK msg:1)")
            n1150 = call "InitializeAcquireFF.vi"("DAQ Rate"="DAQ Rate", "Averaging Number"="Averaging Number", "Sampling Rate"="Sampling Rate") -> ("error out"=w1739:errorcluster, "task out"=w1738:refnum<k21>, "Final Sampling Rate"=→"Final Sampling Rate":dbl)  [unwired: 4 in, 2 out]
            n1151 = while {
              tunnel: [w1757] -> w1744
              tunnel: [w1756] -> w1737
              tunnel: "Averaging Number" -> [w1755]
              tunnel: w1739 -> [w1754]
              tunnel: w1738 -> [w1752]
              stop <- w1753 continue-if-true
              n1152 = call "Acquire2_QPD.vi"("task/channels in"=w1752, "Save Data?"=FALSE ("Take Data?"), "Averaging Number"=w1755, "error in"=w1754) -> ("PSD 1"=→"PSD 1":cluster{dbl[], dbl[]}, "PSD 1 Sum"=→"PSD 1 Sum":dbl, "PSD 2"=→"PSD 2":cluster{dbl[], dbl[]}, "PSD 2 Sum"=→"PSD 2 Sum":dbl, "task out"=w1757:refnum<k21>, "error out"=w1756:errorcluster)  [unwired: 14 in, 4 out]
              n1153 = local read "Start"() -> (w1753:bool)
            }
            n1154 = call <vilib>:"DAQmx Clear Task.vi"("task in"=w1744, "error in"=w1737) -> ("error out"=w1746:errorcluster)  [unwired: 13 in]
            n1155 = call <vilib>:"Simple Error Handler.vi"("type of dialog (OK msg:1)"=w1745, "error in (no error)"=w1746) -> ()  [unwired: 3 in, 5 out]
          }
        }
      }
      frame "Current Saved Data" {
      }
      frame "Data Acquisition" {
      }
      frame "Raw QPD Data" {
      }
    }
    n1156 = local read "Stop"() -> (w1732:bool)
    n1157 = node-c288() -> ()  [unwired: 1 in, 1 out]
  }
  n1158 = node-c288(2 ("Processor")) -> (w34:T13)  [unwired: 3 in]
  n1159 = timed-loop {
    timing: w34 -> [_]
    timing-out: [_] -> w33
    stop <- w1758 stop-if-true
    n1160 = node-c288() -> ()  [unwired: 1 in, 1 out]
    n1161 = event shown="[0] \"Pause Mouse/Mirror Connection\": Value Change" {
      selector: _ -> [_ _]
      dyn-events: _ -> [_ _]
      timeout: _ -> [_ _]
      tunnel: [w1851 _] -> w1759
      tunnel: [_ w1852] -> w1758
      event "Pause Mouse/Mirror Connection": Value Change {
        n1162 = event-data() -> ("NewVal"=w1851:bool)  [unwired: 1 in]
      }
      event "Stop": Value Change {
        n1163 = event-data() -> ("NewVal"=w1852:bool)  [unwired: 1 in]
      }
    }
    n1164 = case shown="True" w1759 {
      frame False {
      }
      frame True {
        n1165 = call "InitializeMouseControl.vi"() -> ("error out 2"=w1768:errorcluster, "task out"=w1769:refnum<k21>, "error out"=w1771:errorcluster, "device ID"=w1770:refnum<k1>)  [unwired: 8 in]
        n1166 = while {
          tunnel: w1771 -> [w1783]
          tunnel: w1770 -> [w1782]
          tunnel: w1769 -> [w1781]
          tunnel: w1768 -> [w1780]
          tunnel: [w1779] -> w1766
          tunnel: [w1778] -> w1765
          tunnel: [w1777] -> w1762
          tunnel: [w1776] -> w1763
          stop <- w1775 stop-if-true
          n1167 = case shown="True" "Use Mouse to Move Trap?" {
            tunnel: w1782 -> [w1790 w1813]
            tunnel: w1783 -> [w1789 w1812]
            tunnel: w1781 -> [w1788 w1811]
            tunnel: w1780 -> [w1787 w1810]
            tunnel: [w1790 w1809] -> w1777
            tunnel: [w1789 w1808] -> w1776
            tunnel: [w1788 w1807] -> w1779
            tunnel: [w1787 w1806] -> w1778
            frame False {
              (unwired) FALSE ("button 1")
            }
            frame True {
              w1801 = 0.0 ("y")
              w1803 = 10
              n1168 = local read "Deflection"() -> (w1814:T5)
              n1169 = call-poly <vilib>:"Acquire Input Data.vi"("device ID"=w1813, "error in (no error)"=w1812) -> ("device ID"=w1809:refnum<k1>, "button info"=w1827:T25, "error out"=w1808:errorcluster)  [unwired: 14 in, 1 out]
              n1170 = Unbundle By Name(w1814) -> ("Horizontal"=w1816:i32, "Vertical"=w1815:i32)
              n1171 = local read "Saved voltage"() -> (w1792:cluster{dbl, dbl})
              n1172 = Divide(x=w1816, y=30) -> (x/y=w1819:dbl)
              n1173 = Divide(x=w1815, y=-20) -> (x/y=w1820:dbl)
              n1174 = Unbundle By Name(w1827) -> ("button 1"=w1805:bool, "button 2"=w1821:bool)
              n1175 = Bundle(w1819, w1820) -> (w1797:cluster{dbl, dbl})  [unwired: 1 in]
              n1176 = local write "Reference Voltage"(w1797) -> ()
              n1177 = Add(x=w1797, y=w1792) -> (x+y=w1825:cluster{dbl, dbl})
              n1178 = case shown="True" w1805 {
                frame False {
                  n1179 = stacked-sequence {
                    frame #0 {
                      n1180 = local write "CoordinatesMousePressed"(T5 {"Horizontal"=0, "Vertical"=0} ("Coords when pressed")) -> ()
                      n1181 = local write "Deflection"(T5 {"Horizontal"=0, "Vertical"=0} ("deflaction")) -> ()
                    }
                  }
                }
                frame True {
                  n1182 = local read "CoordinatesMousePressed"() -> (w1850:T5)
                  n1183 = local read "Real Coordinates"() -> (w1849:cluster{"Horizontal":i32, "Vertical":i32})
                  n1184 = Subtract(x=w1849, y=w1850) -> (x-y=w1848:T5)
                  n1185 = local write "Deflection"(w1848) -> ()
                }
              }
              n1186 = Unbundle(w1825) -> (w1802:dbl, w1793:dbl)
              n1187 = case shown="True" w1821 {
                frame False {
                }
                frame True {
                  n1188 = local read "Reference Voltage"() -> (w1831:cluster{dbl, dbl})
                  n1189 = local read "Saved voltage"() -> (w1829:cluster{dbl, dbl})
                  n1190 = Add(x=w1831, y=w1829) -> (x+y=→"Saved voltage":cluster{dbl, dbl})
                  n1191 = local read "Real Coordinates"() -> (w1830:cluster{"Horizontal":i32, "Vertical":i32})
                  n1192 = local write "CoordinatesMousePressed"(w1830) -> ()
                }
              }
              n1193 = Less?(x=w1802, y=w1803) -> (x < y?=w1800:bool)
              n1194 = Greater?(x=w1802, y=w1801) -> (0:w1799:bool)
              n1195 = Greater?(x=w1793, y=w1801) -> (0:w1795:bool)
              n1196 = Less?(x=w1793, y=w1803) -> (x < y?=w1796:bool)
              n1197 = And(x=w1795, y=w1796) -> (x .and. y?=w1794:bool)
              n1198 = And(x=w1800, y=w1799) -> (x .and. y?=w1798:bool)
              n1199 = case shown="False" w1794 {
                tunnel: [w1841 w1845] -> w1804
                tunnel: w1793 -> [w1839 w1845]
                frame False {
                  n1200 = Greater?(x=w1839, y=10.0) -> (0:w1842:bool)
                  n1201 = case shown="True" w1842 {
                    tunnel: [0.0 10.0] -> w1841
                    frame False {
                    }
                    frame True {
                    }
                  }
                }
                frame True {
                }
              }
              n1202 = case shown="False" w1798 {
                tunnel: w1802 -> [w1833 w1838]
                tunnel: [w1834 w1838] -> w1826
                frame False {
                  n1203 = Greater?(x=w1833, y=10.0) -> (0:w1835:bool)
                  n1204 = case shown="True" w1835 {
                    tunnel: [0.0 10.0] -> w1834
                    frame False {
                    }
                    frame True {
                    }
                  }
                }
                frame True {
                }
              }
              n1205 = Bundle(w1826, w1804) -> (w1791:cluster{dbl, dbl})  [unwired: 1 in]
              n1206 = Cluster To Array(cluster=w1791) -> (array=w1822:dbl[])
              n1207 = call-poly <vilib>:"DAQmx Write.vi"("task/channels in"=w1811, "data"=w1822, "error in"=w1810) -> ("task out"=w1824:refnum<k21>, "error out"=w1823:errorcluster)  [unwired: 10 in, 1 out]
              n1208 = call <vilib>:"DAQmx Is Task Done.vi"("task/channels in"=w1824, "error in"=w1823) -> ("task out"=w1807:refnum<k21>, "error out"=w1806:errorcluster)  [unwired: 11 in, 1 out]
            }
          }
          n1209 = event shown="[0] \"Pane\": Mouse Move" {
            selector: _ -> [_ _ _]
            dyn-events: _ -> [_ _ _]
            timeout: _ -> [_ _ _]
            event Mouse Move {
              n1210 = event-data() -> ("Coords"=w1785:T5)  [unwired: 1 in]
              n1211 = local write "Real Coordinates"(w1785) -> ()
            }
            event Mouse Down {
              n1212 = event-data() -> ("Coords"=w1786:T5)  [unwired: 1 in]
              n1213 = local write "CoordinatesMousePressed"(w1786) -> ()
            }
            event "Pause Mouse/Mirror Connection": Value Change {
              n1214 = event-data() -> ()  [unwired: 1 in, 3 out]
            }
          }
          n1215 = local read "Stop"() -> (w1772:bool)
          n1216 = Not(x="Pause Mouse/Mirror Connection") -> (.not. x?=w1773:bool)
          n1217 = Or(x=w1773, y=w1772) -> (x .or. y?=w1775:bool)
        }
        n1218 = call <vilib>:"DAQmx Clear Task.vi"("task in"=w1766, "error in"=w1765) -> ("error out"=w1767:errorcluster)  [unwired: 13 in]
        n1219 = call <vilib>:"Simple Error Handler.vi"("error in (no error)"=w1767) -> ()  [unwired: 4 in, 5 out]
        n1220 = call-poly <vilib>:"Close Input Device.vi"("error in (no error)"=w1763, "device ID"=w1762) -> ("error out"=w1764:errorcluster)  [unwired: 8 in]
        n1221 = call <vilib>:"Simple Error Handler.vi"("error in (no error)"=w1764) -> ()  [unwired: 4 in, 5 out]
      }
    }
    n1222 = node-c288() -> ()  [unwired: 1 in, 1 out]
  }
  n1223 = node-c288(i64 100 ("Period")) -> (w95:T13)  [unwired: 3 in]
  n1224 = timed-loop {
    tunnel: w97 -> [w1855]
    tunnel: [w1854] -> w96
    tunnel: w100 -> [w1857]
    tunnel: [w1856] -> w99
    timing: w95 -> [_]
    timing-out: [_] -> w94
    stop <- w1853 stop-if-true
    n1225 = node-c288() -> ()  [unwired: 1 in, 1 out]
    n1226 = event shown="[1] \"Shutter 2 (A)\": Value Change" {
      selector: _ -> [_ _ _]
      dyn-events: _ -> [_ _ _]
      timeout: _ -> [_ _ _]
      tunnel: w1857 -> [w1861 _ w1898]
      tunnel: [w1860 _ w1898] -> w1856
      tunnel: w1855 -> [_ w1881 w1899]
      tunnel: [_ w1879 w1899] -> w1854
      tunnel: [_ _ w1900] -> w1853
      event "Shutter 1 (B)": Value Change {
        n1227 = event-data() -> ()  [unwired: 1 in, 1 out]
        n1228 = flat-sequence {
          tunnel: [w1867] -> w1864
          tunnel: w1861 -> [w1866]
          tunnel: [w1871] -> w1863
          tunnel: [w1874] -> w1862
          tunnel: w1864 -> [w1869]
          tunnel: w1863 -> [w1878]
          tunnel: w1862 -> [w1876]
          tunnel: [w1875] -> w1860
          frame #0 {
            n1229 = call-poly <vilib>:"DAQmx Write.vi"("task/channels in"=w1866, "data"=FALSE) -> ("task out"=w1867:refnum<k21>)  [unwired: 11 in, 2 out]
            n1230 = Wait (ms)(milliseconds to wait=100) -> ()  [unwired: 1 out]
          }
          frame #1 {
            n1231 = Or(x="Shutter 1 (B)", y=TRUE) -> (x .or. y?=w1871:bool)
            n1232 = call-poly <vilib>:"DAQmx Write.vi"("task/channels in"=w1869, "data"=w1871) -> ("task out"=w1874:refnum<k21>)  [unwired: 11 in, 2 out]
            n1233 = Wait (ms)(milliseconds to wait=100) -> ()  [unwired: 1 out]
          }
          frame #2 {
            n1234 = Not(x=w1878) -> (.not. x?=w1877:bool)
            n1235 = call-poly <vilib>:"DAQmx Write.vi"("task/channels in"=w1876, "data"=w1877) -> ("task out"=w1875:refnum<k21>)  [unwired: 11 in, 2 out]
          }
        }
      }
      event "Shutter 2 (A)": Value Change {
        n1236 = event-data() -> ()  [unwired: 1 in, 1 out]
        n1237 = flat-sequence {
          tunnel: w1881 -> [w1886]
          tunnel: [w1885] -> w1880
          tunnel: [w1890] -> w1883
          tunnel: [w1893] -> w1882
          tunnel: w1880 -> [w1888]
          tunnel: w1883 -> [w1897]
          tunnel: w1882 -> [w1895]
          tunnel: [w1894] -> w1879
          frame #0 {
            n1238 = call-poly <vilib>:"DAQmx Write.vi"("task/channels in"=w1886, "data"=FALSE) -> ("task out"=w1885:refnum<k21>)  [unwired: 11 in, 2 out]
            n1239 = Wait (ms)(milliseconds to wait=100) -> ()  [unwired: 1 out]
          }
          frame #1 {
            n1240 = Or(x="Shutter 2 (A)", y=TRUE) -> (x .or. y?=w1890:bool)
            n1241 = call-poly <vilib>:"DAQmx Write.vi"("task/channels in"=w1888, "data"=w1890) -> ("task out"=w1893:refnum<k21>)  [unwired: 11 in, 2 out]
            n1242 = Wait (ms)(milliseconds to wait=100) -> ()  [unwired: 1 out]
          }
          frame #2 {
            n1243 = Not(x=w1897) -> (.not. x?=w1896:bool)
            n1244 = call-poly <vilib>:"DAQmx Write.vi"("task/channels in"=w1895, "data"=w1896) -> ("task out"=w1894:refnum<k21>)  [unwired: 11 in, 2 out]
          }
        }
      }
      event "Stop": Value Change {
        n1245 = event-data() -> ("NewVal"=w1900:bool)  [unwired: 1 in, 5 out]
      }
    }
    n1246 = node-c288() -> ()  [unwired: 1 in, 1 out]
  }
  n1247 = node-c288(w94) -> ()  [unwired: 1 out]
  n1248 = node-c288(w81) -> ()  [unwired: 1 out]
  n1249 = call <vilib>:"DAQmx Clear Task.vi"("task in"=w96) -> ()  [unwired: 14 in, 1 out]
  n1250 = call <vilib>:"DAQmx Clear Task.vi"("task in"=w99) -> ()  [unwired: 14 in, 1 out]
  n1251 = node-c288(w33) -> ()  [unwired: 1 out]
  n1252 = node-c288(w29) -> ()  [unwired: 1 out]
  n1253 = local write "Tether"(FALSE ("Tether")) -> ()
  n1254 = local read "Path"() -> (w88:path)
  n1255 = node-c288(i64 1 ("Period"), 2 ("Processor")) -> (w93:T13)  [unwired: 2 in]
  n1256 = timed-loop {
    timing: w93 -> [_]
    timing-out: [_] -> w92
    tunnel: w88 -> [w1902]
    stop <- w1901 stop-if-true
    n1257 = node-c288() -> ()  [unwired: 1 in, 1 out]
    n1258 = event shown="[5] \"Fish\": Value Change" {
      selector: _ -> [_ _ _ _ _ _ _ _ _ _]
      dyn-events: _ -> [_ _ _ _ _ _ _ _ _ _]
      timeout: _ -> [_ _ _ _ _ _ _ _ _ _]
      tunnel: w1902 -> [_ w1906 _ _ _ _ _ _ _ _]
      tunnel: [_ _ w1926 _ _ _ _ _ _ _] -> w1901
      event Timeout {
        n1259 = event-data() -> ()  [unwired: 1 in, 2 out]
      }
      event "Read Cal": Value Change {
        n1260 = event-data() -> ()  [unwired: 1 in, 6 out]
        n1261 = Path To String(path=w1906) -> (string=w1905:string)
        n1262 = Format Date/Time String(time format string (%c)="%y%m%d") -> (date/time string=w1907:string)  [unwired: 2 in]
        n1263 = Concatenate Strings(w1905, "\\" ("string"), w1907, "\\" ("string"), "current.cal") -> (w1925:string)
        n1264 = String To Path(string=w1925) -> (path=w1924:path)
        n1265 = Open/Create/Replace File(file path (use dialog)=w1924, operation (0:open)=T18."open", access (0:read/write)=enum16{"read/write", "read-only", "write-only"}."read-only") -> (refnum out=w1920:refnum<file>, error out=w1921:errorcluster)  [unwired: 3 in, 1 out]
        n1266 = Deny Access(4:w1921, 7:w1920) -> (0:w1919:errorcluster, 3:w1918:refnum<file>)  [unwired: 1 in]
        n1267 = Read from Binary File(5:0.0, 8:w1919, 9:T19."big-endian, network order" ("byte order (0:big-endian, network order)"), 10:12 ("count"), 11:w1918) -> (0:w1914:errorcluster, 2:w1912:dbl[], 3:w1915:refnum<file>)  [unwired: 1 in, 1 out]
        n1268 = Array To Cluster(array=w1912) -> (cluster=→"Cal values":T26)
        n1269 = Close File(refnum=w1915, error in=w1914) -> ()  [unwired: 2 out]
        n1270 = local write "Read Cal"(FALSE ("Read Cal")) -> ()
      }
      event "Stop": Value Change {
        n1271 = event-data() -> ("NewVal"=w1926:bool)  [unwired: 1 in, 5 out]
      }
      event "Trap position (V)": Value Change {
        # "Need to rotate so X and Y don't get mixed up."
        n1272 = event-data() -> ()  [unwired: 1 in, 6 out]
        n1273 = local read "Mirror task"() -> (w1927:refnum<k21>)
        n1274 = Cluster To Array(cluster="Trap position (V)") -> (array=w1930:dbl[])
        n1275 = Rotate 1D Array(1:w1930, 2:1 ("n")) -> (0:w1928:dbl[])
        n1276 = call-poly <vilib>:"DAQmx Write.vi"("task/channels in"=w1927, "data"=w1928) -> ("task out"=w1933:refnum<k21>, "error out"=w1932:errorcluster)  [unwired: 11 in, 1 out]
        n1277 = call <vilib>:"DAQmx Stop Task.vi"("task/channels in"=w1933, "error in"=w1932) -> ("error out"=w1931:errorcluster)  [unwired: 12 in, 1 out]
        n1278 = call <vilib>:"Simple Error Handler.vi"("error in (no error)"=w1931) -> ()  [unwired: 4 in, 5 out]
      }
      event "Trap delta (nm)": Value Change {
        n1279 = event-data() -> ()  [unwired: 1 in, 6 out]
        n1280 = local read "Pulling direction"() -> (w1935:bool)
        n1281 = local read "Conv Y (nm/V)"() -> (w1936:dbl)
        n1282 = local read "Conv X (nm/V)"() -> (w1937:dbl)
        n1283 = Select(t=w1936, s=w1935, f=w1937) -> (s? t:f=w1938:dbl)
        n1284 = local read "Fixed Y"() -> (w1944:dbl)
        n1285 = Divide(x="Trap delta (nm)", y=w1938) -> (x/y=w1939:dbl)
        n1286 = local read "Fixed X"() -> (w1943:dbl)
        n1287 = Select(t=w1944, s=w1935, f=w1943) -> (s? t:f=w1942:dbl)
        n1288 = Add(x=w1939, y=w1942) -> (x+y=w1940:dbl)
        n1289 = case shown="False" w1935 {
          tunnel: w1940 -> [w1945 w1946]
          frame False {
            n1290 = property on="X" class="DigNum (strict)"("Val(Sgnl)"=w1945) -> ()  [unwired: 2 in, 2 out]
          }
          frame True {
            n1291 = property on="Y" class="DigNum (strict)"("Val(Sgnl)"=w1946) -> ()  [unwired: 2 in, 2 out]
          }
        }
      }
      event "Fish": Value Change {
        n1292 = event-data() -> ()  [unwired: 1 in, 6 out]
        n1293 = local read "Fish"() -> (w1947:bool)
        n1294 = case shown="True" w1947 {
          frame False {
          }
          frame True {
            w1957 = 0.0 ("minimum value")
            w1958 = 10.0 ("maximum value")
            # "Grab offset in pulling\ndirection and add to \ndelta values"
            n1295 = call-poly <vilib>:"DAQmx Create Virtual Channel.vi"("maximum value"=w1958, "minimum value"=w1957, "physical channels"=tag "Dev1/ao0") -> ("task out"=w1962:refnum<k21>, "error out"=w1961:errorcluster)  [unwired: 11 in]
            n1296 = call-poly <vilib>:"DAQmx Create Virtual Channel.vi"("task in"=w1962, "maximum value"=w1958, "minimum value"=w1957, "physical channels"=tag "Dev1/ao1", "error in"=w1961) -> ("task out"=w1956:refnum<k21>, "error out"=w1955:errorcluster)  [unwired: 9 in]
            n1297 = node-c288(i64 1 ("Period")) -> (w1964:T13)  [unwired: 3 in]
            n1298 = timed-loop {
              timing: w1964 -> [_]
              timing-out: [_] -> w1963
              tunnel: w1956 -> [w2033]
              tunnel: w1955 -> [w2032]
              tunnel: [w2031] -> w1952
              tunnel: [w2030] -> w1951
              tunnel: [w1990] -> w1953
              tunnel: [w1991] -> w1950
              i -> [w2016]
              stop <- w1991 stop-if-true
              # "x direction"
              # "y direction"
              # "Send offset in direction\nof not-pulling to DAQ"
              n1299 = node-c288() -> ()  [unwired: 1 in, 1 out]
              n1300 = local read "Pulling direction"() -> (w1995:bool)
              n1301 = local read "Conv Y (nm/V)"() -> (w1997:dbl)
              n1302 = local read "Conv X (nm/V)"() -> (w1996:dbl)
              n1303 = local read "Fixed X"() -> (w2004:dbl)
              n1304 = local read "Fixed Y"() -> (w2003:dbl)
              n1305 = Select(t=w2003, s=w1995, f=w2004) -> (s? t:f=w2005:dbl)
              n1306 = Select(t=w2004, s=w1995, f=w2003) -> (s? t:f=w2002:dbl)
              n1307 = Select(t=w1997, s=w1995, f=w1996) -> (s? t:f=w1992:dbl)
              n1308 = Divide(x="Max fish\ndelta (nm)", y=w1992) -> (x/y=w1994:dbl)
              n1309 = Divide(x="Min fish\ndelta (nm)", y=w1992) -> (x/y=w1993:dbl)
              n1310 = Add(x=w2005, y=w1994) -> (x+y=w2007:dbl)
              n1311 = Subtract(x=w1994, y=w1993) -> (x-y=w2009:dbl)
              n1312 = Divide(x=w2009, y="Fish Speed (ms)") -> (x/y=w2010:dbl)
              n1313 = flat-sequence {
                tunnel: w1995 -> [w2053]
                tunnel: w2002 -> [w2052]
                tunnel: w2033 -> [w2051]
                tunnel: w2032 -> [w2050]
                tunnel: w2010 -> [w2049]
                tunnel: w2007 -> [w2048]
                tunnel: "Fish Speed (ms)" -> [w2043]
                tunnel: [w2047] -> w2029
                tunnel: [w2046] -> w2028
                tunnel: [w2045] -> w2027
                tunnel: [w2044] -> w2026
                tunnel: [w2037] -> w2015
                tunnel: [w2036] -> w2001
                tunnel: [w2035] -> w1998
                tunnel: [w2034] -> w1988
                tunnel: [w2106] -> w2025
                tunnel: w2029 -> [w2106]
                tunnel: [w2105] -> w2024
                tunnel: w2028 -> [w2105]
                tunnel: [w2104] -> w2023
                tunnel: w2027 -> [w2104]
                tunnel: [w2103] -> w2022
                tunnel: w2026 -> [w2103]
                tunnel: w2015 -> [w2102]
                tunnel: [w2102] -> w2014
                tunnel: w2001 -> [w2101]
                tunnel: [w2100] -> w1999
                tunnel: w1998 -> [w2100]
                tunnel: [w2099] -> w1989
                tunnel: w1988 -> [w2099]
                tunnel: w2025 -> [w2118]
                tunnel: w2024 -> [w2117]
                tunnel: w2023 -> [w2116]
                tunnel: w2022 -> [w2115]
                tunnel: w2012 -> [w2114]
                tunnel: [w2113] -> w2031
                tunnel: [w2112] -> w2030
                tunnel: w2014 -> [w2111]
                tunnel: [w2110] -> w2000
                tunnel: w1999 -> [w2109]
                tunnel: [w2108] -> w1987
                tunnel: w1989 -> [w2108]
                frame #0 {
                  n1314 = local read "Mean force (pN)"() -> (w2042:dbl)
                  n1315 = local read "Cutoff force (pN)"() -> (w2041:dbl)
                  n1316 = Less Or Equal?(x=w2042, y=w2041) -> (x <= y?=w2039:bool)
                  n1317 = And(x="Fish", y=w2039) -> (x .and. y?=w2040:bool)
                  n1318 = case shown="True" w2040 {
                    selector: w2040 -> [w2056 _]
                    tunnel: w2053 -> [w2059 w2076]
                    tunnel: w2052 -> [_ w2075]
                    tunnel: w2051 -> [w2061 w2074]
                    tunnel: w2050 -> [w2060 w2073]
                    tunnel: w2049 -> [w2058 w2072]
                    tunnel: w2048 -> [w2057 w2071]
                    tunnel: [w2061 w2070] -> w2047
                    tunnel: [w2060 w2069] -> w2046
                    tunnel: [w2059 w2068] -> w2045
                    tunnel: [w2057 w2067] -> w2035
                    tunnel: [w2058 w2066] -> w2044
                    tunnel: w2043 -> [_ w2065]
                    tunnel: [w2056 w2064] -> w2037
                    tunnel: [FALSE w2063] -> w2036
                    tunnel: [FALSE w2062] -> w2034
                    frame False {
                    }
                    frame True {
                      n1319 = while {
                        tunnel: w2076 -> [w2088]
                        tunnel: w2075 -> [w2087]
                        tunnel: w2074 -> [w2095]
                        tunnel: w2073 -> [w2094]
                        tunnel: w2072 -> [w2086]
                        tunnel: w2071 -> [w2092]
                        tunnel: [w2090] -> w2070
                        tunnel: [w2089] -> w2069
                        tunnel: [w2088] -> w2068
                        tunnel: [w2087] -> w2067
                        tunnel: [w2086] -> w2066
                        tunnel: w2065 -> [w2085]
                        tunnel: [w2078] -> w2064
                        tunnel: [w2078] -> w2063
                        tunnel: [w2077] -> w2062
                        i -> [w2084]
                        stop <- w2081 stop-if-true
                        # "top: x"
                        # "x direction"
                        # "y direction"
                        n1320 = Multiply(x=w2086, y=w2084) -> (x*y=w2093:dbl)
                        n1321 = local read "Cutoff force (pN)"() -> (w2079:dbl)
                        n1322 = local read "Mean force (pN)"() -> (w2080:dbl)
                        n1323 = Subtract(x=w2092, y=w2093) -> (x-y=w2091:dbl)
                        n1324 = Build Array(w2087, w2091) -> (w2098:dbl[])
                        n1325 = Build Array(w2091, w2087) -> (w2097:dbl[])
                        n1326 = Greater Or Equal?(x=w2084, y=w2085) -> (x >= y?=w2078:bool)
                        n1327 = Select(t=w2098, s=w2088, f=w2097) -> (s? t:f=w2096:dbl[])
                        n1328 = Greater?(x=w2080, y=w2079) -> (0:w2077:bool)
                        n1329 = local read "Fish"() -> (w2082:bool)
                        n1330 = Not(x=w2082) -> (.not. x?=w2083:bool)
                        n1331 = call-poly <vilib>:"DAQmx Write.vi"("task/channels in"=w2095, "data"=w2096, "error in"=w2094) -> ("task out"=w2090:refnum<k21>, "error out"=w2089:errorcluster)  [unwired: 10 in, 1 out]
                        n1332 = Compound Arithmetic op=OR(w2078, w2083, w2077) -> (w2081:bool)
                      }
                    }
                  }
                }
                frame #1 {
                  n1333 = case shown="True" w2101 {
                    frame False {
                    }
                    frame True {
                      n1334 = Wait (ms)(milliseconds to wait="Wait (ms)") -> ()  [unwired: 1 out]
                    }
                  }
                }
                frame #2 {
                  n1335 = case shown="True" w2111 {
                    tunnel: w2118 -> [w2121 w2130]
                    tunnel: w2117 -> [w2120 w2129]
                    tunnel: w2116 -> [_ w2128]
                    tunnel: w2115 -> [_ w2127]
                    tunnel: w2114 -> [_ w2126]
                    tunnel: [w2121 w2125] -> w2113
                    tunnel: [w2120 w2124] -> w2112
                    tunnel: [FALSE w2123] -> w2110
                    tunnel: w2109 -> [_ w2122]
                    frame False {
                    }
                    frame True {
                      n1336 = while {
                        tunnel: w2130 -> [w2162]
                        tunnel: w2129 -> [w2161]
                        tunnel: w2128 -> [w2133]
                        tunnel: w2127 -> [w2159]
                        tunnel: w2126 -> [w2158]
                        tunnel: [w2156] -> w2125
                        tunnel: [w2155] -> w2124
                        tunnel: [w2140] -> w2123
                        tunnel: w2122 -> [w2131]
                        i -> [w2147]
                        stop <- w2152 stop-if-true
                        # "y direction"
                        # "If tether formed,\nimmediately change\nto new delta."
                        n1337 = local read "Conv Y (nm/V)"() -> (w2134:dbl)
                        n1338 = local read "Conv X (nm/V)"() -> (w2132:dbl)
                        n1339 = local read "Fixed Y"() -> (w2141:dbl)
                        n1340 = local read "Fixed X"() -> (w2146:dbl)
                        n1341 = Select(t=w2134, s=w2133, f=w2132) -> (s? t:f=w2135:dbl)
                        n1342 = local read "Cutoff force (pN)"() -> (w2148:dbl)
                        n1343 = Divide(x="Delta after tether", y=w2135) -> (x/y=w2136:dbl)
                        n1344 = Multiply(x=w2159, y=w2147) -> (x*y=w2160:dbl)
                        n1345 = local read "Mean force (pN)"() -> (w2149:dbl)
                        n1346 = Add(x=w2158, y=w2160) -> (x+y=w2143:dbl)
                        n1347 = Select(t=w2141, s=w2133, f=w2146) -> (s? t:f=w2145:dbl)
                        n1348 = Greater?(x=w2149, y=w2148) -> (0:w2140:bool)
                        n1349 = Add(x=w2145, y=w2136) -> (x+y=w2144:dbl)
                        n1350 = Select(t=w2144, s=w2140, f=w2143) -> (s? t:f=w2142:dbl)
                        n1351 = local read "Fish Speed (ms)"() -> (w2154:i32)
                        n1352 = Build Array(w2131, w2142) -> (w2157:dbl[])
                        n1353 = Build Array(w2142, w2131) -> (w2138:dbl[])
                        n1354 = Select(t=w2157, s=w2133, f=w2138) -> (s? t:f=w2137:dbl[])
                        n1355 = case shown="True" w2140 {
                          tunnel: w2136 -> [_ _]
                          tunnel: w2137 -> [_ w2164]
                          frame False {
                          }
                          frame True {
                            n1356 = Array To Cluster(array=w2164) -> (cluster=w2163:cluster{"[0]":dbl, "[1]":dbl})
                            n1357 = property on="Trap position (V)" class="Clust (strict)"("Val(Sgnl)"=w2163) -> ()  [unwired: 2 in, 2 out]
                          }
                        }
                        n1358 = local read "Fish"() -> (w2151:bool)
                        n1359 = Greater Or Equal?(x=w2147, y=w2154) -> (x >= y?=w2153:bool)
                        n1360 = Not(x=w2151) -> (.not. x?=w2150:bool)
                        n1361 = call-poly <vilib>:"DAQmx Write.vi"("task/channels in"=w2162, "data"=w2137, "error in"=w2161) -> ("task out"=w2156:refnum<k21>, "error out"=w2155:errorcluster)  [unwired: 10 in, 1 out]
                        n1362 = Compound Arithmetic op=OR(w2153, w2150, w2140) -> (w2152:bool)
                      }
                    }
                  }
                }
              }
              n1363 = Add(x=w2005, y=w1993) -> (x+y=w2012:dbl)
              n1364 = Decrement(x="# attempts") -> (x-1=w2020:dbl)
              n1365 = Greater Or Equal?(x=w2016, y=w2020) -> (x >= y?=w2019:bool)
              n1366 = local read "Mean force (pN)"() -> (w2018:dbl)
              n1367 = Greater?(x=w2018, y="Cutoff force (pN)") -> (0:w2013:bool)
              n1368 = Compound Arithmetic op=OR(w1987, w2000, w2013, w2019) -> (w1991:bool)
              n1369 = Or(x=w2000, y=w1987) -> (x .or. y?=w1990:bool)
              "Tether" <- w1990
              n1370 = case shown="True" w1990 {
                frame False {
                }
                frame True {
                  n1371 = call <vilib>:"Beep.vi"() -> ()  [unwired: 12 in]
                }
              }
              n1372 = node-c288() -> ()  [unwired: 1 in, 1 out]
              "Attempt #" <- w2016
            }
            n1373 = node-c288(w1963) -> ()  [unwired: 1 out]
            n1374 = flat-sequence {
              tunnel: w1953 -> [w1971]
              tunnel: [w1971] -> w1949
              tunnel: w1952 -> [w1968]
              tunnel: w1951 -> [w1967]
              tunnel: w1950 -> [w1965]
              tunnel: w1949 -> [w1973]
              tunnel: [w1973] -> w1948
              tunnel: w1948 -> [w1975]
              frame #0 {
                w1970 = T24 1 items=["no dialog", "OK message", "continue or stop message", "OK message + warnings", "continue/stop + warnings"] ("type of dialog (OK msg:1)")
                n1375 = call <vilib>:"DAQmx Clear Task.vi"("task in"=w1968, "error in"=w1967) -> ("error out"=w1969:errorcluster)  [unwired: 13 in]
                n1376 = Not(x=w1965) -> (.not. x?=w1966:bool)
                n1377 = local write "Fish"(w1966) -> ()
                n1378 = call <vilib>:"Simple Error Handler.vi"("type of dialog (OK msg:1)"=w1970, "error in (no error)"=w1969) -> ()  [unwired: 3 in, 5 out]
              }
              frame #1 {
                n1379 = Wait (ms)(milliseconds to wait=u32 500) -> ()  [unwired: 1 out]
              }
              frame #2 {
                n1380 = And(x=w1975, y="Raster after\n tether?") -> (x .and. y?=w1976:bool)
                n1381 = case shown="True" w1976 {
                  selector: w1976 -> [_ w1977]
                  frame False {
                  }
                  frame True {
                    n1382 = stacked-sequence {
                      tunnel: w1977 -> [_ _ _ _ w1986]
                      frame #0 {
                        n1383 = local read "Raster set"() -> (w1981:i32)
                        n1384 = property on="Inject Sample" class="Bool (strict)"("Val(Sgnl)"=FALSE ("Value (Signaling)")) -> ()  [unwired: 2 in, 2 out]
                        n1385 = Replace Array Subset(array=i32[] [0], new element=w1981, index=0) -> (w1978:i32[])
                        n1386 = property on="Scan Parameters" class="Arr (strict)"("Index Values"=w1978) -> ()  [unwired: 2 in, 2 out]
                      }
                      frame #1 {
                        n1387 = Wait (ms)(milliseconds to wait=u32 500) -> ()  [unwired: 1 out]
                      }
                      frame #2 {
                        n1388 = property on="Load param" class="Bool (strict)"("Val(Sgnl)"=TRUE ("Value (Signaling)")) -> ()  [unwired: 2 in, 2 out]
                      }
                      frame #3 {
                        n1389 = Wait (ms)(milliseconds to wait=u32 500) -> ()  [unwired: 1 out]
                      }
                      frame #4 {
                        n1390 = property on="Raster scan" class="Bool (strict)"("Val(Sgnl)"=w1986) -> ()  [unwired: 2 in, 2 out]
                      }
                    }
                  }
                }
              }
            }
          }
        }
      }
      event "Load param": Value Change {
        n1391 = event-data() -> ()  [unwired: 1 in, 6 out]
        n1392 = property on="Scan Parameters" class="Arr (strict)"() -> ("Index Values"=w2180:u32[])  [unwired: 2 in, 2 out]
        n1393 = Index Array(array=w2180, index=0) -> (element=w2177:u32)
        n1394 = Index Array(array="Scan Parameters", index=w2177) -> (element=w2176:T27)
        n1395 = Unbundle(w2176) -> ("Scan range 1"=w2174:dbl, "Step size 1"=w2173:dbl, "Scan speed 1"=w2171:i32, "# scans 2"=w2172:i32)  [unwired: 1 out]
        n1396 = property on="# scans" class="DigNum (strict)"("Val(Sgnl)"=w2172) -> ()  [unwired: 2 in, 2 out]
        n1397 = property on="Scan range (nm)" class="DigNum (strict)"("Val(Sgnl)"=w2174) -> ()  [unwired: 2 in, 2 out]
        n1398 = property on="Step size 1" class="DigNum (strict)"("Val(Sgnl)"=w2173) -> ()  [unwired: 2 in, 2 out]
        n1399 = property on="Scan speed (nm/s)" class="DigNum (strict)"("Val(Sgnl)"=w2171) -> ()  [unwired: 2 in, 2 out]
        n1400 = local write "Load param"(FALSE ("Load param")) -> ()
      }
      event "# scans", "Scan range (nm)", "Step size (nm)", "Scan speed (nm/s)": Value Change {
        n1401 = event-data() -> ()  [unwired: 1 in, 6 out]
        n1402 = local read "Pulling direction"() -> (w2211:bool)
        n1403 = Reciprocal(x="Scan speed (nm/s)") -> (1/x=w2203:dbl)
        n1404 = local read "Conv Y (nm/V)"() -> (w2209:dbl)
        n1405 = local read "Conv X (nm/V)"() -> (w2210:dbl)
        n1406 = Multiply(x="Step size (nm)", y=w2203) -> (x*y=w2201:dbl)
        n1407 = Divide(x="Scan range (nm)", y="Step size (nm)") -> (x/y=w2208:dbl)
        n1408 = Absolute Value(x=w2208) -> (abs(x)=w2207:dbl)
        n1409 = Multiply(x=w2201, y=1000.0) -> (x*y=w2188:dbl)
        n1410 = Select(t=w2209, s=w2211, f=w2210) -> (s? t:f=w2199:dbl)
        n1411 = Multiply(x="# scans", y=2) -> (x*y=w2187:i32)
        n1412 = To Unsigned Quad Integer(1:w2207) -> (0:w2197:u64)
        "Scan steps (mirror)" <- w2197
        n1413 = Divide(x="Scan range (nm)", y=w2199) -> (x/y=→"Scan range (V)":dbl)
        n1414 = Multiply(x=w2197, y=w2188) -> (x*y=w2196:dbl)
        n1415 = Divide(x="Step size (nm)", y=w2199) -> (x/y=→"Scan increment (V)":dbl)
        n1416 = Round Toward +Infinity(x=w2188) -> (ceil(x): smallest int >= x=w2185:dbl)
        "Time per step (ms)" <- w2185
        n1417 = local read "Data update period (s/set)"() -> (w2191:dbl)
        n1418 = Multiply(x=w2187, y=w2196) -> (x*y=w2194:dbl)
        n1419 = Divide(x=w2194, y=1000.0) -> (x/y=w2192:dbl)
        "Total raster time (s)" <- w2192
        n1420 = local read "Data update period (s/set)"() -> (w2183:dbl)
        n1421 = Divide(x=w2192, y=w2191) -> (x/y=w2190:dbl)
        n1422 = Round Toward -Infinity(1:w2190) -> (0:→"N sets to be saved":dbl)
        n1423 = Multiply(x=w2183, y=1000.0) -> (x*y=w2181:dbl)
        n1424 = Less?(x=w2185, y=w2181) -> (x < y?=w2184:bool)
        n1425 = case shown="True" w2184 {
          selector: w2184 -> [_ w2212]
          frame False {
          }
          frame True {
            n1426 = call "Display Message to User"("Enable"=w2212) -> ()  [unwired: 9 in, 2 out]
          }
        }
      }
      event "Pulling direction": Value Change {
        n1427 = event-data() -> ()  [unwired: 1 in, 6 out]
        n1428 = local read "Pulling direction"() -> (w2218:bool)
        n1429 = local read "Conv Y (nm/V)"() -> (w2220:dbl)
        n1430 = local read "Conv X (nm/V)"() -> (w2219:dbl)
        n1431 = local read "Scan range (nm)"() -> (w2217:dbl)
        n1432 = Select(t=w2220, s=w2218, f=w2219) -> (s? t:f=w2214:dbl)
        n1433 = local read "Step size (nm)"() -> (w2215:dbl)
        n1434 = case shown="False" w2218 {
          frame False {
            n1435 = local read "Fixed Y"() -> (w2223:dbl)
            n1436 = local read "Trap delta (nm)"() -> (w2228:dbl)
            n1437 = local read "Conv X (nm/V)"() -> (w2227:dbl)
            n1438 = local read "Fixed X"() -> (w2225:dbl)
            n1439 = Divide(x=w2228, y=w2227) -> (x/y=w2226:dbl)
            n1440 = Add(x=w2226, y=w2225) -> (x+y=w2224:dbl)
            n1441 = Build Array(w2224, w2223) -> (w2222:dbl[])
            n1442 = Array To Cluster(array=w2222) -> (cluster=w2221:cluster{"[0]":dbl, "[1]":dbl})
            n1443 = property on="Trap position (V)" class="Clust (strict)"("Val(Sgnl)"=w2221) -> ()  [unwired: 2 in, 2 out]
          }
          frame True {
            n1444 = local read "Trap delta (nm)"() -> (w2236:dbl)
            n1445 = local read "Conv Y (nm/V)"() -> (w2235:dbl)
            n1446 = local read "Fixed X"() -> (w2231:dbl)
            n1447 = local read "Fixed Y"() -> (w2233:dbl)
            n1448 = Divide(x=w2236, y=w2235) -> (x/y=w2234:dbl)
            n1449 = Add(x=w2234, y=w2233) -> (x+y=w2232:dbl)
            n1450 = Build Array(w2231, w2232) -> (w2230:dbl[])
            n1451 = Array To Cluster(array=w2230) -> (cluster=w2229:cluster{"[0]":dbl, "[1]":dbl})
            n1452 = property on="Trap position (V)" class="Clust (strict)"("Val(Sgnl)"=w2229) -> ()  [unwired: 2 in, 2 out]
          }
        }
        n1453 = Divide(x=w2217, y=w2214) -> (x/y=w2216:dbl)
        n1454 = Divide(x=w2215, y=w2214) -> (x/y=w2213:dbl)
        n1455 = local write "Scan range (V)"(w2216) -> ()
        n1456 = local write "Scan increment (V)"(w2213) -> ()
      }
      event "Averaging Number": Value Change {
        n1457 = event-data() -> ()  [unwired: 1 in, 6 out]
        n1458 = local read "# Samples/channel (in)"() -> (w2240:i32)
        n1459 = local read "Averaging Number"() -> (w2238:i32)
        n1460 = Quotient & Remainder(x=w2240, y=w2238) -> (floor(x/y)=w2239:i32)  [unwired: 1 out]
        n1461 = Multiply(x=w2239, y=w2238) -> (x*y=w2237:i32)
        n1462 = local write "# Samples/channel (in)"(w2237) -> ()
      }
    }
    n1463 = node-c288() -> ()  [unwired: 1 in, 1 out]
  }
  n1464 = VISA Close(VISA resource name=w27) -> (error out=w105:errorcluster)  [unwired: 1 in]
  n1465 = call <vilib>:"Simple Error Handler.vi"("error in (no error)"=w105) -> ()  [unwired: 4 in, 5 out]
  n1466 = disable-structure shown="Enabled" {
    frame Disabled {
      n1467 = node-c288(2 ("Processor")) -> (w2246:T13)  [unwired: 3 in]
      n1468 = timed-loop "Pump Control" {
        timing: w2246 -> [_]
        timing-out: [_] -> w2245
        tunnel: refnum<visa-resource-name> "COM6" ("VISA resource name") -> [w2248]
        stop <- w2247 stop-if-true
        n1469 = node-c288() -> ()  [unwired: 1 in, 1 out]
        n1470 = event shown="[4] \"Inject Pump 1\": Value Change" {
          selector: _ -> [_ _ _ _ _ _ _ _ _]
          dyn-events: _ -> [_ _ _ _ _ _ _ _ _]
          timeout: _ -> [_ _ _ _ _ _ _ _ _]
          tunnel: w2248 -> [w2256 w2352 _ w2428 w2556 w2699 w2744 w2802 w2861]
          tunnel: [_ _ w2427 _ _ _ _ _ _] -> w2247
          event "Flush Pump 1": Value Change {
            w2257 = "\r"
            n1471 = event-data() -> ()  [unwired: 1 in, 5 out]
            n1472 = call-poly "VISA Configure Serial Port"("VISA resource name"=w2256) -> ("VISA resource name out"=w2270:refnum<visa-resource-name>, "error out"=w2271:errorcluster)  [unwired: 13 in]
            n1473 = local read "Write Wait"() -> (w2249:i32)
            n1474 = Concatenate Strings("enter pump1", w2257) -> (w2258:string)
            n1475 = flat-sequence {
              tunnel: w2271 -> [w2290]
              tunnel: w2270 -> [w2292]
              tunnel: [w2291] -> w2287
              tunnel: [w2289] -> w2286
              tunnel: w2258 -> [w2288]
              tunnel: w2287 -> [w2295]
              tunnel: [w2295] -> w2285
              tunnel: w2286 -> [w2294]
              tunnel: [w2294] -> w2284
              tunnel: w2249 -> [w2293]
              tunnel: [w2300] -> w2283
              tunnel: w2263 -> [w2299]
              tunnel: [w2296] -> w2282
              tunnel: w2285 -> [w2298]
              tunnel: w2284 -> [w2297]
              tunnel: w2283 -> [w2303]
              tunnel: [w2303] -> w2281
              tunnel: [w2302] -> w2280
              tunnel: w2282 -> [w2302]
              tunnel: w2249 -> [w2301]
              tunnel: w2281 -> [w2308]
              tunnel: [w2307] -> w2279
              tunnel: w2266 -> [w2306]
              tunnel: w2280 -> [w2305]
              tunnel: [w2304] -> w2278
              tunnel: w2279 -> [w2311]
              tunnel: [w2311] -> w2277
              tunnel: [w2310] -> w2276
              tunnel: w2278 -> [w2310]
              tunnel: w2249 -> [w2309]
              tunnel: w2277 -> [w2316]
              tunnel: [w2315] -> w2275
              tunnel: w2269 -> [w2314]
              tunnel: w2276 -> [w2313]
              tunnel: [w2312] -> w2274
              tunnel: [w2319] -> w2273
              tunnel: w2275 -> [w2319]
              tunnel: [w2318] -> w2272
              tunnel: w2274 -> [w2318]
              tunnel: w2249 -> [w2317]
              tunnel: w2273 -> [w2324]
              tunnel: w2272 -> [w2321]
              tunnel: [w2323] -> w2252
              tunnel: [w2322] -> w2250
              tunnel: [w2329] -> w2253
              tunnel: w2252 -> [w2329]
              tunnel: [w2328] -> w2251
              tunnel: w2250 -> [w2328]
              tunnel: w2249 -> [w2327]
              tunnel: w2253 -> [w2331]
              tunnel: w2251 -> [w2330]
              frame #0 {
                n1476 = VISA Write(VISA resource name=w2292, write buffer=w2288, error in (no error)=w2290) -> (VISA resource name out=w2291:refnum<visa-resource-name>, error out=w2289:errorcluster)  [unwired: 1 out]
              }
              frame #1 {
                n1477 = Wait (ms)(milliseconds to wait=w2293) -> ()  [unwired: 1 out]
              }
              frame #2 {
                n1478 = VISA Write(VISA resource name=w2298, write buffer=w2299, error in (no error)=w2297) -> (VISA resource name out=w2300:refnum<visa-resource-name>, error out=w2296:errorcluster)  [unwired: 1 out]
              }
              frame #3 {
                n1479 = Wait (ms)(milliseconds to wait=w2301) -> ()  [unwired: 1 out]
              }
              frame #4 {
                n1480 = VISA Write(VISA resource name=w2308, write buffer=w2306, error in (no error)=w2305) -> (VISA resource name out=w2307:refnum<visa-resource-name>, error out=w2304:errorcluster)  [unwired: 1 out]
              }
              frame #5 {
                n1481 = Wait (ms)(milliseconds to wait=w2309) -> ()  [unwired: 1 out]
              }
              frame #6 {
                n1482 = VISA Write(VISA resource name=w2316, write buffer=w2314, error in (no error)=w2313) -> (VISA resource name out=w2315:refnum<visa-resource-name>, error out=w2312:errorcluster)  [unwired: 1 out]
              }
              frame #7 {
                n1483 = Wait (ms)(milliseconds to wait=w2317) -> ()  [unwired: 1 out]
              }
              frame #8 {
                n1484 = Concatenate Strings("start ", "\r") -> (w2320:string)
                n1485 = VISA Write(VISA resource name=w2324, write buffer=w2320, error in (no error)=w2321) -> (VISA resource name out=w2323:refnum<visa-resource-name>, error out=w2322:errorcluster)  [unwired: 1 out]
              }
              frame #9 {
                n1486 = Wait (ms)(milliseconds to wait=w2327) -> ()  [unwired: 1 out]
              }
              frame #10 {
                n1487 = local write "Flush Pump 1"(FALSE ("Flush Pump 1")) -> ()
                n1488 = Concatenate Strings("enter main ", "\r") -> (w2335:string)
                n1489 = VISA Write(VISA resource name=w2331, write buffer=w2335, error in (no error)=w2330) -> (VISA resource name out=w2334:refnum<visa-resource-name>, error out=w2333:errorcluster)  [unwired: 1 out]
                n1490 = VISA Close(VISA resource name=w2334, error in (no error)=w2333) -> ()  [unwired: 1 out]
              }
            }
            n1491 = Concatenate Strings("set units 4 ", w2257) -> (w2263:string)
            n1492 = Multiply(x="Flush\nRate (ul/min)", y=60) -> (x*y=w2261:dbl)
            n1493 = Number To Decimal String(number=w2261) -> (decimal integer string=w2264:string)  [unwired: 1 in]
            n1494 = Concatenate Strings("set rate ", w2264, w2257) -> (w2266:string)
            n1495 = Number To Decimal String(number="Flush\nVolume (ul)") -> (decimal integer string=w2268:string)  [unwired: 1 in]
            n1496 = Concatenate Strings("set volume ", w2268, w2257) -> (w2269:string)
          }
          event "Flush Pump 2": Value Change {
            w2343 = "\r"
            n1497 = event-data() -> ()  [unwired: 1 in, 5 out]
            n1498 = call-poly "VISA Configure Serial Port"("VISA resource name"=w2352) -> ("VISA resource name out"=w2363:refnum<visa-resource-name>, "error out"=w2364:errorcluster)  [unwired: 13 in]
            n1499 = local read "Write Wait"() -> (w2338:i32)
            n1500 = Concatenate Strings("enter pump2", w2343) -> (w2344:string)
            n1501 = flat-sequence {
              tunnel: w2364 -> [w2379]
              tunnel: w2363 -> [w2381]
              tunnel: [w2380] -> w2349
              tunnel: [w2378] -> w2347
              tunnel: w2344 -> [w2377]
              tunnel: w2349 -> [w2384]
              tunnel: [w2384] -> w2348
              tunnel: w2347 -> [w2383]
              tunnel: [w2383] -> w2346
              tunnel: w2338 -> [w2382]
              tunnel: [w2389] -> w2376
              tunnel: w2356 -> [w2388]
              tunnel: [w2385] -> w2375
              tunnel: w2348 -> [w2387]
              tunnel: w2346 -> [w2386]
              tunnel: w2376 -> [w2392]
              tunnel: [w2392] -> w2374
              tunnel: [w2391] -> w2373
              tunnel: w2375 -> [w2391]
              tunnel: w2338 -> [w2390]
              tunnel: w2374 -> [w2397]
              tunnel: [w2396] -> w2372
              tunnel: w2359 -> [w2395]
              tunnel: w2373 -> [w2394]
              tunnel: [w2393] -> w2371
              tunnel: w2372 -> [w2400]
              tunnel: [w2400] -> w2370
              tunnel: [w2399] -> w2369
              tunnel: w2371 -> [w2399]
              tunnel: w2338 -> [w2398]
              tunnel: w2370 -> [w2405]
              tunnel: [w2404] -> w2368
              tunnel: w2362 -> [w2403]
              tunnel: w2369 -> [w2402]
              tunnel: [w2401] -> w2367
              tunnel: [w2408] -> w2366
              tunnel: w2368 -> [w2408]
              tunnel: [w2407] -> w2365
              tunnel: w2367 -> [w2407]
              tunnel: w2338 -> [w2406]
              tunnel: w2366 -> [w2415]
              tunnel: w2365 -> [w2414]
              tunnel: [w2410] -> w2342
              tunnel: [w2409] -> w2340
              tunnel: w2342 -> [w2418]
              tunnel: [w2418] -> w2341
              tunnel: w2340 -> [w2417]
              tunnel: [w2417] -> w2339
              tunnel: w2338 -> [w2416]
              tunnel: w2341 -> [w2422]
              tunnel: w2339 -> [w2421]
              frame #0 {
                n1502 = VISA Write(VISA resource name=w2381, write buffer=w2377, error in (no error)=w2379) -> (VISA resource name out=w2380:refnum<visa-resource-name>, error out=w2378:errorcluster)  [unwired: 1 out]
              }
              frame #1 {
                n1503 = Wait (ms)(milliseconds to wait=w2382) -> ()  [unwired: 1 out]
              }
              frame #2 {
                n1504 = VISA Write(VISA resource name=w2387, write buffer=w2388, error in (no error)=w2386) -> (VISA resource name out=w2389:refnum<visa-resource-name>, error out=w2385:errorcluster)  [unwired: 1 out]
              }
              frame #3 {
                n1505 = Wait (ms)(milliseconds to wait=w2390) -> ()  [unwired: 1 out]
              }
              frame #4 {
                n1506 = VISA Write(VISA resource name=w2397, write buffer=w2395, error in (no error)=w2394) -> (VISA resource name out=w2396:refnum<visa-resource-name>, error out=w2393:errorcluster)  [unwired: 1 out]
              }
              frame #5 {
                n1507 = Wait (ms)(milliseconds to wait=w2398) -> ()  [unwired: 1 out]
              }
              frame #6 {
                n1508 = VISA Write(VISA resource name=w2405, write buffer=w2403, error in (no error)=w2402) -> (VISA resource name out=w2404:refnum<visa-resource-name>, error out=w2401:errorcluster)  [unwired: 1 out]
              }
              frame #7 {
                n1509 = Wait (ms)(milliseconds to wait=w2406) -> ()  [unwired: 1 out]
              }
              frame #8 {
                n1510 = Concatenate Strings("start ", "\r") -> (w2413:string)
                n1511 = VISA Write(VISA resource name=w2415, write buffer=w2413, error in (no error)=w2414) -> (VISA resource name out=w2410:refnum<visa-resource-name>, error out=w2409:errorcluster)  [unwired: 1 out]
              }
              frame #9 {
                n1512 = Wait (ms)(milliseconds to wait=w2416) -> ()  [unwired: 1 out]
              }
              frame #10 {
                n1513 = local write "Flush Pump 2"(FALSE ("Flush Pump 1")) -> ()
                n1514 = Concatenate Strings("enter main ", "\r") -> (w2423:string)
                n1515 = VISA Write(VISA resource name=w2422, write buffer=w2423, error in (no error)=w2421) -> (VISA resource name out=w2420:refnum<visa-resource-name>, error out=w2419:errorcluster)  [unwired: 1 out]
                n1516 = VISA Close(VISA resource name=w2420, error in (no error)=w2419) -> ()  [unwired: 1 out]
              }
            }
            n1517 = Concatenate Strings("set units 4 ", w2343) -> (w2356:string)
            n1518 = Multiply(x="Flush \nRate (ul/min)  2", y=60) -> (x*y=w2354:dbl)
            n1519 = Number To Decimal String(number=w2354) -> (decimal integer string=w2357:string)  [unwired: 1 in]
            n1520 = Concatenate Strings("set rate ", w2357, w2343) -> (w2359:string)
            n1521 = Number To Decimal String(number="Flush\nVolume (ul)  2") -> (decimal integer string=w2361:string)  [unwired: 1 in]
            n1522 = Concatenate Strings("set volume ", w2361, w2343) -> (w2362:string)
          }
          event "Stop": Value Change {
            n1523 = event-data() -> ()  [unwired: 1 in, 5 out]
            n1524 = local read "Stop"() -> (w2427:bool)
          }
          event "Inject Pump 2": Value Change {
            n1525 = event-data() -> ()  [unwired: 1 in, 5 out]
            n1526 = case shown="True" "Inject Pump 2" {
              tunnel: w2428 -> [w2431 w2473]
              frame False {
                n1527 = local read "Write Wait"() -> (w2430:i32)
                n1528 = call-poly "VISA Configure Serial Port"("VISA resource name"=w2431) -> ("VISA resource name out"=w2435:refnum<visa-resource-name>, "error out"=w2436:errorcluster)  [unwired: 13 in]
                n1529 = Concatenate Strings("enter pump2", "\r") -> (w2433:string)
                n1530 = flat-sequence {
                  tunnel: w2436 -> [w2447]
                  tunnel: w2435 -> [w2449]
                  tunnel: [w2448] -> w2444
                  tunnel: [w2446] -> w2443
                  tunnel: w2433 -> [w2445]
                  tunnel: w2444 -> [w2452]
                  tunnel: w2443 -> [w2451]
                  tunnel: [w2452] -> w2442
                  tunnel: [w2451] -> w2441
                  tunnel: w2430 -> [w2450]
                  tunnel: [w2456] -> w2440
                  tunnel: [w2455] -> w2439
                  tunnel: w2442 -> [w2454]
                  tunnel: w2441 -> [w2453]
                  tunnel: w2440 -> [w2462]
                  tunnel: [w2462] -> w2438
                  tunnel: w2439 -> [w2461]
                  tunnel: [w2461] -> w2437
                  tunnel: w2430 -> [w2460]
                  tunnel: w2438 -> [w2466]
                  tunnel: w2437 -> [w2465]
                  frame #0 {
                    n1531 = VISA Write(VISA resource name=w2449, write buffer=w2445, error in (no error)=w2447) -> (VISA resource name out=w2448:refnum<visa-resource-name>, error out=w2446:errorcluster)  [unwired: 1 out]
                  }
                  frame #1 {
                    n1532 = Wait (ms)(milliseconds to wait=w2450) -> ()  [unwired: 1 out]
                  }
                  frame #2 {
                    n1533 = Concatenate Strings("stop ", "\r") -> (w2459:string)
                    n1534 = VISA Write(VISA resource name=w2454, write buffer=w2459, error in (no error)=w2453) -> (VISA resource name out=w2456:refnum<visa-resource-name>, error out=w2455:errorcluster)  [unwired: 1 out]
                  }
                  frame #3 {
                    n1535 = Wait (ms)(milliseconds to wait=w2460) -> ()  [unwired: 1 out]
                  }
                  frame #4 {
                    n1536 = Concatenate Strings("enter main ", "\r") -> (w2467:string)
                    n1537 = VISA Write(VISA resource name=w2466, write buffer=w2467, error in (no error)=w2465) -> (VISA resource name out=w2464:refnum<visa-resource-name>, error out=w2463:errorcluster)  [unwired: 1 out]
                    n1538 = VISA Close(VISA resource name=w2464, error in (no error)=w2463) -> ()  [unwired: 1 out]
                  }
                }
              }
              frame True {
                w2486 = "\r"
                n1539 = call-poly "VISA Configure Serial Port"("VISA resource name"=w2473) -> ("VISA resource name out"=w2475:refnum<visa-resource-name>, "error out"=w2474:errorcluster)  [unwired: 13 in]
                n1540 = local read "Write Wait"() -> (w2470:i32)
                n1541 = Concatenate Strings("enter pump2", w2486) -> (w2485:string)
                n1542 = flat-sequence {
                  tunnel: w2474 -> [w2509]
                  tunnel: w2475 -> [w2511]
                  tunnel: [w2510] -> w2506
                  tunnel: [w2508] -> w2505
                  tunnel: w2485 -> [w2507]
                  tunnel: w2506 -> [w2514]
                  tunnel: [w2514] -> w2504
                  tunnel: w2505 -> [w2513]
                  tunnel: [w2513] -> w2503
                  tunnel: w2470 -> [w2512]
                  tunnel: [w2519] -> w2502
                  tunnel: w2482 -> [w2518]
                  tunnel: [w2515] -> w2501
                  tunnel: w2504 -> [w2517]
                  tunnel: w2503 -> [w2516]
                  tunnel: w2502 -> [w2522]
                  tunnel: [w2522] -> w2500
                  tunnel: [w2521] -> w2499
                  tunnel: w2501 -> [w2521]
                  tunnel: w2470 -> [w2520]
                  tunnel: w2500 -> [w2527]
                  tunnel: [w2526] -> w2498
                  tunnel: w2479 -> [w2525]
                  tunnel: w2499 -> [w2524]
                  tunnel: [w2523] -> w2497
                  tunnel: w2498 -> [w2530]
                  tunnel: [w2530] -> w2496
                  tunnel: [w2529] -> w2495
                  tunnel: w2497 -> [w2529]
                  tunnel: w2470 -> [w2528]
                  tunnel: w2496 -> [w2535]
                  tunnel: [w2534] -> w2494
                  tunnel: w2476 -> [w2533]
                  tunnel: w2495 -> [w2532]
                  tunnel: [w2531] -> w2493
                  tunnel: [w2538] -> w2492
                  tunnel: w2494 -> [w2538]
                  tunnel: [w2537] -> w2491
                  tunnel: w2493 -> [w2537]
                  tunnel: w2470 -> [w2536]
                  tunnel: w2492 -> [w2545]
                  tunnel: w2491 -> [w2544]
                  tunnel: [w2540] -> w2490
                  tunnel: [w2539] -> w2489
                  tunnel: w2490 -> [w2548]
                  tunnel: [w2548] -> w2488
                  tunnel: w2489 -> [w2547]
                  tunnel: [w2547] -> w2487
                  tunnel: w2470 -> [w2546]
                  tunnel: w2488 -> [w2552]
                  tunnel: w2487 -> [w2551]
                  frame #0 {
                    n1543 = VISA Write(VISA resource name=w2511, write buffer=w2507, error in (no error)=w2509) -> (VISA resource name out=w2510:refnum<visa-resource-name>, error out=w2508:errorcluster)  [unwired: 1 out]
                  }
                  frame #1 {
                    n1544 = Wait (ms)(milliseconds to wait=w2512) -> ()  [unwired: 1 out]
                  }
                  frame #2 {
                    n1545 = VISA Write(VISA resource name=w2517, write buffer=w2518, error in (no error)=w2516) -> (VISA resource name out=w2519:refnum<visa-resource-name>, error out=w2515:errorcluster)  [unwired: 1 out]
                  }
                  frame #3 {
                    n1546 = Wait (ms)(milliseconds to wait=w2520) -> ()  [unwired: 1 out]
                  }
                  frame #4 {
                    n1547 = VISA Write(VISA resource name=w2527, write buffer=w2525, error in (no error)=w2524) -> (VISA resource name out=w2526:refnum<visa-resource-name>, error out=w2523:errorcluster)  [unwired: 1 out]
                  }
                  frame #5 {
                    n1548 = Wait (ms)(milliseconds to wait=w2528) -> ()  [unwired: 1 out]
                  }
                  frame #6 {
                    n1549 = VISA Write(VISA resource name=w2535, write buffer=w2533, error in (no error)=w2532) -> (VISA resource name out=w2534:refnum<visa-resource-name>, error out=w2531:errorcluster)  [unwired: 1 out]
                  }
                  frame #7 {
                    n1550 = Wait (ms)(milliseconds to wait=w2536) -> ()  [unwired: 1 out]
                  }
                  frame #8 {
                    n1551 = Concatenate Strings("start ", "\r") -> (w2543:string)
                    n1552 = VISA Write(VISA resource name=w2545, write buffer=w2543, error in (no error)=w2544) -> (VISA resource name out=w2540:refnum<visa-resource-name>, error out=w2539:errorcluster)  [unwired: 1 out]
                  }
                  frame #9 {
                    n1553 = Wait (ms)(milliseconds to wait=w2546) -> ()  [unwired: 1 out]
                  }
                  frame #10 {
                    n1554 = Concatenate Strings("enter main ", "\r") -> (w2553:string)
                    n1555 = VISA Write(VISA resource name=w2552, write buffer=w2553, error in (no error)=w2551) -> (VISA resource name out=w2550:refnum<visa-resource-name>, error out=w2549:errorcluster)  [unwired: 1 out]
                    n1556 = VISA Close(VISA resource name=w2550, error in (no error)=w2549) -> ()  [unwired: 1 out]
                  }
                }
                n1557 = local read "Normal \nRate (ul/hr)  2"() -> (w2471:dbl)
                n1558 = Concatenate Strings("set units 4 ", w2486) -> (w2482:string)
                n1559 = local read "Normal \nVolume (ul) 2"() -> (w2472:dbl)
                n1560 = Number To Decimal String(number=w2471) -> (decimal integer string=w2481:string)  [unwired: 1 in]
                n1561 = Concatenate Strings("set rate ", w2481, w2486) -> (w2479:string)
                n1562 = Number To Decimal String(number=w2472) -> (decimal integer string=w2477:string)  [unwired: 1 in]
                n1563 = Concatenate Strings("set volume ", w2477, w2486) -> (w2476:string)
              }
            }
          }
          event "Inject Pump 1": Value Change {
            n1564 = event-data() -> ()  [unwired: 1 in, 5 out]
            n1565 = case shown="True" "Inject Pump 1" {
              tunnel: w2556 -> [w2559 w2601]
              frame False {
                n1566 = local read "Write Wait"() -> (w2558:i32)
                n1567 = call-poly "VISA Configure Serial Port"("VISA resource name"=w2559) -> ("VISA resource name out"=w2563:refnum<visa-resource-name>, "error out"=w2564:errorcluster)  [unwired: 13 in]
                n1568 = Concatenate Strings("enter pump1", "\r") -> (w2561:string)
                n1569 = flat-sequence {
                  tunnel: w2564 -> [w2575]
                  tunnel: w2563 -> [w2577]
                  tunnel: [w2576] -> w2572
                  tunnel: [w2574] -> w2571
                  tunnel: w2561 -> [w2573]
                  tunnel: w2572 -> [w2580]
                  tunnel: w2571 -> [w2579]
                  tunnel: [w2580] -> w2570
                  tunnel: [w2579] -> w2569
                  tunnel: w2558 -> [w2578]
                  tunnel: [w2584] -> w2568
                  tunnel: [w2583] -> w2567
                  tunnel: w2570 -> [w2582]
                  tunnel: w2569 -> [w2581]
                  tunnel: w2568 -> [w2590]
                  tunnel: [w2590] -> w2566
                  tunnel: w2567 -> [w2589]
                  tunnel: [w2589] -> w2565
                  tunnel: w2558 -> [w2588]
                  tunnel: w2566 -> [w2594]
                  tunnel: w2565 -> [w2593]
                  frame #0 {
                    n1570 = VISA Write(VISA resource name=w2577, write buffer=w2573, error in (no error)=w2575) -> (VISA resource name out=w2576:refnum<visa-resource-name>, error out=w2574:errorcluster)  [unwired: 1 out]
                  }
                  frame #1 {
                    n1571 = Wait (ms)(milliseconds to wait=w2578) -> ()  [unwired: 1 out]
                  }
                  frame #2 {
                    n1572 = Concatenate Strings("stop ", "\r") -> (w2587:string)
                    n1573 = VISA Write(VISA resource name=w2582, write buffer=w2587, error in (no error)=w2581) -> (VISA resource name out=w2584:refnum<visa-resource-name>, error out=w2583:errorcluster)  [unwired: 1 out]
                  }
                  frame #3 {
                    n1574 = Wait (ms)(milliseconds to wait=w2588) -> ()  [unwired: 1 out]
                  }
                  frame #4 {
                    n1575 = Concatenate Strings("enter main ", "\r") -> (w2595:string)
                    n1576 = VISA Write(VISA resource name=w2594, write buffer=w2595, error in (no error)=w2593) -> (VISA resource name out=w2592:refnum<visa-resource-name>, error out=w2591:errorcluster)  [unwired: 1 out]
                    n1577 = VISA Close(VISA resource name=w2592, error in (no error)=w2591) -> ()  [unwired: 1 out]
                  }
                }
              }
              frame True {
                w2614 = "\r"
                n1578 = call-poly "VISA Configure Serial Port"("VISA resource name"=w2601) -> ("VISA resource name out"=w2603:refnum<visa-resource-name>, "error out"=w2602:errorcluster)  [unwired: 13 in]
                n1579 = local read "Write Wait"() -> (w2598:i32)
                n1580 = flat-sequence {
                  tunnel: w2602 -> [w2637]
                  tunnel: w2603 -> [w2639]
                  tunnel: [w2638] -> w2634
                  tunnel: [w2636] -> w2633
                  tunnel: w2613 -> [w2635]
                  tunnel: w2634 -> [w2642]
                  tunnel: [w2642] -> w2632
                  tunnel: w2633 -> [w2641]
                  tunnel: [w2641] -> w2631
                  tunnel: w2598 -> [w2640]
                  tunnel: [w2647] -> w2630
                  tunnel: w2610 -> [w2646]
                  tunnel: [w2643] -> w2629
                  tunnel: w2632 -> [w2645]
                  tunnel: w2631 -> [w2644]
                  tunnel: w2630 -> [w2650]
                  tunnel: [w2650] -> w2628
                  tunnel: [w2649] -> w2627
                  tunnel: w2629 -> [w2649]
                  tunnel: w2598 -> [w2648]
                  tunnel: w2628 -> [w2655]
                  tunnel: [w2654] -> w2626
                  tunnel: w2607 -> [w2653]
                  tunnel: w2627 -> [w2652]
                  tunnel: [w2651] -> w2625
                  tunnel: w2626 -> [w2658]
                  tunnel: [w2658] -> w2624
                  tunnel: [w2657] -> w2623
                  tunnel: w2625 -> [w2657]
                  tunnel: w2598 -> [w2656]
                  tunnel: w2624 -> [w2663]
                  tunnel: [w2662] -> w2622
                  tunnel: w2604 -> [w2661]
                  tunnel: w2623 -> [w2660]
                  tunnel: [w2659] -> w2621
                  tunnel: [w2666] -> w2620
                  tunnel: w2622 -> [w2666]
                  tunnel: [w2665] -> w2619
                  tunnel: w2621 -> [w2665]
                  tunnel: w2598 -> [w2664]
                  tunnel: w2620 -> [w2673]
                  tunnel: w2619 -> [w2672]
                  tunnel: [w2668] -> w2618
                  tunnel: [w2667] -> w2617
                  tunnel: w2618 -> [w2676]
                  tunnel: [w2676] -> w2616
                  tunnel: w2617 -> [w2675]
                  tunnel: [w2675] -> w2615
                  tunnel: w2598 -> [w2674]
                  tunnel: w2616 -> [w2680]
                  tunnel: w2615 -> [w2679]
                  frame #0 {
                    n1581 = VISA Write(VISA resource name=w2639, write buffer=w2635, error in (no error)=w2637) -> (VISA resource name out=w2638:refnum<visa-resource-name>, error out=w2636:errorcluster)  [unwired: 1 out]
                  }
                  frame #1 {
                    n1582 = Wait (ms)(milliseconds to wait=w2640) -> ()  [unwired: 1 out]
                  }
                  frame #2 {
                    n1583 = VISA Write(VISA resource name=w2645, write buffer=w2646, error in (no error)=w2644) -> (VISA resource name out=w2647:refnum<visa-resource-name>, error out=w2643:errorcluster)  [unwired: 1 out]
                  }
                  frame #3 {
                    n1584 = Wait (ms)(milliseconds to wait=w2648) -> ()  [unwired: 1 out]
                  }
                  frame #4 {
                    n1585 = VISA Write(VISA resource name=w2655, write buffer=w2653, error in (no error)=w2652) -> (VISA resource name out=w2654:refnum<visa-resource-name>, error out=w2651:errorcluster)  [unwired: 1 out]
                  }
                  frame #5 {
                    n1586 = Wait (ms)(milliseconds to wait=w2656) -> ()  [unwired: 1 out]
                  }
                  frame #6 {
                    n1587 = VISA Write(VISA resource name=w2663, write buffer=w2661, error in (no error)=w2660) -> (VISA resource name out=w2662:refnum<visa-resource-name>, error out=w2659:errorcluster)  [unwired: 1 out]
                  }
                  frame #7 {
                    n1588 = Wait (ms)(milliseconds to wait=w2664) -> ()  [unwired: 1 out]
                  }
                  frame #8 {
                    n1589 = Concatenate Strings("start ", "\r") -> (w2671:string)
                    n1590 = VISA Write(VISA resource name=w2673, write buffer=w2671, error in (no error)=w2672) -> (VISA resource name out=w2668:refnum<visa-resource-name>, error out=w2667:errorcluster)  [unwired: 1 out]
                  }
                  frame #9 {
                    n1591 = Wait (ms)(milliseconds to wait=w2674) -> ()  [unwired: 1 out]
                  }
                  frame #10 {
                    n1592 = Concatenate Strings("enter main ", "\r") -> (w2681:string)
                    n1593 = VISA Write(VISA resource name=w2680, write buffer=w2681, error in (no error)=w2679) -> (VISA resource name out=w2678:refnum<visa-resource-name>, error out=w2677:errorcluster)  [unwired: 1 out]
                    n1594 = VISA Close(VISA resource name=w2678, error in (no error)=w2677) -> ()  [unwired: 1 out]
                  }
                }
                n1595 = Concatenate Strings("enter pump1", w2614) -> (w2613:string)
                n1596 = local read "Normal \nRate (ul/hr)"() -> (w2599:dbl)
                n1597 = Concatenate Strings("set units 4 ", w2614) -> (w2610:string)
                n1598 = local read "Normal \nVolume (ul)"() -> (w2600:dbl)
                n1599 = Number To Decimal String(number=w2599) -> (decimal integer string=w2609:string)  [unwired: 1 in]
                n1600 = Concatenate Strings("set rate ", w2609, w2614) -> (w2607:string)
                n1601 = Number To Decimal String(number=w2600) -> (decimal integer string=w2605:string)  [unwired: 1 in]
                n1602 = Concatenate Strings("set volume ", w2605, w2614) -> (w2604:string)
              }
            }
          }
          event "Normal \nVolume (ul)": Value Change {
            n1603 = event-data() -> ()  [unwired: 1 in, 5 out]
            n1604 = call-poly "VISA Configure Serial Port"("VISA resource name"=w2699) -> ("VISA resource name out"=w2701:refnum<visa-resource-name>, "error out"=w2700:errorcluster)  [unwired: 13 in]
            n1605 = local read "Write Wait"() -> (w2684:i32)
            n1606 = Concatenate Strings("enter pump1", "\r") -> (w2703:string)
            n1607 = flat-sequence {
              tunnel: w2700 -> [w2713]
              tunnel: w2701 -> [w2715]
              tunnel: [w2714] -> w2693
              tunnel: [w2712] -> w2692
              tunnel: w2703 -> [w2711]
              tunnel: w2693 -> [w2718]
              tunnel: [w2718] -> w2691
              tunnel: w2692 -> [w2717]
              tunnel: [w2717] -> w2689
              tunnel: w2684 -> [w2716]
              tunnel: w2691 -> [w2722]
              tunnel: [w2723] -> w2690
              tunnel: w2689 -> [w2721]
              tunnel: [w2720] -> w2688
              tunnel: w2685 -> [w2719]
              tunnel: w2690 -> [w2726]
              tunnel: w2688 -> [w2725]
              tunnel: [w2726] -> w2710
              tunnel: [w2725] -> w2709
              tunnel: w2684 -> [w2724]
              tunnel: [w2731] -> w2708
              tunnel: [w2730] -> w2707
              tunnel: w2710 -> [w2729]
              tunnel: w2709 -> [w2728]
              tunnel: w2694 -> [w2727]
              tunnel: w2708 -> [w2734]
              tunnel: [w2734] -> w2706
              tunnel: w2707 -> [w2733]
              tunnel: [w2733] -> w2705
              tunnel: w2684 -> [w2732]
              tunnel: w2706 -> [w2738]
              tunnel: w2705 -> [w2737]
              frame #0 {
                n1608 = VISA Write(VISA resource name=w2715, write buffer=w2711, error in (no error)=w2713) -> (VISA resource name out=w2714:refnum<visa-resource-name>, error out=w2712:errorcluster)  [unwired: 1 out]
              }
              frame #1 {
                n1609 = Wait (ms)(milliseconds to wait=w2716) -> ()  [unwired: 1 out]
              }
              frame #2 {
                n1610 = VISA Write(VISA resource name=w2722, write buffer=w2719, error in (no error)=w2721) -> (VISA resource name out=w2723:refnum<visa-resource-name>, error out=w2720:errorcluster)  [unwired: 1 out]
              }
              frame #3 {
                n1611 = Wait (ms)(milliseconds to wait=w2724) -> ()  [unwired: 1 out]
              }
              frame #4 {
                n1612 = VISA Write(VISA resource name=w2729, write buffer=w2727, error in (no error)=w2728) -> (VISA resource name out=w2731:refnum<visa-resource-name>, error out=w2730:errorcluster)  [unwired: 1 out]
              }
              frame #5 {
                n1613 = Wait (ms)(milliseconds to wait=w2732) -> ()  [unwired: 1 out]
              }
              frame #6 {
                n1614 = Concatenate Strings("enter main ", "\r") -> (w2739:string)
                n1615 = VISA Write(VISA resource name=w2738, write buffer=w2739, error in (no error)=w2737) -> (VISA resource name out=w2736:refnum<visa-resource-name>, error out=w2735:errorcluster)  [unwired: 1 out]
                n1616 = VISA Close(VISA resource name=w2736, error in (no error)=w2735) -> ()  [unwired: 1 out]
              }
            }
            n1617 = Concatenate Strings("set units 4", "\r") -> (w2685:string)
            n1618 = Number To Decimal String(number="Normal \nVolume (ul)") -> (decimal integer string=w2696:string)  [unwired: 1 in]
            n1619 = Concatenate Strings("set volume", w2696, "\r") -> (w2694:string)
          }
          event "Normal \nRate (ul/hr)": Value Change {
            n1620 = event-data() -> ()  [unwired: 1 in, 5 out]
            n1621 = call-poly "VISA Configure Serial Port"("VISA resource name"=w2744) -> ("VISA resource name out"=w2752:refnum<visa-resource-name>, "error out"=w2751:errorcluster)  [unwired: 13 in]
            n1622 = local read "Write Wait"() -> (w2742:i32)
            n1623 = Concatenate Strings("enter pump1", "\r") -> (w2754:string)
            n1624 = flat-sequence {
              tunnel: w2751 -> [w2771]
              tunnel: w2752 -> [w2773]
              tunnel: [w2772] -> w2767
              tunnel: [w2770] -> w2766
              tunnel: w2754 -> [w2769]
              tunnel: w2767 -> [w2776]
              tunnel: [w2776] -> w2765
              tunnel: w2766 -> [w2775]
              tunnel: [w2775] -> w2764
              tunnel: w2742 -> [w2774]
              tunnel: w2765 -> [w2780]
              tunnel: [w2781] -> w2763
              tunnel: w2764 -> [w2779]
              tunnel: [w2778] -> w2762
              tunnel: w2745 -> [w2777]
              tunnel: w2763 -> [w2784]
              tunnel: w2762 -> [w2783]
              tunnel: [w2784] -> w2761
              tunnel: [w2783] -> w2760
              tunnel: w2742 -> [w2782]
              tunnel: [w2789] -> w2759
              tunnel: [w2788] -> w2758
              tunnel: w2761 -> [w2787]
              tunnel: w2760 -> [w2786]
              tunnel: w2748 -> [w2785]
              tunnel: w2759 -> [w2792]
              tunnel: [w2792] -> w2757
              tunnel: w2758 -> [w2791]
              tunnel: [w2791] -> w2756
              tunnel: w2742 -> [w2790]
              tunnel: w2757 -> [w2796]
              tunnel: w2756 -> [w2795]
              frame #0 {
                n1625 = VISA Write(VISA resource name=w2773, write buffer=w2769, error in (no error)=w2771) -> (VISA resource name out=w2772:refnum<visa-resource-name>, error out=w2770:errorcluster)  [unwired: 1 out]
              }
              frame #1 {
                n1626 = Wait (ms)(milliseconds to wait=w2774) -> ()  [unwired: 1 out]
              }
              frame #2 {
                n1627 = VISA Write(VISA resource name=w2780, write buffer=w2777, error in (no error)=w2779) -> (VISA resource name out=w2781:refnum<visa-resource-name>, error out=w2778:errorcluster)  [unwired: 1 out]
              }
              frame #3 {
                n1628 = Wait (ms)(milliseconds to wait=w2782) -> ()  [unwired: 1 out]
              }
              frame #4 {
                n1629 = VISA Write(VISA resource name=w2787, write buffer=w2785, error in (no error)=w2786) -> (VISA resource name out=w2789:refnum<visa-resource-name>, error out=w2788:errorcluster)  [unwired: 1 out]
              }
              frame #5 {
                n1630 = Wait (ms)(milliseconds to wait=w2790) -> ()  [unwired: 1 out]
              }
              frame #6 {
                n1631 = Concatenate Strings("enter main ", "\r") -> (w2797:string)
                n1632 = VISA Write(VISA resource name=w2796, write buffer=w2797, error in (no error)=w2795) -> (VISA resource name out=w2794:refnum<visa-resource-name>, error out=w2793:errorcluster)  [unwired: 1 out]
                n1633 = VISA Close(VISA resource name=w2794, error in (no error)=w2793) -> ()  [unwired: 1 out]
              }
            }
            n1634 = Concatenate Strings("set units 4", "\r") -> (w2745:string)
            n1635 = Number To Decimal String(number="Normal \nRate (ul/hr)") -> (decimal integer string=w2743:string)  [unwired: 1 in]
            n1636 = Concatenate Strings("set rate", w2743, "\r") -> (w2748:string)
          }
          event "Normal \nRate (ul/hr)  2": Value Change {
            n1637 = event-data() -> ()  [unwired: 1 in, 5 out]
            n1638 = call-poly "VISA Configure Serial Port"("VISA resource name"=w2802) -> ("VISA resource name out"=w2810:refnum<visa-resource-name>, "error out"=w2809:errorcluster)  [unwired: 13 in]
            n1639 = local read "Write Wait"() -> (w2800:i32)
            n1640 = Concatenate Strings("enter pump2", "\r") -> (w2812:string)
            n1641 = flat-sequence {
              tunnel: w2809 -> [w2829]
              tunnel: w2810 -> [w2831]
              tunnel: [w2830] -> w2825
              tunnel: [w2828] -> w2824
              tunnel: w2812 -> [w2827]
              tunnel: w2825 -> [w2834]
              tunnel: [w2834] -> w2823
              tunnel: w2824 -> [w2833]
              tunnel: [w2833] -> w2822
              tunnel: w2800 -> [w2832]
              tunnel: w2823 -> [w2838]
              tunnel: [w2839] -> w2821
              tunnel: w2822 -> [w2837]
              tunnel: [w2836] -> w2820
              tunnel: w2803 -> [w2835]
              tunnel: w2821 -> [w2842]
              tunnel: w2820 -> [w2841]
              tunnel: [w2842] -> w2819
              tunnel: [w2841] -> w2818
              tunnel: w2800 -> [w2840]
              tunnel: [w2847] -> w2817
              tunnel: [w2846] -> w2816
              tunnel: w2819 -> [w2845]
              tunnel: w2818 -> [w2844]
              tunnel: w2806 -> [w2843]
              tunnel: w2817 -> [w2850]
              tunnel: [w2850] -> w2815
              tunnel: w2816 -> [w2849]
              tunnel: [w2849] -> w2814
              tunnel: w2800 -> [w2848]
              tunnel: w2815 -> [w2854]
              tunnel: w2814 -> [w2853]
              frame #0 {
                n1642 = VISA Write(VISA resource name=w2831, write buffer=w2827, error in (no error)=w2829) -> (VISA resource name out=w2830:refnum<visa-resource-name>, error out=w2828:errorcluster)  [unwired: 1 out]
              }
              frame #1 {
                n1643 = Wait (ms)(milliseconds to wait=w2832) -> ()  [unwired: 1 out]
              }
              frame #2 {
                n1644 = VISA Write(VISA resource name=w2838, write buffer=w2835, error in (no error)=w2837) -> (VISA resource name out=w2839:refnum<visa-resource-name>, error out=w2836:errorcluster)  [unwired: 1 out]
              }
              frame #3 {
                n1645 = Wait (ms)(milliseconds to wait=w2840) -> ()  [unwired: 1 out]
              }
              frame #4 {
                n1646 = VISA Write(VISA resource name=w2845, write buffer=w2843, error in (no error)=w2844) -> (VISA resource name out=w2847:refnum<visa-resource-name>, error out=w2846:errorcluster)  [unwired: 1 out]
              }
              frame #5 {
                n1647 = Wait (ms)(milliseconds to wait=w2848) -> ()  [unwired: 1 out]
              }
              frame #6 {
                n1648 = Concatenate Strings("enter main ", "\r") -> (w2855:string)
                n1649 = VISA Write(VISA resource name=w2854, write buffer=w2855, error in (no error)=w2853) -> (VISA resource name out=w2852:refnum<visa-resource-name>, error out=w2851:errorcluster)  [unwired: 1 out]
                n1650 = VISA Close(VISA resource name=w2852, error in (no error)=w2851) -> ()  [unwired: 1 out]
              }
            }
            n1651 = Concatenate Strings("set units 4", "\r") -> (w2803:string)
            n1652 = Number To Decimal String(number="Normal \nRate (ul/hr)  2") -> (decimal integer string=w2801:string)  [unwired: 1 in]
            n1653 = Concatenate Strings("set rate", w2801, "\r") -> (w2806:string)
          }
          event "Normal \nVolume (ul) 2": Value Change {
            n1654 = event-data() -> ()  [unwired: 1 in, 5 out]
            n1655 = call-poly "VISA Configure Serial Port"("VISA resource name"=w2861) -> ("VISA resource name out"=w2865:refnum<visa-resource-name>, "error out"=w2866:errorcluster)  [unwired: 13 in]
            n1656 = local read "Write Wait"() -> (w2858:i32)
            n1657 = Concatenate Strings("enter pump2", "\r") -> (w2863:string)
            n1658 = flat-sequence {
              tunnel: w2866 -> [w2887]
              tunnel: w2865 -> [w2889]
              tunnel: [w2888] -> w2884
              tunnel: [w2886] -> w2883
              tunnel: w2863 -> [w2885]
              tunnel: w2884 -> [w2892]
              tunnel: [w2892] -> w2882
              tunnel: w2883 -> [w2891]
              tunnel: [w2891] -> w2881
              tunnel: w2858 -> [w2890]
              tunnel: w2882 -> [w2896]
              tunnel: [w2897] -> w2880
              tunnel: w2881 -> [w2895]
              tunnel: [w2894] -> w2879
              tunnel: w2872 -> [w2893]
              tunnel: w2880 -> [w2900]
              tunnel: w2879 -> [w2899]
              tunnel: [w2900] -> w2878
              tunnel: [w2899] -> w2877
              tunnel: w2858 -> [w2898]
              tunnel: [w2905] -> w2876
              tunnel: [w2904] -> w2875
              tunnel: w2878 -> [w2903]
              tunnel: w2877 -> [w2902]
              tunnel: w2869 -> [w2901]
              tunnel: w2876 -> [w2908]
              tunnel: [w2908] -> w2874
              tunnel: w2875 -> [w2907]
              tunnel: [w2907] -> w2873
              tunnel: w2858 -> [w2906]
              tunnel: w2874 -> [w2912]
              tunnel: w2873 -> [w2911]
              frame #0 {
                n1659 = VISA Write(VISA resource name=w2889, write buffer=w2885, error in (no error)=w2887) -> (VISA resource name out=w2888:refnum<visa-resource-name>, error out=w2886:errorcluster)  [unwired: 1 out]
              }
              frame #1 {
                n1660 = Wait (ms)(milliseconds to wait=w2890) -> ()  [unwired: 1 out]
              }
              frame #2 {
                n1661 = VISA Write(VISA resource name=w2896, write buffer=w2893, error in (no error)=w2895) -> (VISA resource name out=w2897:refnum<visa-resource-name>, error out=w2894:errorcluster)  [unwired: 1 out]
              }
              frame #3 {
                n1662 = Wait (ms)(milliseconds to wait=w2898) -> ()  [unwired: 1 out]
              }
              frame #4 {
                n1663 = VISA Write(VISA resource name=w2903, write buffer=w2901, error in (no error)=w2902) -> (VISA resource name out=w2905:refnum<visa-resource-name>, error out=w2904:errorcluster)  [unwired: 1 out]
              }
              frame #5 {
                n1664 = Wait (ms)(milliseconds to wait=w2906) -> ()  [unwired: 1 out]
              }
              frame #6 {
                n1665 = Concatenate Strings("enter main ", "\r") -> (w2913:string)
                n1666 = VISA Write(VISA resource name=w2912, write buffer=w2913, error in (no error)=w2911) -> (VISA resource name out=w2910:refnum<visa-resource-name>, error out=w2909:errorcluster)  [unwired: 1 out]
                n1667 = VISA Close(VISA resource name=w2910, error in (no error)=w2909) -> ()  [unwired: 1 out]
              }
            }
            n1668 = Concatenate Strings("set units 4", "\r") -> (w2872:string)
            n1669 = Number To Decimal String(number="Normal \nVolume (ul) 2") -> (decimal integer string=w2859:string)  [unwired: 1 in]
            n1670 = Concatenate Strings("set volume", w2859, "\r") -> (w2869:string)
          }
        }
        n1671 = node-c288() -> ()  [unwired: 1 in, 1 out]
      }
      n1672 = node-c288(w2245) -> ()  [unwired: 1 out]
    }
    frame Enabled {
      n1673 = node-c288(2 ("Processor")) -> (w2925:T13)  [unwired: 3 in]
      n1674 = timed-loop "Pump Control" {
        timing: w2925 -> [_]
        timing-out: [_] -> w2924
        tunnel: refnum<visa-resource-name> "COM4" ("VISA resource name") -> [w2927]
        stop <- w2926 stop-if-true
        n1675 = node-c288() -> ()  [unwired: 1 in, 1 out]
        n1676 = event shown="[2] \"Inject Sample\": Value Change" {
          selector: _ -> [_ _ _ _ _]
          dyn-events: _ -> [_ _ _ _ _]
          timeout: _ -> [_ _ _ _ _]
          tunnel: w2927 -> [w2933 _ w3007 w3034 w3039]
          tunnel: [_ w3005 _ _ _] -> w2926
          event "Flush Sample": Value Change {
            n1677 = event-data() -> ()  [unwired: 1 in, 5 out]
            n1678 = local read "Write Wait"() -> (w2947:i32)
            n1679 = flat-sequence {
              tunnel: [w2971] -> w2967
              tunnel: [w2970] -> w2966
              tunnel: "CLD" -> [w2969]
              tunnel: w2933 -> [w2968]
              tunnel: w2967 -> [w2974]
              tunnel: [w2974] -> w2965
              tunnel: w2966 -> [w2973]
              tunnel: [w2973] -> w2964
              tunnel: w2947 -> [w2972]
              tunnel: [w2979] -> w2963
              tunnel: [w2976] -> w2962
              tunnel: w2965 -> [w2978]
              tunnel: w2964 -> [w2977]
              tunnel: "MODVOL" -> [w2975]
              tunnel: w2963 -> [w2982]
              tunnel: [w2982] -> w2961
              tunnel: [w2981] -> w2960
              tunnel: w2962 -> [w2981]
              tunnel: w2947 -> [w2980]
              tunnel: w2961 -> [w2987]
              tunnel: [w2986] -> w2959
              tunnel: w2949 -> [w2985]
              tunnel: w2960 -> [w2984]
              tunnel: [w2983] -> w2958
              tunnel: w2959 -> [w2990]
              tunnel: [w2990] -> w2957
              tunnel: [w2989] -> w2956
              tunnel: w2958 -> [w2989]
              tunnel: w2947 -> [w2988]
              tunnel: w2957 -> [w2995]
              tunnel: [w2994] -> w2955
              tunnel: w2951 -> [w2993]
              tunnel: w2956 -> [w2992]
              tunnel: [w2991] -> w2954
              tunnel: [w2998] -> w2952
              tunnel: w2955 -> [w2998]
              tunnel: [w2997] -> w2953
              tunnel: w2954 -> [w2997]
              tunnel: w2947 -> [w2996]
              tunnel: w2953 -> [w3003]
              tunnel: w2952 -> [w3004]
              tunnel: [w3002] -> w2942
              tunnel: "RUN " -> [w3001]
              frame #0 {
                n1680 = call "Write to pump 2.vi"("String to write"=w2969, "VISA resource name"=w2968) -> ("error out"=w2970:errorcluster, "VISA resource name out"=w2971:refnum<visa-resource-name>)  [unwired: 8 in]
              }
              frame #1 {
                n1681 = Wait (ms)(milliseconds to wait=w2972) -> ()  [unwired: 1 out]
              }
              frame #2 {
                n1682 = call "Write to pump 2.vi"("error in (no error)"=w2977, "String to write"=w2975, "VISA resource name"=w2978) -> ("error out"=w2976:errorcluster, "VISA resource name out"=w2979:refnum<visa-resource-name>)  [unwired: 7 in]
              }
              frame #3 {
                n1683 = Wait (ms)(milliseconds to wait=w2980) -> ()  [unwired: 1 out]
              }
              frame #4 {
                n1684 = call "Write to pump 2.vi"("error in (no error)"=w2984, "String to write"=w2985, "VISA resource name"=w2987) -> ("error out"=w2983:errorcluster, "VISA resource name out"=w2986:refnum<visa-resource-name>)  [unwired: 7 in]
              }
              frame #5 {
                n1685 = Wait (ms)(milliseconds to wait=w2988) -> ()  [unwired: 1 out]
              }
              frame #6 {
                n1686 = call "Write to pump 2.vi"("error in (no error)"=w2992, "String to write"=w2993, "VISA resource name"=w2995) -> ("error out"=w2991:errorcluster, "VISA resource name out"=w2994:refnum<visa-resource-name>)  [unwired: 7 in]
              }
              frame #7 {
                n1687 = Wait (ms)(milliseconds to wait=w2996) -> ()  [unwired: 1 out]
              }
              frame #8 {
                w3000 = TRUE ("Inject Pump 3")
                n1688 = Tick Count (ms)() -> (millisecond timer value=→"Flush Sample Start Time":u32)
                n1689 = call "Write to pump 2.vi"("error in (no error)"=w3003, "String to write"=w3001, "VISA resource name"=w3004) -> ("error out"=w3002:errorcluster)  [unwired: 7 in, 1 out]
                n1690 = local write "Inject Sample"(w3000) -> ()
                "Flushing Sample" <- w3000
              }
            }
            n1691 = Number To Fractional String(number="Flush \nRate (ul/min)  3") -> (F-format string=w2935:string)  [unwired: 3 in]
            n1692 = String Subset(string=w2935, length (rest)=6 ("length (rest)")) -> (substring=w2934:string)  [unwired: 1 in]
            n1693 = Concatenate Strings("RAT", w2934, "UM") -> (w2949:string)
            n1694 = Divide(x="Flush\nVolume (ul)  3", y=1000.0) -> (x/y=w2940:dbl)
            n1695 = Number To Fractional String(number=w2940) -> (F-format string=w2939:string)  [unwired: 3 in]
            n1696 = Divide(x="Flush\nVolume (ul)  3", y="Flush \nRate (ul/min)  3") -> (x/y=w2930:dbl)
            n1697 = Multiply(x=w2930, y=60.0) -> (x*y=→"Sample flush time (s)":dbl)
            n1698 = String Subset(string=w2939, length (rest)=6 ("length (rest)")) -> (substring=w2938:string)  [unwired: 1 in]
            n1699 = Concatenate Strings("TGT", w2938) -> (w2951:string)
            "error out" <- w2942
          }
          event "Stop": Value Change {
            n1700 = event-data() -> ()  [unwired: 1 in, 5 out]
            n1701 = local read "Stop"() -> (w3005:bool)
          }
          event "Inject Sample": Value Change {
            n1702 = event-data() -> ()  [unwired: 1 in, 5 out]
            n1703 = case shown="True" "Inject Sample" {
              tunnel: w3007 -> [w3009 w3010]
              frame False {
                n1704 = call "Write to pump 2.vi"("String to write"="STP", "VISA resource name"=w3009) -> ()  [unwired: 8 in, 2 out]
              }
              frame True {
                n1705 = local read "Normal \nRate (ul/hr)  3"() -> (w3011:dbl)
                n1706 = Number To Fractional String(number=w3011) -> (F-format string=w3014:string)  [unwired: 3 in]
                n1707 = String Subset(string=w3014, length (rest)=6 ("length (rest)")) -> (substring=w3012:string)  [unwired: 1 in]
                n1708 = flat-sequence {
                  tunnel: "RUN " -> [w3026]
                  tunnel: [w3028] -> _
                  tunnel: [w3027] -> _
                  tunnel: w3010 -> [w3025]
                  frame #0 {
                    n1709 = call "Write to pump 2.vi"("String to write"=w3026, "VISA resource name"=w3025) -> ("error out"=w3027:errorcluster, "VISA resource name out"=w3028:refnum<visa-resource-name>)  [unwired: 8 in]
                  }
                }
                n1710 = Concatenate Strings("RAT", w3012, "UH" ("string")) -> ()  [unwired: 1 out]
                n1711 = local read "Normal \nVolume (ul) 3"() -> (w3020:dbl)
                n1712 = Divide(x=w3020, y=1000.0) -> (x/y=w3015:dbl)
                n1713 = Number To Fractional String(number=w3015) -> (F-format string=w3018:string)  [unwired: 3 in]
                n1714 = String Subset(string=w3018, length (rest)=6 ("length (rest)")) -> (substring=w3016:string)  [unwired: 1 in]
                n1715 = Concatenate Strings("TGT", w3016) -> ()  [unwired: 1 out]
              }
            }
          }
          event "Normal \nRate (ul/hr)  3": Value Change {
            n1716 = event-data() -> ()  [unwired: 1 in, 5 out]
            n1717 = Number To Fractional String(number="Normal \nRate (ul/hr)  3") -> (F-format string=w3032:string)  [unwired: 3 in]
            n1718 = String Subset(string=w3032, length (rest)=6 ("length (rest)")) -> (substring=w3030:string)  [unwired: 1 in]
            n1719 = Concatenate Strings("RAT", w3030, "UH") -> (w3033:string)
            n1720 = call "Write to pump 2.vi"("String to write"=w3033, "VISA resource name"=w3034) -> ()  [unwired: 8 in, 2 out]
          }
          event "Clear Volume": Value Change {
            n1721 = event-data() -> ()  [unwired: 1 in, 5 out]
            n1722 = Divide(x="Normal \nVolume (ul) 3", y=1000.0) -> (x/y=w3052:dbl)
            n1723 = Number To Fractional String(number=w3052) -> (F-format string=w3055:string)  [unwired: 3 in]
            n1724 = String Subset(string=w3055, length (rest)=6 ("length (rest)")) -> (substring=w3053:string)  [unwired: 1 in]
            n1725 = flat-sequence {
              tunnel: [w3062] -> w3050
              tunnel: [w3061] -> w3049
              tunnel: w3039 -> [w3060]
              tunnel: w3038 -> [w3059]
              tunnel: [w3064] -> w3047
              tunnel: [w3063] -> w3048
              tunnel: w3044 -> [w3065]
              tunnel: w3050 -> [w3064]
              tunnel: w3049 -> [w3063]
              tunnel: w3048 -> [w3069]
              tunnel: w3047 -> [w3070]
              tunnel: [w3068] -> _
              tunnel: [w3067] -> _
              tunnel: w3037 -> [w3066]
              frame #0 {
                n1726 = call "Write to pump 2.vi"("String to write"=w3059, "VISA resource name"=w3060) -> ("error out"=w3061:errorcluster, "VISA resource name out"=w3062:refnum<visa-resource-name>)  [unwired: 8 in]
              }
              frame #1 {
                n1727 = Wait (ms)(milliseconds to wait=w3065) -> ()  [unwired: 1 out]
              }
              frame #2 {
                n1728 = call "Write to pump 2.vi"("error in (no error)"=w3069, "String to write"=w3066, "VISA resource name"=w3070) -> ("error out"=w3067:errorcluster, "VISA resource name out"=w3068:refnum<visa-resource-name>)  [unwired: 7 in]
              }
            }
            n1729 = local read "Write Wait"() -> (w3044:i32)
            n1730 = Concatenate Strings("TGT", w3053) -> (w3038:string)
            n1731 = local read "Normal \nRate (ul/hr)  3"() -> (w3040:dbl)
            n1732 = local write "Clear Volume"(FALSE ("Clear Volume")) -> ()
            n1733 = Number To Fractional String(number=w3040) -> (F-format string=w3043:string)  [unwired: 3 in]
            n1734 = String Subset(string=w3043, length (rest)=6 ("length (rest)")) -> (substring=w3041:string)  [unwired: 1 in]
            n1735 = Concatenate Strings("RAT", w3041, "UH" ("string")) -> (w3037:string)
          }
        }
        n1736 = node-c288() -> ()  [unwired: 1 in, 1 out]
      }
      n1737 = node-c288(w2924) -> ()  [unwired: 1 out]
    }
  }
  n1738 = node-c288() -> (w90:T13)  [unwired: 4 in]
  n1739 = timed-loop {
    timing: w90 -> [_]
    timing-out: [_] -> w89
    stop <- w3077 stop-if-true
    n1740 = node-c288() -> ()  [unwired: 1 in, 1 out]
    n1741 = event shown="[1] \"Stop\": Value Change" {
      selector: _ -> [_ _]
      dyn-events: _ -> [_ _]
      timeout: _ -> [_ _]
      tunnel: [_ w3078] -> w3077
      event Timeout {
        n1742 = event-data() -> ()  [unwired: 1 in, 2 out]
      }
      event "Stop": Value Change {
        n1743 = event-data() -> ()  [unwired: 1 in, 4 out]
        n1744 = flat-sequence {
          tunnel: ["Stop"] -> w3078
          frame #0 {
            w3079 = FALSE ("Force Feedback")
            n1745 = local write "Force Feedback 1"(w3079) -> ()
            n1746 = local write "Force Feedback 2"(w3079) -> ()
            n1747 = property on="Cancel dwell" class="Bool (strict)"("Val(Sgnl)"=TRUE ("Value (Signaling)")) -> ()  [unwired: 2 in, 2 out]
          }
          frame #1 {
            w3081 = FALSE
            n1748 = local write "Raster scanning..."(w3081) -> ()
            n1749 = local write "Cancel dwell"(w3081) -> ()
            n1750 = local write "Stage moving"(w3081) -> ()
            n1751 = local write "Saving Move"(w3081) -> ()
          }
        }
      }
    }
    n1752 = node-c288() -> ()  [unwired: 1 in, 1 out]
  }
  n1753 = case shown="True" w80 {
    tunnel: w85 -> [_ w3087]
    tunnel: w84 -> [_ w3086]
    tunnel: w83 -> [_ w3085]
    frame False {
    }
    frame True {
      w3089 = T24 3 items=["no dialog", "OK message", "continue or stop message", "OK message + warnings", "continue/stop + warnings"] ("type of dialog (OK msg:1)")
      w3088 = T24 3 items=["no dialog", "OK message", "continue or stop message", "OK message + warnings", "continue/stop + warnings"] ("type of dialog (OK msg:1)")
      n1754 = call <vilib>:"DAQmx Clear Task.vi"("task in"=w3087, "error in"=w3085) -> ("error out"=w3090:errorcluster)  [unwired: 13 in]
      n1755 = call <vilib>:"DAQmx Clear Task.vi"("task in"=w3086) -> ("error out"=w3091:errorcluster)  [unwired: 14 in]
      n1756 = call <vilib>:"Simple Error Handler.vi"("type of dialog (OK msg:1)"=w3089, "error in (no error)"=w3090) -> ()  [unwired: 3 in, 5 out]
      n1757 = call <vilib>:"Simple Error Handler.vi"("type of dialog (OK msg:1)"=w3088, "error in (no error)"=w3091) -> ()  [unwired: 3 in, 5 out]
    }
  }
  n1758 = case shown="\"Raster scan\"" "?" {
    frame "Force Feedback", Default {
    }
    frame "Raster scan" {
    }
  }
  n1759 = node-c288(w89) -> ()  [unwired: 1 out]
  n1760 = node-c288(w92) -> ()  [unwired: 1 out]
  n1761 = local write "Pause Mouse/Mirror Connection"(FALSE ("Pause Mouse/Mirror Connection")) -> ()
  n1762 = local write "Stop"(FALSE ("Stop all")) -> ()
  "CoordinatesMousePressed" <- T5 {"Horizontal"=0, "Vertical"=0} ("Coords when pressed")
  "Deflection" <- T5 {"Horizontal"=0, "Vertical"=0} ("Coords when pressed")
